vi "MultirunBuilderForNamedLocations2.vi"() -> ()   [LabVIEW 2015]
uses:
  MultirunBuilderSubVIs/RowTemplate.ctl
  Anemometry Sub Vis/Gen Trav/Spacing.ctl
  Anemometry Sub Vis/Controls/Multi_run_mode.ctl
  MultirunBuilderSubVIs/MRBRowTaskSelector.ctl
  Anemometry Sub Vis/File/Setup_Filetype.ctl
  Anemometry Sub Vis/Controls/Tunnel_Coordinates.ctl
  Anemometry Sub Vis/Globals/Meas_global.vi
  MultirunBuilderSubVIs/MRCMDFBGlobal.vi
  MultirunBuilderSubVIs/Set Speed Only.vi
  MultirunBuilderSubVIs/Wait (minutes).vi
  MultirunBuilderSubVIs/Single Measurement.vi
  MultirunBuilderSubVIs/Auto Calibrate.vi
  MultirunBuilderSubVIs/MoveTT.vi
panel:
  in  "Vert.Z-Locations 2":dbl[](array[numeric])=[12.7, 19.05, 25.4]
  in  "TaskArray":T3(array[cluster])=[{"Start X"=0.0, "Start Y"=0.0, "Start Z"=0.0, "End X"=0.0, "End Y"=0.0, "End Z"=0.0, "No. of pts."=0, "Spacing"=enum."Linear", "Filename"=path "M:/\\Projects\\8773\\Results\\Tunnel1\\AnemometerSurvey.xls", "Tunnel Speed"=7.64, "Averaging time (min)"=0.0, "Extra Commands"="", "Carrier_1 Q (l/min)"=0.0, "Carrier_2 Q (l/min)"=0.0, "Trace Gas Concentration (%)"=0.0, "Specific Arguments"="", "Comments"="Tunnel Warm Up", "Row No"=0, "Row Type Selector"=enum."Set Tunnel Speed Only", "Completion time"="", "Row Duration (mins)"=0.0, "No. of Valid pts."=0, "Meas Setup File"="Current_Setup.xls"}, {"Start X"=0.0, "Start Y"=0.0, "Start Z"=0.0, "End X"=0.0, "End Y"=0.0, "End Z"=0.0, "No. of pts."=0, "Spacing"=enum."Linear", "Filename"=path "M:/\\Projects\\8773\\Results\\Tunnel1\\AnemometerSurvey.xls", "Tunnel Speed"=0.0, "Averaging time (min)"=0.0, "Extra Commands"="", "Carrier_1 Q (l/min)"=0.0, "Carrier_2 Q (l/min)"=0.0, "Trace Gas Concentration (%)"=0.0, "Specific Arguments"="10.00", "Comments"="Tunnel Warm Up", "Row No"=0, "Row Type Selector"=enum."Wait (minutes)", "Completion time"="", "Row Duration (mins)"=0.0, "No. of Valid pts."=0, "Meas Setup File"="Current_Setup.xls"}, {"Start X"=-3390.0, "Start Y"=-113.0, "Start Z"=780.0, "End X"=-3390.0, "End Y"=-113.0, "End Z"=780.0, "No. of pts."=0, "Spacing"=enum."Linear", "Filename"=path "M:/\\Projects\\8773\\Results\\Tunnel1\\AnemometerSurvey.xls", "Tunnel Speed"=0.0, "Averaging time (min)"=1.0, "Extra Commands"="!Work in Tunnel Coordinates", "Carrier_1 Q (l/min)"=0.0, "Carrier_2 Q (l/min)"=0.0, "Trace Gas Concentration (%)"=0.0, "Specific Arguments"="", "Comments"="Zeroes", "Row No"=0, "Row Type Selector"=enum."Single Measurement", "Completion time"="", "Row Duration (mins)"=0.0, "No. of Valid pts."=0, "Meas Setup File"="Current_Setup.xls"}, {"Start X"=-3390.0, "Start Y"=-113.0, "Start Z"=780.0, "End X"=-3390.0, "End Y"=-113.0, "End Z"=780.0, "No. of pts."=0, "Spacing"=enum."Linear", "Filename"=path "M:/\\Projects\\8773\\Results\\Tunnel1\\AnemometerSurvey.xls", "Tunnel Speed"=7.64, "Averaging time (min)"=1.0, "Extra Commands"="!Work in Tunnel Coordinates", "Carrier_1 Q (l/min)"=0.0, "Carrier_2 Q (l/min)"=0.0, "Trace Gas Concentration (%)"=0.0, "Specific Arguments"="", "Comments"="CalCheck", "Row No"=0, "Row Type Selector"=enum."Single Measurement", "Completion time"="", "Row Duration (mins)"=0.0, "No. of Valid pts."=0, "Meas Setup File"="Current_Setup.xls"}, {"Start X"=0.0, "Start Y"=0.0, "Start Z"=780.0, "End X"=0.0, "End Y"=0.0, "End Z"=780.0, "No. of pts."=0, "Spacing"=enum."Linear", "Filename"=path "M:/\\Projects\\8773\\Results\\Tunnel1\\AnemometerSurvey.xls", "Tunnel Speed"=7.64, "Averaging time (min)"=1.0, "Extra Commands"="!Work in Tunnel Coordinates", "Carrier_1 Q (l/min)"=0.0, "Carrier_2 Q (l/min)"=0.0, "Trace Gas Concentration (%)"=0.0, "Specific Arguments"="", "Comments"="LocalCalCheck", "Row No"=0, "Row Type Selector"=enum."Single Measurement", "Completion time"="", "Row Duration (mins)"=0.0, "No. of Valid pts."=0, "Meas Setup File"="Current_Setup.xls"}, {"Start X"=0.0, "Start Y"=0.0, "Start Z"=0.0, "End X"=0.0, "End Y"=0.0, "End Z"=0.0, "No. of pts."=0, "Spacing"=enum."N/A", "Filename"=path "M:/\\Projects\\8773\\Results\\Tunnel1\\AnemometerSurvey.xls", "Tunnel Speed"=0.0, "Averaging time (min)"=0.0, "Extra Commands"="", "Carrier_1 Q (l/min)"=0.0, "Carrier_2 Q (l/min)"=0.0, "Trace Gas Concentration (%)"=0.0, "Specific Arguments"="MoveTT.vi;0", "Comments"="", "Row No"=0, "Row Type Selector"=enum."Run VI Named:", "Completion time"="", "Row Duration (mins)"=0.0, "No. of Valid pts."=0, "Meas Setup File"="Current_Setup.xls"}, {"Start X"=0.0, "Start Y"=0.0, "Start Z"=0.0, "End X"=0.0, "End Y"=0.0, "End Z"=0.0, "No. of pts."=0, "Spacing"=enum."Linear", "Filename"=path "M:/\\Projects\\8773\\Results\\Tunnel1\\AnemometerSurvey.xls", "Tunnel Speed"=0.0, "Averaging time (min)"=0.0, "Extra Commands"="", "Carrier_1 Q (l/min)"=0.0, "Carrier_2 Q (l/min)"=0.0, "Trace Gas Concentration (%)"=0.0, "Specific Arguments"="1440.00", "Comments"="", "Row No"=0, "Row Type Selector"=enum."Wait (minutes)", "Completion time"="", "Row Duration (mins)"=0.0, "No. of Valid pts."=0, "Meas Setup File"="Current_Setup.xls"}, {"Start X"=0.0, "Start Y"=0.0, "Start Z"=0.0, "End X"=0.0, "End Y"=0.0, "End Z"=0.0, "No. of pts."=0, "Spacing"=enum."Linear", "Filename"=path "M:/\\Projects\\8773\\Results\\Tunnel1\\AnemometerSurvey.xls", "Tunnel Speed"=0.0, "Averaging time (min)"=0.0, "Extra Commands"="-0.000", "Carrier_1 Q (l/min)"=0.0, "Carrier_2 Q (l/min)"=0.0, "Trace Gas Concentration (%)"=0.0, "Specific Arguments"="T1:Z:Corrections", "Comments"="", "Row No"=0, "Row Type Selector"=enum."Set ADAM Ch", "Completion time"="", "Row Duration (mins)"=0.0, "No. of Valid pts."=0, "Meas Setup File"="Current_Setup.xls"}, {"Start X"=-72.9, "Start Y"=-56.5, "Start Z"=12.7, "End X"=-72.9, "End Y"=-56.5, "End Z"=25.4, "No. of pts."=3, "Spacing"=enum."Specified", "Filename"=path "M:/\\Projects\\8773\\Results\\Tunnel1\\AnemometerSurvey.xls", "Tunnel Speed"=7.64, "Averaging time (min)"=1.0, "Extra Commands"="", "Carrier_1 Q (l/min)"=0.0, "Carrier_2 Q (l/min)"=0.0, "Trace Gas Concentration (%)"=0.0, "Specific Arguments"="Z= ;12.7;19.1;25.4\r", "Comments"="Anemo1", "Row No"=0, "Row Type Selector"=enum."Vertical Profile", "Completion time"="", "Row Duration (mins)"=0.0, "No. of Valid pts."=0, "Meas Setup File"="Current_Setup.xls"}, {"Start X"=0.0, "Start Y"=0.0, "Start Z"=0.0, "End X"=0.0, "End Y"=0.0, "End Z"=0.0, "No. of pts."=0, "Spacing"=enum."Linear", "Filename"=path "M:/\\Projects\\8773\\Results\\Tunnel1\\AnemometerSurvey.xls", "Tunnel Speed"=0.0, "Averaging time (min)"=0.0, "Extra Commands"="-0.000", "Carrier_1 Q (l/min)"=0.0, "Carrier_2 Q (l/min)"=0.0, "Trace Gas Concentration (%)"=0.0, "Specific Arguments"="T1:Z:Corrections", "Comments"="", "Row No"=0, "Row Type Selector"=enum."Set ADAM Ch", "Completion time"="", "Row Duration (mins)"=0.0, "No. of Valid pts."=0, "Meas Setup File"="Current_Setup.xls"}, {"Start X"=-458.4, "Start Y"=87.9, "Start Z"=25.6, "End X"=-458.4, "End Y"=87.9, "End Z"=38.3, "No. of pts."=3, "Spacing"=enum."Specified", "Filename"=path "M:/\\Projects\\8773\\Results\\Tunnel1\\AnemometerSurvey.xls", "Tunnel Speed"=7.64, "Averaging time (min)"=1.0, "Extra Commands"="", "Carrier_1 Q (l/min)"=0.0, "Carrier_2 Q (l/min)"=0.0, "Trace Gas Concentration (%)"=0.0, "Specific Arguments"="Z= ;25.6;32.0;38.3\r", "Comments"="Anemo2", "Row No"=0, "Row Type Selector"=enum."Vertical Profile", "Completion time"="", "Row Duration (mins)"=0.0, "No. of Valid pts."=0, "Meas Setup File"="Current_Setup.xls"}, {"Start X"=0.0, "Start Y"=0.0, "Start Z"=150.0, "End X"=0.0, "End Y"=0.0, "End Z"=150.0, "No. of pts."=0, "Spacing"=enum."Linear", "Filename"=path "M:/\\Projects\\8773\\Results\\Tunnel1\\AnemometerSurvey.xls", "Tunnel Speed"=0.0, "Averaging time (min)"=0.0, "Extra Commands"="!Work in Tunnel Coordinates", "Carrier_1 Q (l/min)"=0.0, "Carrier_2 Q (l/min)"=0.0, "Trace Gas Concentration (%)"=0.0, "Specific Arguments"="", "Comments"="", "Row No"=0, "Row Type Selector"=enum."Move Traverse Only", "Completion time"="", "Row Duration (mins)"=0.0, "No. of Valid pts."=0, "Meas Setup File"="Current_Setup.xls"}, {"Start X"=0.0, "Start Y"=0.0, "Start Z"=0.0, "End X"=0.0, "End Y"=0.0, "End Z"=0.0, "No. of pts."=0, "Spacing"=enum."Linear", "Filename"=path "M:/\\Projects\\8773\\Results\\Tunnel1\\AnemometerSurvey.xls", "Tunnel Speed"=0.0, "Averaging time (min)"=0.0, "Extra Commands"="", "Carrier_1 Q (l/min)"=0.0, "Carrier_2 Q (l/min)"=0.0, "Trace Gas Concentration (%)"=0.0, "Specific Arguments"="", "Comments"="Time to set ramps...", "Row No"=0, "Row Type Selector"=enum."Send Message", "Completion time"="", "Row Duration (mins)"=0.0, "No. of Valid pts."=0, "Meas Setup File"="Current_Setup.xls"}, {"Start X"=0.0, "Start Y"=0.0, "Start Z"=0.0, "End X"=0.0, "End Y"=0.0, "End Z"=0.0, "No. of pts."=0, "Spacing"=enum."Linear", "Filename"=path "", "Tunnel Speed"=0.0, "Averaging time (min)"=0.0, "Extra Commands"="", "Carrier_1 Q (l/min)"=0.0, "Carrier_2 Q (l/min)"=0.0, "Trace Gas Concentration (%)"=0.0, "Specific Arguments"="", "Comments"="", "Row No"=0, "Row Type Selector"=enum."Blank Row", "Completion time"="", "Row Duration (mins)"=0.0, "No. of Valid pts."=0, "Meas Setup File"=""}, {"Start X"=0.0, "Start Y"=0.0, "Start Z"=0.0, "End X"=0.0, "End Y"=0.0, "End Z"=0.0, "No. of pts."=0, "Spacing"=enum."N/A", "Filename"=path "M:/\\Projects\\8773\\Results\\Tunnel1\\AnemometerSurvey.xls", "Tunnel Speed"=0.0, "Averaging time (min)"=0.0, "Extra Commands"="", "Carrier_1 Q (l/min)"=0.0, "Carrier_2 Q (l/min)"=0.0, "Trace Gas Concentration (%)"=0.0, "Specific Arguments"="MoveTT.vi;20", "Comments"="", "Row No"=0, "Row Type Selector"=enum."Run VI Named:", "Completion time"="", "Row Duration (mins)"=0.0, "No. of Valid pts."=0, "Meas Setup File"="Current_Setup.xls"}, {"Start X"=0.0, "Start Y"=0.0, "Start Z"=0.0, "End X"=0.0, "End Y"=0.0, "End Z"=0.0, "No. of pts."=0, "Spacing"=enum."Linear", "Filename"=path "M:/\\Projects\\8773\\Results\\Tunnel1\\AnemometerSurvey.xls", "Tunnel Speed"=0.0, "Averaging time (min)"=0.0, "Extra Commands"="", "Carrier_1 Q (l/min)"=0.0, "Carrier_2 Q (l/min)"=0.0, "Trace Gas Concentration (%)"=0.0, "Specific Arguments"="1440.00", "Comments"="", "Row No"=0, "Row Type Selector"=enum."Wait (minutes)", "Completion time"="", "Row Duration (mins)"=0.0, "No. of Valid pts."=0, "Meas Setup File"="Current_Setup.xls"}, {"Start X"=0.0, "Start Y"=0.0, "Start Z"=0.0, "End X"=0.0, "End Y"=0.0, "End Z"=0.0, "No. of pts."=0, "Spacing"=enum."Linear", "Filename"=path "M:/\\Projects\\8773\\Results\\Tunnel1\\AnemometerSurvey.xls", "Tunnel Speed"=0.0, "Averaging time (min)"=0.0, "Extra Commands"="-0.500", "Carrier_1 Q (l/min)"=0.0, "Carrier_2 Q (l/min)"=0.0, "Trace Gas Concentration (%)"=0.0, "Specific Arguments"="T1:Z:Corrections", "Comments"="", "Row No"=0, "Row Type Selector"=enum."Set ADAM Ch", "Completion time"="", "Row Duration (mins)"=0.0, "No. of Valid pts."=0, "Meas Setup File"="Current_Setup.xls"}, {"Start X"=-72.9, "Start Y"=-56.5, "Start Z"=12.2, "End X"=-72.9, "End Y"=-56.5, "End Z"=24.9, "No. of pts."=3, "Spacing"=enum."Specified", "Filename"=path "M:/\\Projects\\8773\\Results\\Tunnel1\\AnemometerSurvey.xls", "Tunnel Speed"=7.64, "Averaging time (min)"=1.0, "Extra Commands"="", "Carrier_1 Q (l/min)"=0.0, "Carrier_2 Q (l/min)"=0.0, "Trace Gas Concentration (%)"=0.0, "Specific Arguments"="Z= ;12.2;18.6;24.9\r", "Comments"="Anemo1", "Row No"=0, "Row Type Selector"=enum."Vertical Profile", "Completion time"="", "Row Duration (mins)"=0.0, "No. of Valid pts."=0, "Meas Setup File"="Current_Setup.xls"}, {"Start X"=0.0, "Start Y"=0.0, "Start Z"=0.0, "End X"=0.0, "End Y"=0.0, "End Z"=0.0, "No. of pts."=0, "Spacing"=enum."Linear", "Filename"=path "M:/\\Projects\\8773\\Results\\Tunnel1\\AnemometerSurvey.xls", "Tunnel Speed"=0.0, "Averaging time (min)"=0.0, "Extra Commands"="-1.400", "Carrier_1 Q (l/min)"=0.0, "Carrier_2 Q (l/min)"=0.0, "Trace Gas Concentration (%)"=0.0, "Specific Arguments"="T1:Z:Corrections", "Comments"="", "Row No"=0, "Row Type Selector"=enum."Set ADAM Ch", "Completion time"="", "Row Duration (mins)"=0.0, "No. of Valid pts."=0, "Meas Setup File"="Current_Setup.xls"}, {"Start X"=-458.4, "Start Y"=87.9, "Start Z"=24.2, "End X"=-458.4, "End Y"=87.9, "End Z"=36.9, "No. of pts."=3, "Spacing"=enum."Specified", "Filename"=path "M:/\\Projects\\8773\\Results\\Tunnel1\\AnemometerSurvey.xls", "Tunnel Speed"=7.64, "Averaging time (min)"=1.0, "Extra Commands"="", "Carrier_1 Q (l/min)"=0.0, "Carrier_2 Q (l/min)"=0.0, "Trace Gas Concentration (%)"=0.0, "Specific Arguments"="Z= ;24.2;30.5;36.9\r", "Comments"="Anemo2", "Row No"=0, "Row Type Selector"=enum."Vertical Profile", "Completion time"="", "Row Duration (mins)"=0.0, "No. of Valid pts."=0, "Meas Setup File"="Current_Setup.xls"}, {"Start X"=0.0, "Start Y"=0.0, "Start Z"=150.0, "End X"=0.0, "End Y"=0.0, "End Z"=150.0, "No. of pts."=0, "Spacing"=enum."Linear", "Filename"=path "M:/\\Projects\\8773\\Results\\Tunnel1\\AnemometerSurvey.xls", "Tunnel Speed"=0.0, "Averaging time (min)"=0.0, "Extra Commands"="!Work in Tunnel Coordinates", "Carrier_1 Q (l/min)"=0.0, "Carrier_2 Q (l/min)"=0.0, "Trace Gas Concentration (%)"=0.0, "Specific Arguments"="", "Comments"="", "Row No"=0, "Row Type Selector"=enum."Move Traverse Only", "Completion time"="", "Row Duration (mins)"=0.0, "No. of Valid pts."=0, "Meas Setup File"="Current_Setup.xls"}, {"Start X"=0.0, "Start Y"=0.0, "Start Z"=0.0, "End X"=0.0, "End Y"=0.0, "End Z"=0.0, "No. of pts."=0, "Spacing"=enum."Linear", "Filename"=path "M:/\\Projects\\8773\\Results\\Tunnel1\\AnemometerSurvey.xls", "Tunnel Speed"=0.0, "Averaging time (min)"=0.0, "Extra Commands"="", "Carrier_1 Q (l/min)"=0.0, "Carrier_2 Q (l/min)"=0.0, "Trace Gas Concentration (%)"=0.0, "Specific Arguments"="", "Comments"="Time to set ramps...", "Row No"=0, "Row Type Selector"=enum."Send Message", "Completion time"="", "Row Duration (mins)"=0.0, "No. of Valid pts."=0, "Meas Setup File"="Current_Setup.xls"}, {"Start X"=0.0, "Start Y"=0.0, "Start Z"=0.0, "End X"=0.0, "End Y"=0.0, "End Z"=0.0, "No. of pts."=0, "Spacing"=enum."Linear", "Filename"=path "", "Tunnel Speed"=0.0, "Averaging time (min)"=0.0, "Extra Commands"="", "Carrier_1 Q (l/min)"=0.0, "Carrier_2 Q (l/min)"=0.0, "Trace Gas Concentration (%)"=0.0, "Specific Arguments"="", "Comments"="", "Row No"=0, "Row Type Selector"=enum."Blank Row", "Completion time"="", "Row Duration (mins)"=0.0, "No. of Valid pts."=0, "Meas Setup File"=""}, {"Start X"=0.0, "Start Y"=0.0, "Start Z"=0.0, "End X"=0.0, "End Y"=0.0, "End Z"=0.0, "No. of pts."=0, "Spacing"=enum."N/A", "Filename"=path "M:/\\Projects\\8773\\Results\\Tunnel1\\AnemometerSurvey.xls", "Tunnel Speed"=0.0, "Averaging time (min)"=0.0, "Extra Commands"="", "Carrier_1 Q (l/min)"=0.0, "Carrier_2 Q (l/min)"=0.0, "Trace Gas Concentration (%)"=0.0, "Specific Arguments"="MoveTT.vi;40", "Comments"="", "Row No"=0, "Row Type Selector"=enum."Run VI Named:", "Completion time"="", "Row Duration (mins)"=0.0, "No. of Valid pts."=0, "Meas Setup File"="Current_Setup.xls"}, {"Start X"=0.0, "Start Y"=0.0, "Start Z"=0.0, "End X"=0.0, "End Y"=0.0, "End Z"=0.0, "No. of pts."=0, "Spacing"=enum."Linear", "Filename"=path "M:/\\Projects\\8773\\Results\\Tunnel1\\AnemometerSurvey.xls", "Tunnel Speed"=0.0, "Averaging time (min)"=0.0, "Extra Commands"="", "Carrier_1 Q (l/min)"=0.0, "Carrier_2 Q (l/min)"=0.0, "Trace Gas Concentration (%)"=0.0, "Specific Arguments"="1440.00", "Comments"="", "Row No"=0, "Row Type Selector"=enum."Wait (minutes)", "Completion time"="", "Row Duration (mins)"=0.0, "No. of Valid pts."=0, "Meas Setup File"="Current_Setup.xls"}, {"Start X"=0.0, "Start Y"=0.0, "Start Z"=0.0, "End X"=0.0, "End Y"=0.0, "End Z"=0.0, "No. of pts."=0, "Spacing"=enum."Linear", "Filename"=path "M:/\\Projects\\8773\\Results\\Tunnel1\\AnemometerSurvey.xls", "Tunnel Speed"=0.0, "Averaging time (min)"=0.0, "Extra Commands"="-1.000", "Carrier_1 Q (l/min)"=0.0, "Carrier_2 Q (l/min)"=0.0, "Trace Gas Concentration (%)"=0.0, "Specific Arguments"="T1:Z:Corrections", "Comments"="", "Row No"=0, "Row Type Selector"=enum."Set ADAM Ch", "Completion time"="", "Row Duration (mins)"=0.0, "No. of Valid pts."=0, "Meas Setup File"="Current_Setup.xls"}, {"Start X"=-72.9, "Start Y"=-56.5, "Start Z"=11.7, "End X"=-72.9, "End Y"=-56.5, "End Z"=24.4, "No. of pts."=3, "Spacing"=enum."Specified", "Filename"=path "M:/\\Projects\\8773\\Results\\Tunnel1\\AnemometerSurvey.xls", "Tunnel Speed"=7.64, "Averaging time (min)"=1.0, "Extra Commands"="", "Carrier_1 Q (l/min)"=0.0, "Carrier_2 Q (l/min)"=0.0, "Trace Gas Concentration (%)"=0.0, "Specific Arguments"="Z= ;11.7;18.1;24.4\r", "Comments"="Anemo1", "Row No"=0, "Row Type Selector"=enum."Vertical Profile", "Completion time"="", "Row Duration (mins)"=0.0, "No. of Valid pts."=0, "Meas Setup File"="Current_Setup.xls"}, {"Start X"=0.0, "Start Y"=0.0, "Start Z"=0.0, "End X"=0.0, "End Y"=0.0, "End Z"=0.0, "No. of pts."=0, "Spacing"=enum."Linear", "Filename"=path "M:/\\Projects\\8773\\Results\\Tunnel1\\AnemometerSurvey.xls", "Tunnel Speed"=0.0, "Averaging time (min)"=0.0, "Extra Commands"="-3.100", "Carrier_1 Q (l/min)"=0.0, "Carrier_2 Q (l/min)"=0.0, "Trace Gas Concentration (%)"=0.0, "Specific Arguments"="T1:Z:Corrections", "Comments"="", "Row No"=0, "Row Type Selector"=enum."Set ADAM Ch", "Completion time"="", "Row Duration (mins)"=0.0, "No. of Valid pts."=0, "Meas Setup File"="Current_Setup.xls"}, {"Start X"=-458.4, "Start Y"=87.9, "Start Z"=22.5, "End X"=-458.4, "End Y"=87.9, "End Z"=35.2, "No. of pts."=3, "Spacing"=enum."Specified", "Filename"=path "M:/\\Projects\\8773\\Results\\Tunnel1\\AnemometerSurvey.xls", "Tunnel Speed"=7.64, "Averaging time (min)"=1.0, "Extra Commands"="", "Carrier_1 Q (l/min)"=0.0, "Carrier_2 Q (l/min)"=0.0, "Trace Gas Concentration (%)"=0.0, "Specific Arguments"="Z= ;22.5;28.8;35.2\r", "Comments"="Anemo2", "Row No"=0, "Row Type Selector"=enum."Vertical Profile", "Completion time"="", "Row Duration (mins)"=0.0, "No. of Valid pts."=0, "Meas Setup File"="Current_Setup.xls"}, {"Start X"=0.0, "Start Y"=0.0, "Start Z"=150.0, "End X"=0.0, "End Y"=0.0, "End Z"=150.0, "No. of pts."=0, "Spacing"=enum."Linear", "Filename"=path "M:/\\Projects\\8773\\Results\\Tunnel1\\AnemometerSurvey.xls", "Tunnel Speed"=0.0, "Averaging time (min)"=0.0, "Extra Commands"="!Work in Tunnel Coordinates", "Carrier_1 Q (l/min)"=0.0, "Carrier_2 Q (l/min)"=0.0, "Trace Gas Concentration (%)"=0.0, "Specific Arguments"="", "Comments"="", "Row No"=0, "Row Type Selector"=enum."Move Traverse Only", "Completion time"="", "Row Duration (mins)"=0.0, "No. of Valid pts."=0, "Meas Setup File"="Current_Setup.xls"}, {"Start X"=0.0, "Start Y"=0.0, "Start Z"=0.0, "End X"=0.0, "End Y"=0.0, "End Z"=0.0, "No. of pts."=0, "Spacing"=enum."Linear", "Filename"=path "M:/\\Projects\\8773\\Results\\Tunnel1\\AnemometerSurvey.xls", "Tunnel Speed"=0.0, "Averaging time (min)"=0.0, "Extra Commands"="", "Carrier_1 Q (l/min)"=0.0, "Carrier_2 Q (l/min)"=0.0, "Trace Gas Concentration (%)"=0.0, "Specific Arguments"="", "Comments"="Time to set ramps...", "Row No"=0, "Row Type Selector"=enum."Send Message", "Completion time"="", "Row Duration (mins)"=0.0, "No. of Valid pts."=0, "Meas Setup File"="Current_Setup.xls"}, {"Start X"=0.0, "Start Y"=0.0, "Start Z"=0.0, "End X"=0.0, "End Y"=0.0, "End Z"=0.0, "No. of pts."=0, "Spacing"=enum."Linear", "Filename"=path "", "Tunnel Speed"=0.0, "Averaging time (min)"=0.0, "Extra Commands"="", "Carrier_1 Q (l/min)"=0.0, "Carrier_2 Q (l/min)"=0.0, "Trace Gas Concentration (%)"=0.0, "Specific Arguments"="", "Comments"="", "Row No"=0, "Row Type Selector"=enum."Blank Row", "Completion time"="", "Row Duration (mins)"=0.0, "No. of Valid pts."=0, "Meas Setup File"=""}, {"Start X"=0.0, "Start Y"=0.0, "Start Z"=780.0, "End X"=0.0, "End Y"=0.0, "End Z"=780.0, "No. of pts."=0, "Spacing"=enum."Linear", "Filename"=path "M:/\\Projects\\8773\\Results\\Tunnel1\\AnemometerSurvey.xls", "Tunnel Speed"=7.64, "Averaging time (min)"=1.0, "Extra Commands"="!Work in Tunnel Coordinates", "Carrier_1 Q (l/min)"=0.0, "Carrier_2 Q (l/min)"=0.0, "Trace Gas Concentration (%)"=0.0, "Specific Arguments"="", "Comments"="LocalCalCheck", "Row No"=0, "Row Type Selector"=enum."Single Measurement", "Completion time"="", "Row Duration (mins)"=0.0, "No. of Valid pts."=0, "Meas Setup File"="Current_Setup.xls"}, {"Start X"=0.0, "Start Y"=0.0, "Start Z"=0.0, "End X"=0.0, "End Y"=0.0, "End Z"=0.0, "No. of pts."=0, "Spacing"=enum."N/A", "Filename"=path "M:/\\Projects\\8773\\Results\\Tunnel1\\AnemometerSurvey.xls", "Tunnel Speed"=0.0, "Averaging time (min)"=0.0, "Extra Commands"="", "Carrier_1 Q (l/min)"=0.0, "Carrier_2 Q (l/min)"=0.0, "Trace Gas Concentration (%)"=0.0, "Specific Arguments"="MoveTT.vi;60", "Comments"="", "Row No"=0, "Row Type Selector"=enum."Run VI Named:", "Completion time"="", "Row Duration (mins)"=0.0, "No. of Valid pts."=0, "Meas Setup File"="Current_Setup.xls"}, {"Start X"=0.0, "Start Y"=0.0, "Start Z"=0.0, "End X"=0.0, "End Y"=0.0, "End Z"=0.0, "No. of pts."=0, "Spacing"=enum."Linear", "Filename"=path "M:/\\Projects\\8773\\Results\\Tunnel1\\AnemometerSurvey.xls", "Tunnel Speed"=0.0, "Averaging time (min)"=0.0, "Extra Commands"="", "Carrier_1 Q (l/min)"=0.0, "Carrier_2 Q (l/min)"=0.0, "Trace Gas Concentration (%)"=0.0, "Specific Arguments"="1440.00", "Comments"="", "Row No"=0, "Row Type Selector"=enum."Wait (minutes)", "Completion time"="", "Row Duration (mins)"=0.0, "No. of Valid pts."=0, "Meas Setup File"="Current_Setup.xls"}, {"Start X"=0.0, "Start Y"=0.0, "Start Z"=0.0, "End X"=0.0, "End Y"=0.0, "End Z"=0.0, "No. of pts."=0, "Spacing"=enum."Linear", "Filename"=path "M:/\\Projects\\8773\\Results\\Tunnel1\\AnemometerSurvey.xls", "Tunnel Speed"=0.0, "Averaging time (min)"=0.0, "Extra Commands"="-0.500", "Carrier_1 Q (l/min)"=0.0, "Carrier_2 Q (l/min)"=0.0, "Trace Gas Concentration (%)"=0.0, "Specific Arguments"="T1:Z:Corrections", "Comments"="", "Row No"=0, "Row Type Selector"=enum."Set ADAM Ch", "Completion time"="", "Row Duration (mins)"=0.0, "No. of Valid pts."=0, "Meas Setup File"="Current_Setup.xls"}, {"Start X"=-72.9, "Start Y"=-56.5, "Start Z"=12.2, "End X"=-72.9, "End Y"=-56.5, "End Z"=24.9, "No. of pts."=3, "Spacing"=enum."Specified", "Filename"=path "M:/\\Projects\\8773\\Results\\Tunnel1\\AnemometerSurvey.xls", "Tunnel Speed"=7.64, "Averaging time (min)"=1.0, "Extra Commands"="", "Carrier_1 Q (l/min)"=0.0, "Carrier_2 Q (l/min)"=0.0, "Trace Gas Concentration (%)"=0.0, "Specific Arguments"="Z= ;12.2;18.6;24.9\r", "Comments"="Anemo1", "Row No"=0, "Row Type Selector"=enum."Vertical Profile", "Completion time"="", "Row Duration (mins)"=0.0, "No. of Valid pts."=0, "Meas Setup File"="Current_Setup.xls"}, {"Start X"=0.0, "Start Y"=0.0, "Start Z"=0.0, "End X"=0.0, "End Y"=0.0, "End Z"=0.0, "No. of pts."=0, "Spacing"=enum."Linear", "Filename"=path "M:/\\Projects\\8773\\Results\\Tunnel1\\AnemometerSurvey.xls", "Tunnel Speed"=0.0, "Averaging time (min)"=0.0, "Extra Commands"="-4.100", "Carrier_1 Q (l/min)"=0.0, "Carrier_2 Q (l/min)"=0.0, "Trace Gas Concentration (%)"=0.0, "Specific Arguments"="T1:Z:Corrections", "Comments"="", "Row No"=0, "Row Type Selector"=enum."Set ADAM Ch", "Completion time"="", "Row Duration (mins)"=0.0, "No. of Valid pts."=0, "Meas Setup File"="Current_Setup.xls"}, {"Start X"=-458.4, "Start Y"=87.9, "Start Z"=21.5, "End X"=-458.4, "End Y"=87.9, "End Z"=34.2, "No. of pts."=3, "Spacing"=enum."Specified", "Filename"=path "M:/\\Projects\\8773\\Results\\Tunnel1\\AnemometerSurvey.xls", "Tunnel Speed"=7.64, "Averaging time (min)"=1.0, "Extra Commands"="", "Carrier_1 Q (l/min)"=0.0, "Carrier_2 Q (l/min)"=0.0, "Trace Gas Concentration (%)"=0.0, "Specific Arguments"="Z= ;21.5;27.8;34.2\r", "Comments"="Anemo2", "Row No"=0, "Row Type Selector"=enum."Vertical Profile", "Completion time"="", "Row Duration (mins)"=0.0, "No. of Valid pts."=0, "Meas Setup File"="Current_Setup.xls"}, {"Start X"=0.0, "Start Y"=0.0, "Start Z"=150.0, "End X"=0.0, "End Y"=0.0, "End Z"=150.0, "No. of pts."=0, "Spacing"=enum."Linear", "Filename"=path "M:/\\Projects\\8773\\Results\\Tunnel1\\AnemometerSurvey.xls", "Tunnel Speed"=0.0, "Averaging time (min)"=0.0, "Extra Commands"="!Work in Tunnel Coordinates", "Carrier_1 Q (l/min)"=0.0, "Carrier_2 Q (l/min)"=0.0, "Trace Gas Concentration (%)"=0.0, "Specific Arguments"="", "Comments"="", "Row No"=0, "Row Type Selector"=enum."Move Traverse Only", "Completion time"="", "Row Duration (mins)"=0.0, "No. of Valid pts."=0, "Meas Setup File"="Current_Setup.xls"}, {"Start X"=0.0, "Start Y"=0.0, "Start Z"=0.0, "End X"=0.0, "End Y"=0.0, "End Z"=0.0, "No. of pts."=0, "Spacing"=enum."Linear", "Filename"=path "M:/\\Projects\\8773\\Results\\Tunnel1\\AnemometerSurvey.xls", "Tunnel Speed"=0.0, "Averaging time (min)"=0.0, "Extra Commands"="", "Carrier_1 Q (l/min)"=0.0, "Carrier_2 Q (l/min)"=0.0, "Trace Gas Concentration (%)"=0.0, "Specific Arguments"="", "Comments"="Time to set ramps...", "Row No"=0, "Row Type Selector"=enum."Send Message", "Completion time"="", "Row Duration (mins)"=0.0, "No. of Valid pts."=0, "Meas Setup File"="Current_Setup.xls"}, {"Start X"=0.0, "Start Y"=0.0, "Start Z"=0.0, "End X"=0.0, "End Y"=0.0, "End Z"=0.0, "No. of pts."=0, "Spacing"=enum."Linear", "Filename"=path "", "Tunnel Speed"=0.0, "Averaging time (min)"=0.0, "Extra Commands"="", "Carrier_1 Q (l/min)"=0.0, "Carrier_2 Q (l/min)"=0.0, "Trace Gas Concentration (%)"=0.0, "Specific Arguments"="", "Comments"="", "Row No"=0, "Row Type Selector"=enum."Blank Row", "Completion time"="", "Row Duration (mins)"=0.0, "No. of Valid pts."=0, "Meas Setup File"=""}, {"Start X"=0.0, "Start Y"=0.0, "Start Z"=0.0, "End X"=0.0, "End Y"=0.0, "End Z"=0.0, "No. of pts."=0, "Spacing"=enum."N/A", "Filename"=path "M:/\\Projects\\8773\\Results\\Tunnel1\\AnemometerSurvey.xls", "Tunnel Speed"=0.0, "Averaging time (min)"=0.0, "Extra Commands"="", "Carrier_1 Q (l/min)"=0.0, "Carrier_2 Q (l/min)"=0.0, "Trace Gas Concentration (%)"=0.0, "Specific Arguments"="MoveTT.vi;80", "Comments"="", "Row No"=0, "Row Type Selector"=enum."Run VI Named:", "Completion time"="", "Row Duration (mins)"=0.0, "No. of Valid pts."=0, "Meas Setup File"="Current_Setup.xls"}, {"Start X"=0.0, "Start Y"=0.0, "Start Z"=0.0, "End X"=0.0, "End Y"=0.0, "End Z"=0.0, "No. of pts."=0, "Spacing"=enum."Linear", "Filename"=path "M:/\\Projects\\8773\\Results\\Tunnel1\\AnemometerSurvey.xls", "Tunnel Speed"=0.0, "Averaging time (min)"=0.0, "Extra Commands"="", "Carrier_1 Q (l/min)"=0.0, "Carrier_2 Q (l/min)"=0.0, "Trace Gas Concentration (%)"=0.0, "Specific Arguments"="1440.00", "Comments"="", "Row No"=0, "Row Type Selector"=enum."Wait (minutes)", "Completion time"="", "Row Duration (mins)"=0.0, "No. of Valid pts."=0, "Meas Setup File"="Current_Setup.xls"}, {"Start X"=0.0, "Start Y"=0.0, "Start Z"=0.0, "End X"=0.0, "End Y"=0.0, "End Z"=0.0, "No. of pts."=0, "Spacing"=enum."Linear", "Filename"=path "M:/\\Projects\\8773\\Results\\Tunnel1\\AnemometerSurvey.xls", "Tunnel Speed"=0.0, "Averaging time (min)"=0.0, "Extra Commands"="-0.800", "Carrier_1 Q (l/min)"=0.0, "Carrier_2 Q (l/min)"=0.0, "Trace Gas Concentration (%)"=0.0, "Specific Arguments"="T1:Z:Corrections", "Comments"="", "Row No"=0, "Row Type Selector"=enum."Set ADAM Ch", "Completion time"="", "Row Duration (mins)"=0.0, "No. of Valid pts."=0, "Meas Setup File"="Current_Setup.xls"}, {"Start X"=-72.9, "Start Y"=-56.5, "Start Z"=11.9, "End X"=-72.9, "End Y"=-56.5, "End Z"=24.6, "No. of pts."=3, "Spacing"=enum."Specified", "Filename"=path "M:/\\Projects\\8773\\Results\\Tunnel1\\AnemometerSurvey.xls", "Tunnel Speed"=7.64, "Averaging time (min)"=1.0, "Extra Commands"="", "Carrier_1 Q (l/min)"=0.0, "Carrier_2 Q (l/min)"=0.0, "Trace Gas Concentration (%)"=0.0, "Specific Arguments"="Z= ;11.9;18.3;24.6\r", "Comments"="Anemo1", "Row No"=0, "Row Type Selector"=enum."Vertical Profile", "Completion time"="", "Row Duration (mins)"=0.0, "No. of Valid pts."=0, "Meas Setup File"="Current_Setup.xls"}, {"Start X"=0.0, "Start Y"=0.0, "Start Z"=0.0, "End X"=0.0, "End Y"=0.0, "End Z"=0.0, "No. of pts."=0, "Spacing"=enum."Linear", "Filename"=path "M:/\\Projects\\8773\\Results\\Tunnel1\\AnemometerSurvey.xls", "Tunnel Speed"=0.0, "Averaging time (min)"=0.0, "Extra Commands"="-4.900", "Carrier_1 Q (l/min)"=0.0, "Carrier_2 Q (l/min)"=0.0, "Trace Gas Concentration (%)"=0.0, "Specific Arguments"="T1:Z:Corrections", "Comments"="", "Row No"=0, "Row Type Selector"=enum."Set ADAM Ch", "Completion time"="", "Row Duration (mins)"=0.0, "No. of Valid pts."=0, "Meas Setup File"="Current_Setup.xls"}, {"Start X"=-458.4, "Start Y"=87.9, "Start Z"=20.7, "End X"=-458.4, "End Y"=87.9, "End Z"=33.4, "No. of pts."=3, "Spacing"=enum."Specified", "Filename"=path "M:/\\Projects\\8773\\Results\\Tunnel1\\AnemometerSurvey.xls", "Tunnel Speed"=7.64, "Averaging time (min)"=1.0, "Extra Commands"="", "Carrier_1 Q (l/min)"=0.0, "Carrier_2 Q (l/min)"=0.0, "Trace Gas Concentration (%)"=0.0, "Specific Arguments"="Z= ;20.7;27.0;33.4\r", "Comments"="Anemo2", "Row No"=0, "Row Type Selector"=enum."Vertical Profile", "Completion time"="", "Row Duration (mins)"=0.0, "No. of Valid pts."=0, "Meas Setup File"="Current_Setup.xls"}, {"Start X"=0.0, "Start Y"=0.0, "Start Z"=150.0, "End X"=0.0, "End Y"=0.0, "End Z"=150.0, "No. of pts."=0, "Spacing"=enum."Linear", "Filename"=path "M:/\\Projects\\8773\\Results\\Tunnel1\\AnemometerSurvey.xls", "Tunnel Speed"=0.0, "Averaging time (min)"=0.0, "Extra Commands"="!Work in Tunnel Coordinates", "Carrier_1 Q (l/min)"=0.0, "Carrier_2 Q (l/min)"=0.0, "Trace Gas Concentration (%)"=0.0, "Specific Arguments"="", "Comments"="", "Row No"=0, "Row Type Selector"=enum."Move Traverse Only", "Completion time"="", "Row Duration (mins)"=0.0, "No. of Valid pts."=0, "Meas Setup File"="Current_Setup.xls"}, {"Start X"=0.0, "Start Y"=0.0, "Start Z"=0.0, "End X"=0.0, "End Y"=0.0, "End Z"=0.0, "No. of pts."=0, "Spacing"=enum."Linear", "Filename"=path "M:/\\Projects\\8773\\Results\\Tunnel1\\AnemometerSurvey.xls", "Tunnel Speed"=0.0, "Averaging time (min)"=0.0, "Extra Commands"="", "Carrier_1 Q (l/min)"=0.0, "Carrier_2 Q (l/min)"=0.0, "Trace Gas Concentration (%)"=0.0, "Specific Arguments"="", "Comments"="Time to set ramps...", "Row No"=0, "Row Type Selector"=enum."Send Message", "Completion time"="", "Row Duration (mins)"=0.0, "No. of Valid pts."=0, "Meas Setup File"="Current_Setup.xls"}, {"Start X"=0.0, "Start Y"=0.0, "Start Z"=0.0, "End X"=0.0, "End Y"=0.0, "End Z"=0.0, "No. of pts."=0, "Spacing"=enum."Linear", "Filename"=path "", "Tunnel Speed"=0.0, "Averaging time (min)"=0.0, "Extra Commands"="", "Carrier_1 Q (l/min)"=0.0, "Carrier_2 Q (l/min)"=0.0, "Trace Gas Concentration (%)"=0.0, "Specific Arguments"="", "Comments"="", "Row No"=0, "Row Type Selector"=enum."Blank Row", "Completion time"="", "Row Duration (mins)"=0.0, "No. of Valid pts."=0, "Meas Setup File"=""}, {"Start X"=0.0, "Start Y"=0.0, "Start Z"=0.0, "End X"=0.0, "End Y"=0.0, "End Z"=0.0, "No. of pts."=0, "Spacing"=enum."N/A", "Filename"=path "M:/\\Projects\\8773\\Results\\Tunnel1\\AnemometerSurvey.xls", "Tunnel Speed"=0.0, "Averaging time (min)"=0.0, "Extra Commands"="", "Carrier_1 Q (l/min)"=0.0, "Carrier_2 Q (l/min)"=0.0, "Trace Gas Concentration (%)"=0.0, "Specific Arguments"="MoveTT.vi;100", "Comments"="", "Row No"=0, "Row Type Selector"=enum."Run VI Named:", "Completion time"="", "Row Duration (mins)"=0.0, "No. of Valid pts."=0, "Meas Setup File"="Current_Setup.xls"}, {"Start X"=0.0, "Start Y"=0.0, "Start Z"=0.0, "End X"=0.0, "End Y"=0.0, "End Z"=0.0, "No. of pts."=0, "Spacing"=enum."Linear", "Filename"=path "M:/\\Projects\\8773\\Results\\Tunnel1\\AnemometerSurvey.xls", "Tunnel Speed"=0.0, "Averaging time (min)"=0.0, "Extra Commands"="", "Carrier_1 Q (l/min)"=0.0, "Carrier_2 Q (l/min)"=0.0, "Trace Gas Concentration (%)"=0.0, "Specific Arguments"="1440.00", "Comments"="", "Row No"=0, "Row Type Selector"=enum."Wait (minutes)", "Completion time"="", "Row Duration (mins)"=0.0, "No. of Valid pts."=0, "Meas Setup File"="Current_Setup.xls"}, {"Start X"=0.0, "Start Y"=0.0, "Start Z"=0.0, "End X"=0.0, "End Y"=0.0, "End Z"=0.0, "No. of pts."=0, "Spacing"=enum."Linear", "Filename"=path "M:/\\Projects\\8773\\Results\\Tunnel1\\AnemometerSurvey.xls", "Tunnel Speed"=0.0, "Averaging time (min)"=0.0, "Extra Commands"="-0.900", "Carrier_1 Q (l/min)"=0.0, "Carrier_2 Q (l/min)"=0.0, "Trace Gas Concentration (%)"=0.0, "Specific Arguments"="T1:Z:Corrections", "Comments"="", "Row No"=0, "Row Type Selector"=enum."Set ADAM Ch", "Completion time"="", "Row Duration (mins)"=0.0, "No. of Valid pts."=0, "Meas Setup File"="Current_Setup.xls"}, {"Start X"=-72.9, "Start Y"=-56.5, "Start Z"=11.8, "End X"=-72.9, "End Y"=-56.5, "End Z"=24.5, "No. of pts."=3, "Spacing"=enum."Specified", "Filename"=path "M:/\\Projects\\8773\\Results\\Tunnel1\\AnemometerSurvey.xls", "Tunnel Speed"=7.64, "Averaging time (min)"=1.0, "Extra Commands"="", "Carrier_1 Q (l/min)"=0.0, "Carrier_2 Q (l/min)"=0.0, "Trace Gas Concentration (%)"=0.0, "Specific Arguments"="Z= ;11.8;18.2;24.5\r", "Comments"="Anemo1", "Row No"=0, "Row Type Selector"=enum."Vertical Profile", "Completion time"="", "Row Duration (mins)"=0.0, "No. of Valid pts."=0, "Meas Setup File"="Current_Setup.xls"}, {"Start X"=0.0, "Start Y"=0.0, "Start Z"=0.0, "End X"=0.0, "End Y"=0.0, "End Z"=0.0, "No. of pts."=0, "Spacing"=enum."Linear", "Filename"=path "M:/\\Projects\\8773\\Results\\Tunnel1\\AnemometerSurvey.xls", "Tunnel Speed"=0.0, "Averaging time (min)"=0.0, "Extra Commands"="-5.600", "Carrier_1 Q (l/min)"=0.0, "Carrier_2 Q (l/min)"=0.0, "Trace Gas Concentration (%)"=0.0, "Specific Arguments"="T1:Z:Corrections", "Comments"="", "Row No"=0, "Row Type Selector"=enum."Set ADAM Ch", "Completion time"="", "Row Duration (mins)"=0.0, "No. of Valid pts."=0, "Meas Setup File"="Current_Setup.xls"}, {"Start X"=-458.4, "Start Y"=87.9, "Start Z"=20.0, "End X"=-458.4, "End Y"=87.9, "End Z"=32.7, "No. of pts."=3, "Spacing"=enum."Specified", "Filename"=path "M:/\\Projects\\8773\\Results\\Tunnel1\\AnemometerSurvey.xls", "Tunnel Speed"=7.64, "Averaging time (min)"=1.0, "Extra Commands"="", "Carrier_1 Q (l/min)"=0.0, "Carrier_2 Q (l/min)"=0.0, "Trace Gas Concentration (%)"=0.0, "Specific Arguments"="Z= ;20.0;26.3;32.7\r", "Comments"="Anemo2", "Row No"=0, "Row Type Selector"=enum."Vertical Profile", "Completion time"="", "Row Duration (mins)"=0.0, "No. of Valid pts."=0, "Meas Setup File"="Current_Setup.xls"}, {"Start X"=0.0, "Start Y"=0.0, "Start Z"=150.0, "End X"=0.0, "End Y"=0.0, "End Z"=150.0, "No. of pts."=0, "Spacing"=enum."Linear", "Filename"=path "M:/\\Projects\\8773\\Results\\Tunnel1\\AnemometerSurvey.xls", "Tunnel Speed"=0.0, "Averaging time (min)"=0.0, "Extra Commands"="!Work in Tunnel Coordinates", "Carrier_1 Q (l/min)"=0.0, "Carrier_2 Q (l/min)"=0.0, "Trace Gas Concentration (%)"=0.0, "Specific Arguments"="", "Comments"="", "Row No"=0, "Row Type Selector"=enum."Move Traverse Only", "Completion time"="", "Row Duration (mins)"=0.0, "No. of Valid pts."=0, "Meas Setup File"="Current_Setup.xls"}, {"Start X"=0.0, "Start Y"=0.0, "Start Z"=0.0, "End X"=0.0, "End Y"=0.0, "End Z"=0.0, "No. of pts."=0, "Spacing"=enum."Linear", "Filename"=path "M:/\\Projects\\8773\\Results\\Tunnel1\\AnemometerSurvey.xls", "Tunnel Speed"=0.0, "Averaging time (min)"=0.0, "Extra Commands"="", "Carrier_1 Q (l/min)"=0.0, "Carrier_2 Q (l/min)"=0.0, "Trace Gas Concentration (%)"=0.0, "Specific Arguments"="", "Comments"="Time to set ramps...", "Row No"=0, "Row Type Selector"=enum."Send Message", "Completion time"="", "Row Duration (mins)"=0.0, "No. of Valid pts."=0, "Meas Setup File"="Current_Setup.xls"}, {"Start X"=0.0, "Start Y"=0.0, "Start Z"=0.0, "End X"=0.0, "End Y"=0.0, "End Z"=0.0, "No. of pts."=0, "Spacing"=enum."Linear", "Filename"=path "", "Tunnel Speed"=0.0, "Averaging time (min)"=0.0, "Extra Commands"="", "Carrier_1 Q (l/min)"=0.0, "Carrier_2 Q (l/min)"=0.0, "Trace Gas Concentration (%)"=0.0, "Specific Arguments"="", "Comments"="", "Row No"=0, "Row Type Selector"=enum."Blank Row", "Completion time"="", "Row Duration (mins)"=0.0, "No. of Valid pts."=0, "Meas Setup File"=""}, {"Start X"=-3390.0, "Start Y"=-113.0, "Start Z"=780.0, "End X"=-3390.0, "End Y"=-113.0, "End Z"=780.0, "No. of pts."=0, "Spacing"=enum."Linear", "Filename"=path "M:/\\Projects\\8773\\Results\\Tunnel1\\AnemometerSurvey.xls", "Tunnel Speed"=0.0, "Averaging time (min)"=1.0, "Extra Commands"="!Work in Tunnel Coordinates", "Carrier_1 Q (l/min)"=0.0, "Carrier_2 Q (l/min)"=0.0, "Trace Gas Concentration (%)"=0.0, "Specific Arguments"="", "Comments"="Zeroes", "Row No"=0, "Row Type Selector"=enum."Single Measurement", "Completion time"="", "Row Duration (mins)"=0.0, "No. of Valid pts."=0, "Meas Setup File"="Current_Setup.xls"}, {"Start X"=-3390.0, "Start Y"=-113.0, "Start Z"=780.0, "End X"=-3390.0, "End Y"=-113.0, "End Z"=780.0, "No. of pts."=0, "Spacing"=enum."Linear", "Filename"=path "M:/\\Projects\\8773\\Results\\Tunnel1\\AnemometerSurvey.xls", "Tunnel Speed"=7.64, "Averaging time (min)"=1.0, "Extra Commands"="!Work in Tunnel Coordinates", "Carrier_1 Q (l/min)"=0.0, "Carrier_2 Q (l/min)"=0.0, "Trace Gas Concentration (%)"=0.0, "Specific Arguments"="", "Comments"="CalCheck", "Row No"=0, "Row Type Selector"=enum."Single Measurement", "Completion time"="", "Row Duration (mins)"=0.0, "No. of Valid pts."=0, "Meas Setup File"="Current_Setup.xls"}, {"Start X"=0.0, "Start Y"=0.0, "Start Z"=780.0, "End X"=0.0, "End Y"=0.0, "End Z"=780.0, "No. of pts."=0, "Spacing"=enum."Linear", "Filename"=path "M:/\\Projects\\8773\\Results\\Tunnel1\\AnemometerSurvey.xls", "Tunnel Speed"=7.64, "Averaging time (min)"=1.0, "Extra Commands"="!Work in Tunnel Coordinates", "Carrier_1 Q (l/min)"=0.0, "Carrier_2 Q (l/min)"=0.0, "Trace Gas Concentration (%)"=0.0, "Specific Arguments"="", "Comments"="LocalCalCheck", "Row No"=0, "Row Type Selector"=enum."Single Measurement", "Completion time"="", "Row Duration (mins)"=0.0, "No. of Valid pts."=0, "Meas Setup File"="Current_Setup.xls"}, {"Start X"=0.0, "Start Y"=0.0, "Start Z"=0.0, "End X"=0.0, "End Y"=0.0, "End Z"=0.0, "No. of pts."=0, "Spacing"=enum."N/A", "Filename"=path "M:/\\Projects\\8773\\Results\\Tunnel1\\AnemometerSurvey.xls", "Tunnel Speed"=0.0, "Averaging time (min)"=0.0, "Extra Commands"="", "Carrier_1 Q (l/min)"=0.0, "Carrier_2 Q (l/min)"=0.0, "Trace Gas Concentration (%)"=0.0, "Specific Arguments"="MoveTT.vi;120", "Comments"="", "Row No"=0, "Row Type Selector"=enum."Run VI Named:", "Completion time"="", "Row Duration (mins)"=0.0, "No. of Valid pts."=0, "Meas Setup File"="Current_Setup.xls"}, {"Start X"=0.0, "Start Y"=0.0, "Start Z"=0.0, "End X"=0.0, "End Y"=0.0, "End Z"=0.0, "No. of pts."=0, "Spacing"=enum."Linear", "Filename"=path "M:/\\Projects\\8773\\Results\\Tunnel1\\AnemometerSurvey.xls", "Tunnel Speed"=0.0, "Averaging time (min)"=0.0, "Extra Commands"="", "Carrier_1 Q (l/min)"=0.0, "Carrier_2 Q (l/min)"=0.0, "Trace Gas Concentration (%)"=0.0, "Specific Arguments"="1440.00", "Comments"="", "Row No"=0, "Row Type Selector"=enum."Wait (minutes)", "Completion time"="", "Row Duration (mins)"=0.0, "No. of Valid pts."=0, "Meas Setup File"="Current_Setup.xls"}, {"Start X"=0.0, "Start Y"=0.0, "Start Z"=0.0, "End X"=0.0, "End Y"=0.0, "End Z"=0.0, "No. of pts."=0, "Spacing"=enum."Linear", "Filename"=path "M:/\\Projects\\8773\\Results\\Tunnel1\\AnemometerSurvey.xls", "Tunnel Speed"=0.0, "Averaging time (min)"=0.0, "Extra Commands"="-0.400", "Carrier_1 Q (l/min)"=0.0, "Carrier_2 Q (l/min)"=0.0, "Trace Gas Concentration (%)"=0.0, "Specific Arguments"="T1:Z:Corrections", "Comments"="", "Row No"=0, "Row Type Selector"=enum."Set ADAM Ch", "Completion time"="", "Row Duration (mins)"=0.0, "No. of Valid pts."=0, "Meas Setup File"="Current_Setup.xls"}, {"Start X"=-72.9, "Start Y"=-56.5, "Start Z"=12.3, "End X"=-72.9, "End Y"=-56.5, "End Z"=25.0, "No. of pts."=3, "Spacing"=enum."Specified", "Filename"=path "M:/\\Projects\\8773\\Results\\Tunnel1\\AnemometerSurvey.xls", "Tunnel Speed"=7.64, "Averaging time (min)"=1.0, "Extra Commands"="", "Carrier_1 Q (l/min)"=0.0, "Carrier_2 Q (l/min)"=0.0, "Trace Gas Concentration (%)"=0.0, "Specific Arguments"="Z= ;12.3;18.7;25.0\r", "Comments"="Anemo1", "Row No"=0, "Row Type Selector"=enum."Vertical Profile", "Completion time"="", "Row Duration (mins)"=0.0, "No. of Valid pts."=0, "Meas Setup File"="Current_Setup.xls"}, {"Start X"=0.0, "Start Y"=0.0, "Start Z"=0.0, "End X"=0.0, "End Y"=0.0, "End Z"=0.0, "No. of pts."=0, "Spacing"=enum."Linear", "Filename"=path "M:/\\Projects\\8773\\Results\\Tunnel1\\AnemometerSurvey.xls", "Tunnel Speed"=0.0, "Averaging time (min)"=0.0, "Extra Commands"="-5.500", "Carrier_1 Q (l/min)"=0.0, "Carrier_2 Q (l/min)"=0.0, "Trace Gas Concentration (%)"=0.0, "Specific Arguments"="T1:Z:Corrections", "Comments"="", "Row No"=0, "Row Type Selector"=enum."Set ADAM Ch", "Completion time"="", "Row Duration (mins)"=0.0, "No. of Valid pts."=0, "Meas Setup File"="Current_Setup.xls"}, {"Start X"=-458.4, "Start Y"=87.9, "Start Z"=20.1, "End X"=-458.4, "End Y"=87.9, "End Z"=32.8, "No. of pts."=3, "Spacing"=enum."Specified", "Filename"=path "M:/\\Projects\\8773\\Results\\Tunnel1\\AnemometerSurvey.xls", "Tunnel Speed"=7.64, "Averaging time (min)"=1.0, "Extra Commands"="", "Carrier_1 Q (l/min)"=0.0, "Carrier_2 Q (l/min)"=0.0, "Trace Gas Concentration (%)"=0.0, "Specific Arguments"="Z= ;20.1;26.5;32.8\r", "Comments"="Anemo2", "Row No"=0, "Row Type Selector"=enum."Vertical Profile", "Completion time"="", "Row Duration (mins)"=0.0, "No. of Valid pts."=0, "Meas Setup File"="Current_Setup.xls"}, {"Start X"=0.0, "Start Y"=0.0, "Start Z"=150.0, "End X"=0.0, "End Y"=0.0, "End Z"=150.0, "No. of pts."=0, "Spacing"=enum."Linear", "Filename"=path "M:/\\Projects\\8773\\Results\\Tunnel1\\AnemometerSurvey.xls", "Tunnel Speed"=0.0, "Averaging time (min)"=0.0, "Extra Commands"="!Work in Tunnel Coordinates", "Carrier_1 Q (l/min)"=0.0, "Carrier_2 Q (l/min)"=0.0, "Trace Gas Concentration (%)"=0.0, "Specific Arguments"="", "Comments"="", "Row No"=0, "Row Type Selector"=enum."Move Traverse Only", "Completion time"="", "Row Duration (mins)"=0.0, "No. of Valid pts."=0, "Meas Setup File"="Current_Setup.xls"}, {"Start X"=0.0, "Start Y"=0.0, "Start Z"=0.0, "End X"=0.0, "End Y"=0.0, "End Z"=0.0, "No. of pts."=0, "Spacing"=enum."Linear", "Filename"=path "M:/\\Projects\\8773\\Results\\Tunnel1\\AnemometerSurvey.xls", "Tunnel Speed"=0.0, "Averaging time (min)"=0.0, "Extra Commands"="", "Carrier_1 Q (l/min)"=0.0, "Carrier_2 Q (l/min)"=0.0, "Trace Gas Concentration (%)"=0.0, "Specific Arguments"="", "Comments"="Time to set ramps...", "Row No"=0, "Row Type Selector"=enum."Send Message", "Completion time"="", "Row Duration (mins)"=0.0, "No. of Valid pts."=0, "Meas Setup File"="Current_Setup.xls"}, {"Start X"=0.0, "Start Y"=0.0, "Start Z"=0.0, "End X"=0.0, "End Y"=0.0, "End Z"=0.0, "No. of pts."=0, "Spacing"=enum."Linear", "Filename"=path "", "Tunnel Speed"=0.0, "Averaging time (min)"=0.0, "Extra Commands"="", "Carrier_1 Q (l/min)"=0.0, "Carrier_2 Q (l/min)"=0.0, "Trace Gas Concentration (%)"=0.0, "Specific Arguments"="", "Comments"="", "Row No"=0, "Row Type Selector"=enum."Blank Row", "Completion time"="", "Row Duration (mins)"=0.0, "No. of Valid pts."=0, "Meas Setup File"=""}, {"Start X"=0.0, "Start Y"=0.0, "Start Z"=0.0, "End X"=0.0, "End Y"=0.0, "End Z"=0.0, "No. of pts."=0, "Spacing"=enum."N/A", "Filename"=path "M:/\\Projects\\8773\\Results\\Tunnel1\\AnemometerSurvey.xls", "Tunnel Speed"=0.0, "Averaging time (min)"=0.0, "Extra Commands"="", "Carrier_1 Q (l/min)"=0.0, "Carrier_2 Q (l/min)"=0.0, "Trace Gas Concentration (%)"=0.0, "Specific Arguments"="MoveTT.vi;140", "Comments"="", "Row No"=0, "Row Type Selector"=enum."Run VI Named:", "Completion time"="", "Row Duration (mins)"=0.0, "No. of Valid pts."=0, "Meas Setup File"="Current_Setup.xls"}, {"Start X"=0.0, "Start Y"=0.0, "Start Z"=0.0, "End X"=0.0, "End Y"=0.0, "End Z"=0.0, "No. of pts."=0, "Spacing"=enum."Linear", "Filename"=path "M:/\\Projects\\8773\\Results\\Tunnel1\\AnemometerSurvey.xls", "Tunnel Speed"=0.0, "Averaging time (min)"=0.0, "Extra Commands"="", "Carrier_1 Q (l/min)"=0.0, "Carrier_2 Q (l/min)"=0.0, "Trace Gas Concentration (%)"=0.0, "Specific Arguments"="1440.00", "Comments"="", "Row No"=0, "Row Type Selector"=enum."Wait (minutes)", "Completion time"="", "Row Duration (mins)"=0.0, "No. of Valid pts."=0, "Meas Setup File"="Current_Setup.xls"}, {"Start X"=0.0, "Start Y"=0.0, "Start Z"=0.0, "End X"=0.0, "End Y"=0.0, "End Z"=0.0, "No. of pts."=0, "Spacing"=enum."Linear", "Filename"=path "M:/\\Projects\\8773\\Results\\Tunnel1\\AnemometerSurvey.xls", "Tunnel Speed"=0.0, "Averaging time (min)"=0.0, "Extra Commands"="0.100", "Carrier_1 Q (l/min)"=0.0, "Carrier_2 Q (l/min)"=0.0, "Trace Gas Concentration (%)"=0.0, "Specific Arguments"="T1:Z:Corrections", "Comments"="", "Row No"=0, "Row Type Selector"=enum."Set ADAM Ch", "Completion time"="", "Row Duration (mins)"=0.0, "No. of Valid pts."=0, "Meas Setup File"="Current_Setup.xls"}, {"Start X"=-72.9, "Start Y"=-56.5, "Start Z"=12.8, "End X"=-72.9, "End Y"=-56.5, "End Z"=25.5, "No. of pts."=3, "Spacing"=enum."Specified", "Filename"=path "M:/\\Projects\\8773\\Results\\Tunnel1\\AnemometerSurvey.xls", "Tunnel Speed"=7.64, "Averaging time (min)"=1.0, "Extra Commands"="", "Carrier_1 Q (l/min)"=0.0, "Carrier_2 Q (l/min)"=0.0, "Trace Gas Concentration (%)"=0.0, "Specific Arguments"="Z= ;12.8;19.2;25.5\r", "Comments"="Anemo1", "Row No"=0, "Row Type Selector"=enum."Vertical Profile", "Completion time"="", "Row Duration (mins)"=0.0, "No. of Valid pts."=0, "Meas Setup File"="Current_Setup.xls"}, {"Start X"=0.0, "Start Y"=0.0, "Start Z"=0.0, "End X"=0.0, "End Y"=0.0, "End Z"=0.0, "No. of pts."=0, "Spacing"=enum."Linear", "Filename"=path "M:/\\Projects\\8773\\Results\\Tunnel1\\AnemometerSurvey.xls", "Tunnel Speed"=0.0, "Averaging time (min)"=0.0, "Extra Commands"="-5.100", "Carrier_1 Q (l/min)"=0.0, "Carrier_2 Q (l/min)"=0.0, "Trace Gas Concentration (%)"=0.0, "Specific Arguments"="T1:Z:Corrections", "Comments"="", "Row No"=0, "Row Type Selector"=enum."Set ADAM Ch", "Completion time"="", "Row Duration (mins)"=0.0, "No. of Valid pts."=0, "Meas Setup File"="Current_Setup.xls"}, {"Start X"=-458.4, "Start Y"=87.9, "Start Z"=20.5, "End X"=-458.4, "End Y"=87.9, "End Z"=33.2, "No. of pts."=3, "Spacing"=enum."Specified", "Filename"=path "M:/\\Projects\\8773\\Results\\Tunnel1\\AnemometerSurvey.xls", "Tunnel Speed"=7.64, "Averaging time (min)"=1.0, "Extra Commands"="", "Carrier_1 Q (l/min)"=0.0, "Carrier_2 Q (l/min)"=0.0, "Trace Gas Concentration (%)"=0.0, "Specific Arguments"="Z= ;20.5;26.8;33.2\r", "Comments"="Anemo2", "Row No"=0, "Row Type Selector"=enum."Vertical Profile", "Completion time"="", "Row Duration (mins)"=0.0, "No. of Valid pts."=0, "Meas Setup File"="Current_Setup.xls"}, {"Start X"=0.0, "Start Y"=0.0, "Start Z"=150.0, "End X"=0.0, "End Y"=0.0, "End Z"=150.0, "No. of pts."=0, "Spacing"=enum."Linear", "Filename"=path "M:/\\Projects\\8773\\Results\\Tunnel1\\AnemometerSurvey.xls", "Tunnel Speed"=0.0, "Averaging time (min)"=0.0, "Extra Commands"="!Work in Tunnel Coordinates", "Carrier_1 Q (l/min)"=0.0, "Carrier_2 Q (l/min)"=0.0, "Trace Gas Concentration (%)"=0.0, "Specific Arguments"="", "Comments"="", "Row No"=0, "Row Type Selector"=enum."Move Traverse Only", "Completion time"="", "Row Duration (mins)"=0.0, "No. of Valid pts."=0, "Meas Setup File"="Current_Setup.xls"}, {"Start X"=0.0, "Start Y"=0.0, "Start Z"=0.0, "End X"=0.0, "End Y"=0.0, "End Z"=0.0, "No. of pts."=0, "Spacing"=enum."Linear", "Filename"=path "M:/\\Projects\\8773\\Results\\Tunnel1\\AnemometerSurvey.xls", "Tunnel Speed"=0.0, "Averaging time (min)"=0.0, "Extra Commands"="", "Carrier_1 Q (l/min)"=0.0, "Carrier_2 Q (l/min)"=0.0, "Trace Gas Concentration (%)"=0.0, "Specific Arguments"="", "Comments"="Time to set ramps...", "Row No"=0, "Row Type Selector"=enum."Send Message", "Completion time"="", "Row Duration (mins)"=0.0, "No. of Valid pts."=0, "Meas Setup File"="Current_Setup.xls"}, {"Start X"=0.0, "Start Y"=0.0, "Start Z"=0.0, "End X"=0.0, "End Y"=0.0, "End Z"=0.0, "No. of pts."=0, "Spacing"=enum."Linear", "Filename"=path "", "Tunnel Speed"=0.0, "Averaging time (min)"=0.0, "Extra Commands"="", "Carrier_1 Q (l/min)"=0.0, "Carrier_2 Q (l/min)"=0.0, "Trace Gas Concentration (%)"=0.0, "Specific Arguments"="", "Comments"="", "Row No"=0, "Row Type Selector"=enum."Blank Row", "Completion time"="", "Row Duration (mins)"=0.0, "No. of Valid pts."=0, "Meas Setup File"=""}, {"Start X"=0.0, "Start Y"=0.0, "Start Z"=0.0, "End X"=0.0, "End Y"=0.0, "End Z"=0.0, "No. of pts."=0, "Spacing"=enum."N/A", "Filename"=path "M:/\\Projects\\8773\\Results\\Tunnel1\\AnemometerSurvey.xls", "Tunnel Speed"=0.0, "Averaging time (min)"=0.0, "Extra Commands"="", "Carrier_1 Q (l/min)"=0.0, "Carrier_2 Q (l/min)"=0.0, "Trace Gas Concentration (%)"=0.0, "Specific Arguments"="MoveTT.vi;160", "Comments"="", "Row No"=0, "Row Type Selector"=enum."Run VI Named:", "Completion time"="", "Row Duration (mins)"=0.0, "No. of Valid pts."=0, "Meas Setup File"="Current_Setup.xls"}, {"Start X"=0.0, "Start Y"=0.0, "Start Z"=0.0, "End X"=0.0, "End Y"=0.0, "End Z"=0.0, "No. of pts."=0, "Spacing"=enum."Linear", "Filename"=path "M:/\\Projects\\8773\\Results\\Tunnel1\\AnemometerSurvey.xls", "Tunnel Speed"=0.0, "Averaging time (min)"=0.0, "Extra Commands"="", "Carrier_1 Q (l/min)"=0.0, "Carrier_2 Q (l/min)"=0.0, "Trace Gas Concentration (%)"=0.0, "Specific Arguments"="1440.00", "Comments"="", "Row No"=0, "Row Type Selector"=enum."Wait (minutes)", "Completion time"="", "Row Duration (mins)"=0.0, "No. of Valid pts."=0, "Meas Setup File"="Current_Setup.xls"}, {"Start X"=0.0, "Start Y"=0.0, "Start Z"=0.0, "End X"=0.0, "End Y"=0.0, "End Z"=0.0, "No. of pts."=0, "Spacing"=enum."Linear", "Filename"=path "M:/\\Projects\\8773\\Results\\Tunnel1\\AnemometerSurvey.xls", "Tunnel Speed"=0.0, "Averaging time (min)"=0.0, "Extra Commands"="0.100", "Carrier_1 Q (l/min)"=0.0, "Carrier_2 Q (l/min)"=0.0, "Trace Gas Concentration (%)"=0.0, "Specific Arguments"="T1:Z:Corrections", "Comments"="", "Row No"=0, "Row Type Selector"=enum."Set ADAM Ch", "Completion time"="", "Row Duration (mins)"=0.0, "No. of Valid pts."=0, "Meas Setup File"="Current_Setup.xls"}, {"Start X"=-72.9, "Start Y"=-56.5, "Start Z"=12.8, "End X"=-72.9, "End Y"=-56.5, "End Z"=25.5, "No. of pts."=3, "Spacing"=enum."Specified", "Filename"=path "M:/\\Projects\\8773\\Results\\Tunnel1\\AnemometerSurvey.xls", "Tunnel Speed"=7.64, "Averaging time (min)"=1.0, "Extra Commands"="", "Carrier_1 Q (l/min)"=0.0, "Carrier_2 Q (l/min)"=0.0, "Trace Gas Concentration (%)"=0.0, "Specific Arguments"="Z= ;12.8;19.2;25.5\r", "Comments"="Anemo1", "Row No"=0, "Row Type Selector"=enum."Vertical Profile", "Completion time"="", "Row Duration (mins)"=0.0, "No. of Valid pts."=0, "Meas Setup File"="Current_Setup.xls"}, {"Start X"=0.0, "Start Y"=0.0, "Start Z"=0.0, "End X"=0.0, "End Y"=0.0, "End Z"=0.0, "No. of pts."=0, "Spacing"=enum."Linear", "Filename"=path "M:/\\Projects\\8773\\Results\\Tunnel1\\AnemometerSurvey.xls", "Tunnel Speed"=0.0, "Averaging time (min)"=0.0, "Extra Commands"="-4.700", "Carrier_1 Q (l/min)"=0.0, "Carrier_2 Q (l/min)"=0.0, "Trace Gas Concentration (%)"=0.0, "Specific Arguments"="T1:Z:Corrections", "Comments"="", "Row No"=0, "Row Type Selector"=enum."Set ADAM Ch", "Completion time"="", "Row Duration (mins)"=0.0, "No. of Valid pts."=0, "Meas Setup File"="Current_Setup.xls"}, {"Start X"=-458.4, "Start Y"=87.9, "Start Z"=20.9, "End X"=-458.4, "End Y"=87.9, "End Z"=33.6, "No. of pts."=3, "Spacing"=enum."Specified", "Filename"=path "M:/\\Projects\\8773\\Results\\Tunnel1\\AnemometerSurvey.xls", "Tunnel Speed"=7.64, "Averaging time (min)"=1.0, "Extra Commands"="", "Carrier_1 Q (l/min)"=0.0, "Carrier_2 Q (l/min)"=0.0, "Trace Gas Concentration (%)"=0.0, "Specific Arguments"="Z= ;20.9;27.2;33.6\r", "Comments"="Anemo2", "Row No"=0, "Row Type Selector"=enum."Vertical Profile", "Completion time"="", "Row Duration (mins)"=0.0, "No. of Valid pts."=0, "Meas Setup File"="Current_Setup.xls"}, {"Start X"=0.0, "Start Y"=0.0, "Start Z"=150.0, "End X"=0.0, "End Y"=0.0, "End Z"=150.0, "No. of pts."=0, "Spacing"=enum."Linear", "Filename"=path "M:/\\Projects\\8773\\Results\\Tunnel1\\AnemometerSurvey.xls", "Tunnel Speed"=0.0, "Averaging time (min)"=0.0, "Extra Commands"="!Work in Tunnel Coordinates", "Carrier_1 Q (l/min)"=0.0, "Carrier_2 Q (l/min)"=0.0, "Trace Gas Concentration (%)"=0.0, "Specific Arguments"="", "Comments"="", "Row No"=0, "Row Type Selector"=enum."Move Traverse Only", "Completion time"="", "Row Duration (mins)"=0.0, "No. of Valid pts."=0, "Meas Setup File"="Current_Setup.xls"}, {"Start X"=0.0, "Start Y"=0.0, "Start Z"=0.0, "End X"=0.0, "End Y"=0.0, "End Z"=0.0, "No. of pts."=0, "Spacing"=enum."Linear", "Filename"=path "M:/\\Projects\\8773\\Results\\Tunnel1\\AnemometerSurvey.xls", "Tunnel Speed"=0.0, "Averaging time (min)"=0.0, "Extra Commands"="", "Carrier_1 Q (l/min)"=0.0, "Carrier_2 Q (l/min)"=0.0, "Trace Gas Concentration (%)"=0.0, "Specific Arguments"="", "Comments"="Time to set ramps...", "Row No"=0, "Row Type Selector"=enum."Send Message", "Completion time"="", "Row Duration (mins)"=0.0, "No. of Valid pts."=0, "Meas Setup File"="Current_Setup.xls"}, {"Start X"=0.0, "Start Y"=0.0, "Start Z"=0.0, "End X"=0.0, "End Y"=0.0, "End Z"=0.0, "No. of pts."=0, "Spacing"=enum."Linear", "Filename"=path "", "Tunnel Speed"=0.0, "Averaging time (min)"=0.0, "Extra Commands"="", "Carrier_1 Q (l/min)"=0.0, "Carrier_2 Q (l/min)"=0.0, "Trace Gas Concentration (%)"=0.0, "Specific Arguments"="", "Comments"="", "Row No"=0, "Row Type Selector"=enum."Blank Row", "Completion time"="", "Row Duration (mins)"=0.0, "No. of Valid pts."=0, "Meas Setup File"=""}, {"Start X"=0.0, "Start Y"=0.0, "Start Z"=780.0, "End X"=0.0, "End Y"=0.0, "End Z"=780.0, "No. of pts."=0, "Spacing"=enum."Linear", "Filename"=path "M:/\\Projects\\8773\\Results\\Tunnel1\\AnemometerSurvey.xls", "Tunnel Speed"=7.64, "Averaging time (min)"=1.0, "Extra Commands"="!Work in Tunnel Coordinates", "Carrier_1 Q (l/min)"=0.0, "Carrier_2 Q (l/min)"=0.0, "Trace Gas Concentration (%)"=0.0, "Specific Arguments"="", "Comments"="LocalCalCheck", "Row No"=0, "Row Type Selector"=enum."Single Measurement", "Completion time"="", "Row Duration (mins)"=0.0, "No. of Valid pts."=0, "Meas Setup File"="Current_Setup.xls"}, {"Start X"=0.0, "Start Y"=0.0, "Start Z"=0.0, "End X"=0.0, "End Y"=0.0, "End Z"=0.0, "No. of pts."=0, "Spacing"=enum."N/A", "Filename"=path "M:/\\Projects\\8773\\Results\\Tunnel1\\AnemometerSurvey.xls", "Tunnel Speed"=0.0, "Averaging time (min)"=0.0, "Extra Commands"="", "Carrier_1 Q (l/min)"=0.0, "Carrier_2 Q (l/min)"=0.0, "Trace Gas Concentration (%)"=0.0, "Specific Arguments"="MoveTT.vi;180", "Comments"="", "Row No"=0, "Row Type Selector"=enum."Run VI Named:", "Completion time"="", "Row Duration (mins)"=0.0, "No. of Valid pts."=0, "Meas Setup File"="Current_Setup.xls"}, {"Start X"=0.0, "Start Y"=0.0, "Start Z"=0.0, "End X"=0.0, "End Y"=0.0, "End Z"=0.0, "No. of pts."=0, "Spacing"=enum."Linear", "Filename"=path "M:/\\Projects\\8773\\Results\\Tunnel1\\AnemometerSurvey.xls", "Tunnel Speed"=0.0, "Averaging time (min)"=0.0, "Extra Commands"="", "Carrier_1 Q (l/min)"=0.0, "Carrier_2 Q (l/min)"=0.0, "Trace Gas Concentration (%)"=0.0, "Specific Arguments"="1440.00", "Comments"="", "Row No"=0, "Row Type Selector"=enum."Wait (minutes)", "Completion time"="", "Row Duration (mins)"=0.0, "No. of Valid pts."=0, "Meas Setup File"="Current_Setup.xls"}, {"Start X"=0.0, "Start Y"=0.0, "Start Z"=0.0, "End X"=0.0, "End Y"=0.0, "End Z"=0.0, "No. of pts."=0, "Spacing"=enum."Linear", "Filename"=path "M:/\\Projects\\8773\\Results\\Tunnel1\\AnemometerSurvey.xls", "Tunnel Speed"=0.0, "Averaging time (min)"=0.0, "Extra Commands"="0.500", "Carrier_1 Q (l/min)"=0.0, "Carrier_2 Q (l/min)"=0.0, "Trace Gas Concentration (%)"=0.0, "Specific Arguments"="T1:Z:Corrections", "Comments"="", "Row No"=0, "Row Type Selector"=enum."Set ADAM Ch", "Completion time"="", "Row Duration (mins)"=0.0, "No. of Valid pts."=0, "Meas Setup File"="Current_Setup.xls"}, {"Start X"=-72.9, "Start Y"=-56.5, "Start Z"=13.2, "End X"=-72.9, "End Y"=-56.5, "End Z"=25.9, "No. of pts."=3, "Spacing"=enum."Specified", "Filename"=path "M:/\\Projects\\8773\\Results\\Tunnel1\\AnemometerSurvey.xls", "Tunnel Speed"=7.64, "Averaging time (min)"=1.0, "Extra Commands"="", "Carrier_1 Q (l/min)"=0.0, "Carrier_2 Q (l/min)"=0.0, "Trace Gas Concentration (%)"=0.0, "Specific Arguments"="Z= ;13.2;19.6;25.9\r", "Comments"="Anemo1", "Row No"=0, "Row Type Selector"=enum."Vertical Profile", "Completion time"="", "Row Duration (mins)"=0.0, "No. of Valid pts."=0, "Meas Setup File"="Current_Setup.xls"}, {"Start X"=0.0, "Start Y"=0.0, "Start Z"=0.0, "End X"=0.0, "End Y"=0.0, "End Z"=0.0, "No. of pts."=0, "Spacing"=enum."Linear", "Filename"=path "M:/\\Projects\\8773\\Results\\Tunnel1\\AnemometerSurvey.xls", "Tunnel Speed"=0.0, "Averaging time (min)"=0.0, "Extra Commands"="-3.900", "Carrier_1 Q (l/min)"=0.0, "Carrier_2 Q (l/min)"=0.0, "Trace Gas Concentration (%)"=0.0, "Specific Arguments"="T1:Z:Corrections", "Comments"="", "Row No"=0, "Row Type Selector"=enum."Set ADAM Ch", "Completion time"="", "Row Duration (mins)"=0.0, "No. of Valid pts."=0, "Meas Setup File"="Current_Setup.xls"}, {"Start X"=-458.4, "Start Y"=87.9, "Start Z"=21.7, "End X"=-458.4, "End Y"=87.9, "End Z"=34.4, "No. of pts."=3, "Spacing"=enum."Specified", "Filename"=path "M:/\\Projects\\8773\\Results\\Tunnel1\\AnemometerSurvey.xls", "Tunnel Speed"=7.64, "Averaging time (min)"=1.0, "Extra Commands"="", "Carrier_1 Q (l/min)"=0.0, "Carrier_2 Q (l/min)"=0.0, "Trace Gas Concentration (%)"=0.0, "Specific Arguments"="Z= ;21.7;28.0;34.4\r", "Comments"="Anemo2", "Row No"=0, "Row Type Selector"=enum."Vertical Profile", "Completion time"="", "Row Duration (mins)"=0.0, "No. of Valid pts."=0, "Meas Setup File"="Current_Setup.xls"}, {"Start X"=0.0, "Start Y"=0.0, "Start Z"=150.0, "End X"=0.0, "End Y"=0.0, "End Z"=150.0, "No. of pts."=0, "Spacing"=enum."Linear", "Filename"=path "M:/\\Projects\\8773\\Results\\Tunnel1\\AnemometerSurvey.xls", "Tunnel Speed"=0.0, "Averaging time (min)"=0.0, "Extra Commands"="!Work in Tunnel Coordinates", "Carrier_1 Q (l/min)"=0.0, "Carrier_2 Q (l/min)"=0.0, "Trace Gas Concentration (%)"=0.0, "Specific Arguments"="", "Comments"="", "Row No"=0, "Row Type Selector"=enum."Move Traverse Only", "Completion time"="", "Row Duration (mins)"=0.0, "No. of Valid pts."=0, "Meas Setup File"="Current_Setup.xls"}, {"Start X"=0.0, "Start Y"=0.0, "Start Z"=0.0, "End X"=0.0, "End Y"=0.0, "End Z"=0.0, "No. of pts."=0, "Spacing"=enum."Linear", "Filename"=path "M:/\\Projects\\8773\\Results\\Tunnel1\\AnemometerSurvey.xls", "Tunnel Speed"=0.0, "Averaging time (min)"=0.0, "Extra Commands"="", "Carrier_1 Q (l/min)"=0.0, "Carrier_2 Q (l/min)"=0.0, "Trace Gas Concentration (%)"=0.0, "Specific Arguments"="", "Comments"="Time to set ramps...", "Row No"=0, "Row Type Selector"=enum."Send Message", "Completion time"="", "Row Duration (mins)"=0.0, "No. of Valid pts."=0, "Meas Setup File"="Current_Setup.xls"}, {"Start X"=0.0, "Start Y"=0.0, "Start Z"=0.0, "End X"=0.0, "End Y"=0.0, "End Z"=0.0, "No. of pts."=0, "Spacing"=enum."Linear", "Filename"=path "", "Tunnel Speed"=0.0, "Averaging time (min)"=0.0, "Extra Commands"="", "Carrier_1 Q (l/min)"=0.0, "Carrier_2 Q (l/min)"=0.0, "Trace Gas Concentration (%)"=0.0, "Specific Arguments"="", "Comments"="", "Row No"=0, "Row Type Selector"=enum."Blank Row", "Completion time"="", "Row Duration (mins)"=0.0, "No. of Valid pts."=0, "Meas Setup File"=""}, {"Start X"=0.0, "Start Y"=0.0, "Start Z"=0.0, "End X"=0.0, "End Y"=0.0, "End Z"=0.0, "No. of pts."=0, "Spacing"=enum."N/A", "Filename"=path "M:/\\Projects\\8773\\Results\\Tunnel1\\AnemometerSurvey.xls", "Tunnel Speed"=0.0, "Averaging time (min)"=0.0, "Extra Commands"="", "Carrier_1 Q (l/min)"=0.0, "Carrier_2 Q (l/min)"=0.0, "Trace Gas Concentration (%)"=0.0, "Specific Arguments"="MoveTT.vi;200", "Comments"="", "Row No"=0, "Row Type Selector"=enum."Run VI Named:", "Completion time"="", "Row Duration (mins)"=0.0, "No. of Valid pts."=0, "Meas Setup File"="Current_Setup.xls"}, {"Start X"=0.0, "Start Y"=0.0, "Start Z"=0.0, "End X"=0.0, "End Y"=0.0, "End Z"=0.0, "No. of pts."=0, "Spacing"=enum."Linear", "Filename"=path "M:/\\Projects\\8773\\Results\\Tunnel1\\AnemometerSurvey.xls", "Tunnel Speed"=0.0, "Averaging time (min)"=0.0, "Extra Commands"="", "Carrier_1 Q (l/min)"=0.0, "Carrier_2 Q (l/min)"=0.0, "Trace Gas Concentration (%)"=0.0, "Specific Arguments"="1440.00", "Comments"="", "Row No"=0, "Row Type Selector"=enum."Wait (minutes)", "Completion time"="", "Row Duration (mins)"=0.0, "No. of Valid pts."=0, "Meas Setup File"="Current_Setup.xls"}, {"Start X"=0.0, "Start Y"=0.0, "Start Z"=0.0, "End X"=0.0, "End Y"=0.0, "End Z"=0.0, "No. of pts."=0, "Spacing"=enum."Linear", "Filename"=path "M:/\\Projects\\8773\\Results\\Tunnel1\\AnemometerSurvey.xls", "Tunnel Speed"=0.0, "Averaging time (min)"=0.0, "Extra Commands"="0.600", "Carrier_1 Q (l/min)"=0.0, "Carrier_2 Q (l/min)"=0.0, "Trace Gas Concentration (%)"=0.0, "Specific Arguments"="T1:Z:Corrections", "Comments"="", "Row No"=0, "Row Type Selector"=enum."Set ADAM Ch", "Completion time"="", "Row Duration (mins)"=0.0, "No. of Valid pts."=0, "Meas Setup File"="Current_Setup.xls"}, {"Start X"=-72.9, "Start Y"=-56.5, "Start Z"=13.3, "End X"=-72.9, "End Y"=-56.5, "End Z"=26.0, "No. of pts."=3, "Spacing"=enum."Specified", "Filename"=path "M:/\\Projects\\8773\\Results\\Tunnel1\\AnemometerSurvey.xls", "Tunnel Speed"=7.64, "Averaging time (min)"=1.0, "Extra Commands"="", "Carrier_1 Q (l/min)"=0.0, "Carrier_2 Q (l/min)"=0.0, "Trace Gas Concentration (%)"=0.0, "Specific Arguments"="Z= ;13.3;19.7;26.0\r", "Comments"="Anemo1", "Row No"=0, "Row Type Selector"=enum."Vertical Profile", "Completion time"="", "Row Duration (mins)"=0.0, "No. of Valid pts."=0, "Meas Setup File"="Current_Setup.xls"}, {"Start X"=0.0, "Start Y"=0.0, "Start Z"=0.0, "End X"=0.0, "End Y"=0.0, "End Z"=0.0, "No. of pts."=0, "Spacing"=enum."Linear", "Filename"=path "M:/\\Projects\\8773\\Results\\Tunnel1\\AnemometerSurvey.xls", "Tunnel Speed"=0.0, "Averaging time (min)"=0.0, "Extra Commands"="-2.700", "Carrier_1 Q (l/min)"=0.0, "Carrier_2 Q (l/min)"=0.0, "Trace Gas Concentration (%)"=0.0, "Specific Arguments"="T1:Z:Corrections", "Comments"="", "Row No"=0, "Row Type Selector"=enum."Set ADAM Ch", "Completion time"="", "Row Duration (mins)"=0.0, "No. of Valid pts."=0, "Meas Setup File"="Current_Setup.xls"}, {"Start X"=-458.4, "Start Y"=87.9, "Start Z"=22.9, "End X"=-458.4, "End Y"=87.9, "End Z"=35.6, "No. of pts."=3, "Spacing"=enum."Specified", "Filename"=path "M:/\\Projects\\8773\\Results\\Tunnel1\\AnemometerSurvey.xls", "Tunnel Speed"=7.64, "Averaging time (min)"=1.0, "Extra Commands"="", "Carrier_1 Q (l/min)"=0.0, "Carrier_2 Q (l/min)"=0.0, "Trace Gas Concentration (%)"=0.0, "Specific Arguments"="Z= ;22.9;29.2;35.6\r", "Comments"="Anemo2", "Row No"=0, "Row Type Selector"=enum."Vertical Profile", "Completion time"="", "Row Duration (mins)"=0.0, "No. of Valid pts."=0, "Meas Setup File"="Current_Setup.xls"}, {"Start X"=0.0, "Start Y"=0.0, "Start Z"=150.0, "End X"=0.0, "End Y"=0.0, "End Z"=150.0, "No. of pts."=0, "Spacing"=enum."Linear", "Filename"=path "M:/\\Projects\\8773\\Results\\Tunnel1\\AnemometerSurvey.xls", "Tunnel Speed"=0.0, "Averaging time (min)"=0.0, "Extra Commands"="!Work in Tunnel Coordinates", "Carrier_1 Q (l/min)"=0.0, "Carrier_2 Q (l/min)"=0.0, "Trace Gas Concentration (%)"=0.0, "Specific Arguments"="", "Comments"="", "Row No"=0, "Row Type Selector"=enum."Move Traverse Only", "Completion time"="", "Row Duration (mins)"=0.0, "No. of Valid pts."=0, "Meas Setup File"="Current_Setup.xls"}, {"Start X"=0.0, "Start Y"=0.0, "Start Z"=0.0, "End X"=0.0, "End Y"=0.0, "End Z"=0.0, "No. of pts."=0, "Spacing"=enum."Linear", "Filename"=path "M:/\\Projects\\8773\\Results\\Tunnel1\\AnemometerSurvey.xls", "Tunnel Speed"=0.0, "Averaging time (min)"=0.0, "Extra Commands"="", "Carrier_1 Q (l/min)"=0.0, "Carrier_2 Q (l/min)"=0.0, "Trace Gas Concentration (%)"=0.0, "Specific Arguments"="", "Comments"="Time to set ramps...", "Row No"=0, "Row Type Selector"=enum."Send Message", "Completion time"="", "Row Duration (mins)"=0.0, "No. of Valid pts."=0, "Meas Setup File"="Current_Setup.xls"}, {"Start X"=0.0, "Start Y"=0.0, "Start Z"=0.0, "End X"=0.0, "End Y"=0.0, "End Z"=0.0, "No. of pts."=0, "Spacing"=enum."Linear", "Filename"=path "", "Tunnel Speed"=0.0, "Averaging time (min)"=0.0, "Extra Commands"="", "Carrier_1 Q (l/min)"=0.0, "Carrier_2 Q (l/min)"=0.0, "Trace Gas Concentration (%)"=0.0, "Specific Arguments"="", "Comments"="", "Row No"=0, "Row Type Selector"=enum."Blank Row", "Completion time"="", "Row Duration (mins)"=0.0, "No. of Valid pts."=0, "Meas Setup File"=""}, {"Start X"=0.0, "Start Y"=0.0, "Start Z"=0.0, "End X"=0.0, "End Y"=0.0, "End Z"=0.0, "No. of pts."=0, "Spacing"=enum."N/A", "Filename"=path "M:/\\Projects\\8773\\Results\\Tunnel1\\AnemometerSurvey.xls", "Tunnel Speed"=0.0, "Averaging time (min)"=0.0, "Extra Commands"="", "Carrier_1 Q (l/min)"=0.0, "Carrier_2 Q (l/min)"=0.0, "Trace Gas Concentration (%)"=0.0, "Specific Arguments"="MoveTT.vi;220", "Comments"="", "Row No"=0, "Row Type Selector"=enum."Run VI Named:", "Completion time"="", "Row Duration (mins)"=0.0, "No. of Valid pts."=0, "Meas Setup File"="Current_Setup.xls"}, {"Start X"=0.0, "Start Y"=0.0, "Start Z"=0.0, "End X"=0.0, "End Y"=0.0, "End Z"=0.0, "No. of pts."=0, "Spacing"=enum."Linear", "Filename"=path "M:/\\Projects\\8773\\Results\\Tunnel1\\AnemometerSurvey.xls", "Tunnel Speed"=0.0, "Averaging time (min)"=0.0, "Extra Commands"="", "Carrier_1 Q (l/min)"=0.0, "Carrier_2 Q (l/min)"=0.0, "Trace Gas Concentration (%)"=0.0, "Specific Arguments"="1440.00", "Comments"="", "Row No"=0, "Row Type Selector"=enum."Wait (minutes)", "Completion time"="", "Row Duration (mins)"=0.0, "No. of Valid pts."=0, "Meas Setup File"="Current_Setup.xls"}, {"Start X"=0.0, "Start Y"=0.0, "Start Z"=0.0, "End X"=0.0, "End Y"=0.0, "End Z"=0.0, "No. of pts."=0, "Spacing"=enum."Linear", "Filename"=path "M:/\\Projects\\8773\\Results\\Tunnel1\\AnemometerSurvey.xls", "Tunnel Speed"=0.0, "Averaging time (min)"=0.0, "Extra Commands"="0.100", "Carrier_1 Q (l/min)"=0.0, "Carrier_2 Q (l/min)"=0.0, "Trace Gas Concentration (%)"=0.0, "Specific Arguments"="T1:Z:Corrections", "Comments"="", "Row No"=0, "Row Type Selector"=enum."Set ADAM Ch", "Completion time"="", "Row Duration (mins)"=0.0, "No. of Valid pts."=0, "Meas Setup File"="Current_Setup.xls"}, {"Start X"=-72.9, "Start Y"=-56.5, "Start Z"=12.8, "End X"=-72.9, "End Y"=-56.5, "End Z"=25.5, "No. of pts."=3, "Spacing"=enum."Specified", "Filename"=path "M:/\\Projects\\8773\\Results\\Tunnel1\\AnemometerSurvey.xls", "Tunnel Speed"=7.64, "Averaging time (min)"=1.0, "Extra Commands"="", "Carrier_1 Q (l/min)"=0.0, "Carrier_2 Q (l/min)"=0.0, "Trace Gas Concentration (%)"=0.0, "Specific Arguments"="Z= ;12.8;19.2;25.5\r", "Comments"="Anemo1", "Row No"=0, "Row Type Selector"=enum."Vertical Profile", "Completion time"="", "Row Duration (mins)"=0.0, "No. of Valid pts."=0, "Meas Setup File"="Current_Setup.xls"}, {"Start X"=0.0, "Start Y"=0.0, "Start Z"=0.0, "End X"=0.0, "End Y"=0.0, "End Z"=0.0, "No. of pts."=0, "Spacing"=enum."Linear", "Filename"=path "M:/\\Projects\\8773\\Results\\Tunnel1\\AnemometerSurvey.xls", "Tunnel Speed"=0.0, "Averaging time (min)"=0.0, "Extra Commands"="-2.100", "Carrier_1 Q (l/min)"=0.0, "Carrier_2 Q (l/min)"=0.0, "Trace Gas Concentration (%)"=0.0, "Specific Arguments"="T1:Z:Corrections", "Comments"="", "Row No"=0, "Row Type Selector"=enum."Set ADAM Ch", "Completion time"="", "Row Duration (mins)"=0.0, "No. of Valid pts."=0, "Meas Setup File"="Current_Setup.xls"}, {"Start X"=-458.4, "Start Y"=87.9, "Start Z"=23.5, "End X"=-458.4, "End Y"=87.9, "End Z"=36.2, "No. of pts."=3, "Spacing"=enum."Specified", "Filename"=path "M:/\\Projects\\8773\\Results\\Tunnel1\\AnemometerSurvey.xls", "Tunnel Speed"=7.64, "Averaging time (min)"=1.0, "Extra Commands"="", "Carrier_1 Q (l/min)"=0.0, "Carrier_2 Q (l/min)"=0.0, "Trace Gas Concentration (%)"=0.0, "Specific Arguments"="Z= ;23.5;29.8;36.2\r", "Comments"="Anemo2", "Row No"=0, "Row Type Selector"=enum."Vertical Profile", "Completion time"="", "Row Duration (mins)"=0.0, "No. of Valid pts."=0, "Meas Setup File"="Current_Setup.xls"}, {"Start X"=0.0, "Start Y"=0.0, "Start Z"=150.0, "End X"=0.0, "End Y"=0.0, "End Z"=150.0, "No. of pts."=0, "Spacing"=enum."Linear", "Filename"=path "M:/\\Projects\\8773\\Results\\Tunnel1\\AnemometerSurvey.xls", "Tunnel Speed"=0.0, "Averaging time (min)"=0.0, "Extra Commands"="!Work in Tunnel Coordinates", "Carrier_1 Q (l/min)"=0.0, "Carrier_2 Q (l/min)"=0.0, "Trace Gas Concentration (%)"=0.0, "Specific Arguments"="", "Comments"="", "Row No"=0, "Row Type Selector"=enum."Move Traverse Only", "Completion time"="", "Row Duration (mins)"=0.0, "No. of Valid pts."=0, "Meas Setup File"="Current_Setup.xls"}, {"Start X"=0.0, "Start Y"=0.0, "Start Z"=0.0, "End X"=0.0, "End Y"=0.0, "End Z"=0.0, "No. of pts."=0, "Spacing"=enum."Linear", "Filename"=path "M:/\\Projects\\8773\\Results\\Tunnel1\\AnemometerSurvey.xls", "Tunnel Speed"=0.0, "Averaging time (min)"=0.0, "Extra Commands"="", "Carrier_1 Q (l/min)"=0.0, "Carrier_2 Q (l/min)"=0.0, "Trace Gas Concentration (%)"=0.0, "Specific Arguments"="", "Comments"="Time to set ramps...", "Row No"=0, "Row Type Selector"=enum."Send Message", "Completion time"="", "Row Duration (mins)"=0.0, "No. of Valid pts."=0, "Meas Setup File"="Current_Setup.xls"}, {"Start X"=0.0, "Start Y"=0.0, "Start Z"=0.0, "End X"=0.0, "End Y"=0.0, "End Z"=0.0, "No. of pts."=0, "Spacing"=enum."Linear", "Filename"=path "", "Tunnel Speed"=0.0, "Averaging time (min)"=0.0, "Extra Commands"="", "Carrier_1 Q (l/min)"=0.0, "Carrier_2 Q (l/min)"=0.0, "Trace Gas Concentration (%)"=0.0, "Specific Arguments"="", "Comments"="", "Row No"=0, "Row Type Selector"=enum."Blank Row", "Completion time"="", "Row Duration (mins)"=0.0, "No. of Valid pts."=0, "Meas Setup File"=""}, {"Start X"=-3390.0, "Start Y"=-113.0, "Start Z"=780.0, "End X"=-3390.0, "End Y"=-113.0, "End Z"=780.0, "No. of pts."=0, "Spacing"=enum."Linear", "Filename"=path "M:/\\Projects\\8773\\Results\\Tunnel1\\AnemometerSurvey.xls", "Tunnel Speed"=0.0, "Averaging time (min)"=1.0, "Extra Commands"="!Work in Tunnel Coordinates", "Carrier_1 Q (l/min)"=0.0, "Carrier_2 Q (l/min)"=0.0, "Trace Gas Concentration (%)"=0.0, "Specific Arguments"="", "Comments"="Zeroes", "Row No"=0, "Row Type Selector"=enum."Single Measurement", "Completion time"="", "Row Duration (mins)"=0.0, "No. of Valid pts."=0, "Meas Setup File"="Current_Setup.xls"}, {"Start X"=-3390.0, "Start Y"=-113.0, "Start Z"=780.0, "End X"=-3390.0, "End Y"=-113.0, "End Z"=780.0, "No. of pts."=0, "Spacing"=enum."Linear", "Filename"=path "M:/\\Projects\\8773\\Results\\Tunnel1\\AnemometerSurvey.xls", "Tunnel Speed"=7.64, "Averaging time (min)"=1.0, "Extra Commands"="!Work in Tunnel Coordinates", "Carrier_1 Q (l/min)"=0.0, "Carrier_2 Q (l/min)"=0.0, "Trace Gas Concentration (%)"=0.0, "Specific Arguments"="", "Comments"="CalCheck", "Row No"=0, "Row Type Selector"=enum."Single Measurement", "Completion time"="", "Row Duration (mins)"=0.0, "No. of Valid pts."=0, "Meas Setup File"="Current_Setup.xls"}, {"Start X"=0.0, "Start Y"=0.0, "Start Z"=780.0, "End X"=0.0, "End Y"=0.0, "End Z"=780.0, "No. of pts."=0, "Spacing"=enum."Linear", "Filename"=path "M:/\\Projects\\8773\\Results\\Tunnel1\\AnemometerSurvey.xls", "Tunnel Speed"=7.64, "Averaging time (min)"=1.0, "Extra Commands"="!Work in Tunnel Coordinates", "Carrier_1 Q (l/min)"=0.0, "Carrier_2 Q (l/min)"=0.0, "Trace Gas Concentration (%)"=0.0, "Specific Arguments"="", "Comments"="LocalCalCheck", "Row No"=0, "Row Type Selector"=enum."Single Measurement", "Completion time"="", "Row Duration (mins)"=0.0, "No. of Valid pts."=0, "Meas Setup File"="Current_Setup.xls"}, {"Start X"=0.0, "Start Y"=0.0, "Start Z"=0.0, "End X"=0.0, "End Y"=0.0, "End Z"=0.0, "No. of pts."=0, "Spacing"=enum."N/A", "Filename"=path "M:/\\Projects\\8773\\Results\\Tunnel1\\AnemometerSurvey.xls", "Tunnel Speed"=0.0, "Averaging time (min)"=0.0, "Extra Commands"="", "Carrier_1 Q (l/min)"=0.0, "Carrier_2 Q (l/min)"=0.0, "Trace Gas Concentration (%)"=0.0, "Specific Arguments"="MoveTT.vi;240", "Comments"="", "Row No"=0, "Row Type Selector"=enum."Run VI Named:", "Completion time"="", "Row Duration (mins)"=0.0, "No. of Valid pts."=0, "Meas Setup File"="Current_Setup.xls"}, {"Start X"=0.0, "Start Y"=0.0, "Start Z"=0.0, "End X"=0.0, "End Y"=0.0, "End Z"=0.0, "No. of pts."=0, "Spacing"=enum."Linear", "Filename"=path "M:/\\Projects\\8773\\Results\\Tunnel1\\AnemometerSurvey.xls", "Tunnel Speed"=0.0, "Averaging time (min)"=0.0, "Extra Commands"="", "Carrier_1 Q (l/min)"=0.0, "Carrier_2 Q (l/min)"=0.0, "Trace Gas Concentration (%)"=0.0, "Specific Arguments"="1440.00", "Comments"="", "Row No"=0, "Row Type Selector"=enum."Wait (minutes)", "Completion time"="", "Row Duration (mins)"=0.0, "No. of Valid pts."=0, "Meas Setup File"="Current_Setup.xls"}, {"Start X"=0.0, "Start Y"=0.0, "Start Z"=0.0, "End X"=0.0, "End Y"=0.0, "End Z"=0.0, "No. of pts."=0, "Spacing"=enum."Linear", "Filename"=path "M:/\\Projects\\8773\\Results\\Tunnel1\\AnemometerSurvey.xls", "Tunnel Speed"=0.0, "Averaging time (min)"=0.0, "Extra Commands"="0.600", "Carrier_1 Q (l/min)"=0.0, "Carrier_2 Q (l/min)"=0.0, "Trace Gas Concentration (%)"=0.0, "Specific Arguments"="T1:Z:Corrections", "Comments"="", "Row No"=0, "Row Type Selector"=enum."Set ADAM Ch", "Completion time"="", "Row Duration (mins)"=0.0, "No. of Valid pts."=0, "Meas Setup File"="Current_Setup.xls"}, {"Start X"=-72.9, "Start Y"=-56.5, "Start Z"=13.3, "End X"=-72.9, "End Y"=-56.5, "End Z"=26.0, "No. of pts."=3, "Spacing"=enum."Specified", "Filename"=path "M:/\\Projects\\8773\\Results\\Tunnel1\\AnemometerSurvey.xls", "Tunnel Speed"=7.64, "Averaging time (min)"=1.0, "Extra Commands"="", "Carrier_1 Q (l/min)"=0.0, "Carrier_2 Q (l/min)"=0.0, "Trace Gas Concentration (%)"=0.0, "Specific Arguments"="Z= ;13.3;19.7;26.0\r", "Comments"="Anemo1", "Row No"=0, "Row Type Selector"=enum."Vertical Profile", "Completion time"="", "Row Duration (mins)"=0.0, "No. of Valid pts."=0, "Meas Setup File"="Current_Setup.xls"}, {"Start X"=0.0, "Start Y"=0.0, "Start Z"=0.0, "End X"=0.0, "End Y"=0.0, "End Z"=0.0, "No. of pts."=0, "Spacing"=enum."Linear", "Filename"=path "M:/\\Projects\\8773\\Results\\Tunnel1\\AnemometerSurvey.xls", "Tunnel Speed"=0.0, "Averaging time (min)"=0.0, "Extra Commands"="-0.900", "Carrier_1 Q (l/min)"=0.0, "Carrier_2 Q (l/min)"=0.0, "Trace Gas Concentration (%)"=0.0, "Specific Arguments"="T1:Z:Corrections", "Comments"="", "Row No"=0, "Row Type Selector"=enum."Set ADAM Ch", "Completion time"="", "Row Duration (mins)"=0.0, "No. of Valid pts."=0, "Meas Setup File"="Current_Setup.xls"}, {"Start X"=-458.4, "Start Y"=87.9, "Start Z"=24.7, "End X"=-458.4, "End Y"=87.9, "End Z"=37.4, "No. of pts."=3, "Spacing"=enum."Specified", "Filename"=path "M:/\\Projects\\8773\\Results\\Tunnel1\\AnemometerSurvey.xls", "Tunnel Speed"=7.64, "Averaging time (min)"=1.0, "Extra Commands"="", "Carrier_1 Q (l/min)"=0.0, "Carrier_2 Q (l/min)"=0.0, "Trace Gas Concentration (%)"=0.0, "Specific Arguments"="Z= ;24.7;31.0;37.4\r", "Comments"="Anemo2", "Row No"=0, "Row Type Selector"=enum."Vertical Profile", "Completion time"="", "Row Duration (mins)"=0.0, "No. of Valid pts."=0, "Meas Setup File"="Current_Setup.xls"}, {"Start X"=0.0, "Start Y"=0.0, "Start Z"=150.0, "End X"=0.0, "End Y"=0.0, "End Z"=150.0, "No. of pts."=0, "Spacing"=enum."Linear", "Filename"=path "M:/\\Projects\\8773\\Results\\Tunnel1\\AnemometerSurvey.xls", "Tunnel Speed"=0.0, "Averaging time (min)"=0.0, "Extra Commands"="!Work in Tunnel Coordinates", "Carrier_1 Q (l/min)"=0.0, "Carrier_2 Q (l/min)"=0.0, "Trace Gas Concentration (%)"=0.0, "Specific Arguments"="", "Comments"="", "Row No"=0, "Row Type Selector"=enum."Move Traverse Only", "Completion time"="", "Row Duration (mins)"=0.0, "No. of Valid pts."=0, "Meas Setup File"="Current_Setup.xls"}, {"Start X"=0.0, "Start Y"=0.0, "Start Z"=0.0, "End X"=0.0, "End Y"=0.0, "End Z"=0.0, "No. of pts."=0, "Spacing"=enum."Linear", "Filename"=path "M:/\\Projects\\8773\\Results\\Tunnel1\\AnemometerSurvey.xls", "Tunnel Speed"=0.0, "Averaging time (min)"=0.0, "Extra Commands"="", "Carrier_1 Q (l/min)"=0.0, "Carrier_2 Q (l/min)"=0.0, "Trace Gas Concentration (%)"=0.0, "Specific Arguments"="", "Comments"="Time to set ramps...", "Row No"=0, "Row Type Selector"=enum."Send Message", "Completion time"="", "Row Duration (mins)"=0.0, "No. of Valid pts."=0, "Meas Setup File"="Current_Setup.xls"}, {"Start X"=0.0, "Start Y"=0.0, "Start Z"=0.0, "End X"=0.0, "End Y"=0.0, "End Z"=0.0, "No. of pts."=0, "Spacing"=enum."Linear", "Filename"=path "", "Tunnel Speed"=0.0, "Averaging time (min)"=0.0, "Extra Commands"="", "Carrier_1 Q (l/min)"=0.0, "Carrier_2 Q (l/min)"=0.0, "Trace Gas Concentration (%)"=0.0, "Specific Arguments"="", "Comments"="", "Row No"=0, "Row Type Selector"=enum."Blank Row", "Completion time"="", "Row Duration (mins)"=0.0, "No. of Valid pts."=0, "Meas Setup File"=""}, {"Start X"=0.0, "Start Y"=0.0, "Start Z"=0.0, "End X"=0.0, "End Y"=0.0, "End Z"=0.0, "No. of pts."=0, "Spacing"=enum."N/A", "Filename"=path "M:/\\Projects\\8773\\Results\\Tunnel1\\AnemometerSurvey.xls", "Tunnel Speed"=0.0, "Averaging time (min)"=0.0, "Extra Commands"="", "Carrier_1 Q (l/min)"=0.0, "Carrier_2 Q (l/min)"=0.0, "Trace Gas Concentration (%)"=0.0, "Specific Arguments"="MoveTT.vi;260", "Comments"="", "Row No"=0, "Row Type Selector"=enum."Run VI Named:", "Completion time"="", "Row Duration (mins)"=0.0, "No. of Valid pts."=0, "Meas Setup File"="Current_Setup.xls"}, {"Start X"=0.0, "Start Y"=0.0, "Start Z"=0.0, "End X"=0.0, "End Y"=0.0, "End Z"=0.0, "No. of pts."=0, "Spacing"=enum."Linear", "Filename"=path "M:/\\Projects\\8773\\Results\\Tunnel1\\AnemometerSurvey.xls", "Tunnel Speed"=0.0, "Averaging time (min)"=0.0, "Extra Commands"="", "Carrier_1 Q (l/min)"=0.0, "Carrier_2 Q (l/min)"=0.0, "Trace Gas Concentration (%)"=0.0, "Specific Arguments"="1440.00", "Comments"="", "Row No"=0, "Row Type Selector"=enum."Wait (minutes)", "Completion time"="", "Row Duration (mins)"=0.0, "No. of Valid pts."=0, "Meas Setup File"="Current_Setup.xls"}, {"Start X"=0.0, "Start Y"=0.0, "Start Z"=0.0, "End X"=0.0, "End Y"=0.0, "End Z"=0.0, "No. of pts."=0, "Spacing"=enum."Linear", "Filename"=path "M:/\\Projects\\8773\\Results\\Tunnel1\\AnemometerSurvey.xls", "Tunnel Speed"=0.0, "Averaging time (min)"=0.0, "Extra Commands"="0.600", "Carrier_1 Q (l/min)"=0.0, "Carrier_2 Q (l/min)"=0.0, "Trace Gas Concentration (%)"=0.0, "Specific Arguments"="T1:Z:Corrections", "Comments"="", "Row No"=0, "Row Type Selector"=enum."Set ADAM Ch", "Completion time"="", "Row Duration (mins)"=0.0, "No. of Valid pts."=0, "Meas Setup File"="Current_Setup.xls"}, {"Start X"=-72.9, "Start Y"=-56.5, "Start Z"=13.3, "End X"=-72.9, "End Y"=-56.5, "End Z"=26.0, "No. of pts."=3, "Spacing"=enum."Specified", "Filename"=path "M:/\\Projects\\8773\\Results\\Tunnel1\\AnemometerSurvey.xls", "Tunnel Speed"=7.64, "Averaging time (min)"=1.0, "Extra Commands"="", "Carrier_1 Q (l/min)"=0.0, "Carrier_2 Q (l/min)"=0.0, "Trace Gas Concentration (%)"=0.0, "Specific Arguments"="Z= ;13.3;19.7;26.0\r", "Comments"="Anemo1", "Row No"=0, "Row Type Selector"=enum."Vertical Profile", "Completion time"="", "Row Duration (mins)"=0.0, "No. of Valid pts."=0, "Meas Setup File"="Current_Setup.xls"}, {"Start X"=0.0, "Start Y"=0.0, "Start Z"=0.0, "End X"=0.0, "End Y"=0.0, "End Z"=0.0, "No. of pts."=0, "Spacing"=enum."Linear", "Filename"=path "M:/\\Projects\\8773\\Results\\Tunnel1\\AnemometerSurvey.xls", "Tunnel Speed"=0.0, "Averaging time (min)"=0.0, "Extra Commands"="0.300", "Carrier_1 Q (l/min)"=0.0, "Carrier_2 Q (l/min)"=0.0, "Trace Gas Concentration (%)"=0.0, "Specific Arguments"="T1:Z:Corrections", "Comments"="", "Row No"=0, "Row Type Selector"=enum."Set ADAM Ch", "Completion time"="", "Row Duration (mins)"=0.0, "No. of Valid pts."=0, "Meas Setup File"="Current_Setup.xls"}, {"Start X"=-458.4, "Start Y"=87.9, "Start Z"=25.9, "End X"=-458.4, "End Y"=87.9, "End Z"=38.6, "No. of pts."=3, "Spacing"=enum."Specified", "Filename"=path "M:/\\Projects\\8773\\Results\\Tunnel1\\AnemometerSurvey.xls", "Tunnel Speed"=7.64, "Averaging time (min)"=1.0, "Extra Commands"="", "Carrier_1 Q (l/min)"=0.0, "Carrier_2 Q (l/min)"=0.0, "Trace Gas Concentration (%)"=0.0, "Specific Arguments"="Z= ;25.9;32.2;38.6\r", "Comments"="Anemo2", "Row No"=0, "Row Type Selector"=enum."Vertical Profile", "Completion time"="", "Row Duration (mins)"=0.0, "No. of Valid pts."=0, "Meas Setup File"="Current_Setup.xls"}, {"Start X"=0.0, "Start Y"=0.0, "Start Z"=150.0, "End X"=0.0, "End Y"=0.0, "End Z"=150.0, "No. of pts."=0, "Spacing"=enum."Linear", "Filename"=path "M:/\\Projects\\8773\\Results\\Tunnel1\\AnemometerSurvey.xls", "Tunnel Speed"=0.0, "Averaging time (min)"=0.0, "Extra Commands"="!Work in Tunnel Coordinates", "Carrier_1 Q (l/min)"=0.0, "Carrier_2 Q (l/min)"=0.0, "Trace Gas Concentration (%)"=0.0, "Specific Arguments"="", "Comments"="", "Row No"=0, "Row Type Selector"=enum."Move Traverse Only", "Completion time"="", "Row Duration (mins)"=0.0, "No. of Valid pts."=0, "Meas Setup File"="Current_Setup.xls"}, {"Start X"=0.0, "Start Y"=0.0, "Start Z"=0.0, "End X"=0.0, "End Y"=0.0, "End Z"=0.0, "No. of pts."=0, "Spacing"=enum."Linear", "Filename"=path "M:/\\Projects\\8773\\Results\\Tunnel1\\AnemometerSurvey.xls", "Tunnel Speed"=0.0, "Averaging time (min)"=0.0, "Extra Commands"="", "Carrier_1 Q (l/min)"=0.0, "Carrier_2 Q (l/min)"=0.0, "Trace Gas Concentration (%)"=0.0, "Specific Arguments"="", "Comments"="Time to set ramps...", "Row No"=0, "Row Type Selector"=enum."Send Message", "Completion time"="", "Row Duration (mins)"=0.0, "No. of Valid pts."=0, "Meas Setup File"="Current_Setup.xls"}, {"Start X"=0.0, "Start Y"=0.0, "Start Z"=0.0, "End X"=0.0, "End Y"=0.0, "End Z"=0.0, "No. of pts."=0, "Spacing"=enum."Linear", "Filename"=path "", "Tunnel Speed"=0.0, "Averaging time (min)"=0.0, "Extra Commands"="", "Carrier_1 Q (l/min)"=0.0, "Carrier_2 Q (l/min)"=0.0, "Trace Gas Concentration (%)"=0.0, "Specific Arguments"="", "Comments"="", "Row No"=0, "Row Type Selector"=enum."Blank Row", "Completion time"="", "Row Duration (mins)"=0.0, "No. of Valid pts."=0, "Meas Setup File"=""}, {"Start X"=0.0, "Start Y"=0.0, "Start Z"=0.0, "End X"=0.0, "End Y"=0.0, "End Z"=0.0, "No. of pts."=0, "Spacing"=enum."N/A", "Filename"=path "M:/\\Projects\\8773\\Results\\Tunnel1\\AnemometerSurvey.xls", "Tunnel Speed"=0.0, "Averaging time (min)"=0.0, "Extra Commands"="", "Carrier_1 Q (l/min)"=0.0, "Carrier_2 Q (l/min)"=0.0, "Trace Gas Concentration (%)"=0.0, "Specific Arguments"="MoveTT.vi;280", "Comments"="", "Row No"=0, "Row Type Selector"=enum."Run VI Named:", "Completion time"="", "Row Duration (mins)"=0.0, "No. of Valid pts."=0, "Meas Setup File"="Current_Setup.xls"}, {"Start X"=0.0, "Start Y"=0.0, "Start Z"=0.0, "End X"=0.0, "End Y"=0.0, "End Z"=0.0, "No. of pts."=0, "Spacing"=enum."Linear", "Filename"=path "M:/\\Projects\\8773\\Results\\Tunnel1\\AnemometerSurvey.xls", "Tunnel Speed"=0.0, "Averaging time (min)"=0.0, "Extra Commands"="", "Carrier_1 Q (l/min)"=0.0, "Carrier_2 Q (l/min)"=0.0, "Trace Gas Concentration (%)"=0.0, "Specific Arguments"="1440.00", "Comments"="", "Row No"=0, "Row Type Selector"=enum."Wait (minutes)", "Completion time"="", "Row Duration (mins)"=0.0, "No. of Valid pts."=0, "Meas Setup File"="Current_Setup.xls"}, {"Start X"=0.0, "Start Y"=0.0, "Start Z"=0.0, "End X"=0.0, "End Y"=0.0, "End Z"=0.0, "No. of pts."=0, "Spacing"=enum."Linear", "Filename"=path "M:/\\Projects\\8773\\Results\\Tunnel1\\AnemometerSurvey.xls", "Tunnel Speed"=0.0, "Averaging time (min)"=0.0, "Extra Commands"="0.300", "Carrier_1 Q (l/min)"=0.0, "Carrier_2 Q (l/min)"=0.0, "Trace Gas Concentration (%)"=0.0, "Specific Arguments"="T1:Z:Corrections", "Comments"="", "Row No"=0, "Row Type Selector"=enum."Set ADAM Ch", "Completion time"="", "Row Duration (mins)"=0.0, "No. of Valid pts."=0, "Meas Setup File"="Current_Setup.xls"}, {"Start X"=-72.9, "Start Y"=-56.5, "Start Z"=13.0, "End X"=-72.9, "End Y"=-56.5, "End Z"=25.7, "No. of pts."=3, "Spacing"=enum."Specified", "Filename"=path "M:/\\Projects\\8773\\Results\\Tunnel1\\AnemometerSurvey.xls", "Tunnel Speed"=7.64, "Averaging time (min)"=1.0, "Extra Commands"="", "Carrier_1 Q (l/min)"=0.0, "Carrier_2 Q (l/min)"=0.0, "Trace Gas Concentration (%)"=0.0, "Specific Arguments"="Z= ;13.0;19.3;25.7\r", "Comments"="Anemo1", "Row No"=0, "Row Type Selector"=enum."Vertical Profile", "Completion time"="", "Row Duration (mins)"=0.0, "No. of Valid pts."=0, "Meas Setup File"="Current_Setup.xls"}, {"Start X"=0.0, "Start Y"=0.0, "Start Z"=0.0, "End X"=0.0, "End Y"=0.0, "End Z"=0.0, "No. of pts."=0, "Spacing"=enum."Linear", "Filename"=path "M:/\\Projects\\8773\\Results\\Tunnel1\\AnemometerSurvey.xls", "Tunnel Speed"=0.0, "Averaging time (min)"=0.0, "Extra Commands"="0.900", "Carrier_1 Q (l/min)"=0.0, "Carrier_2 Q (l/min)"=0.0, "Trace Gas Concentration (%)"=0.0, "Specific Arguments"="T1:Z:Corrections", "Comments"="", "Row No"=0, "Row Type Selector"=enum."Set ADAM Ch", "Completion time"="", "Row Duration (mins)"=0.0, "No. of Valid pts."=0, "Meas Setup File"="Current_Setup.xls"}, {"Start X"=-458.4, "Start Y"=87.9, "Start Z"=26.5, "End X"=-458.4, "End Y"=87.9, "End Z"=39.2, "No. of pts."=3, "Spacing"=enum."Specified", "Filename"=path "M:/\\Projects\\8773\\Results\\Tunnel1\\AnemometerSurvey.xls", "Tunnel Speed"=7.64, "Averaging time (min)"=1.0, "Extra Commands"="", "Carrier_1 Q (l/min)"=0.0, "Carrier_2 Q (l/min)"=0.0, "Trace Gas Concentration (%)"=0.0, "Specific Arguments"="Z= ;26.5;32.8;39.2\r", "Comments"="Anemo2", "Row No"=0, "Row Type Selector"=enum."Vertical Profile", "Completion time"="", "Row Duration (mins)"=0.0, "No. of Valid pts."=0, "Meas Setup File"="Current_Setup.xls"}, {"Start X"=0.0, "Start Y"=0.0, "Start Z"=150.0, "End X"=0.0, "End Y"=0.0, "End Z"=150.0, "No. of pts."=0, "Spacing"=enum."Linear", "Filename"=path "M:/\\Projects\\8773\\Results\\Tunnel1\\AnemometerSurvey.xls", "Tunnel Speed"=0.0, "Averaging time (min)"=0.0, "Extra Commands"="!Work in Tunnel Coordinates", "Carrier_1 Q (l/min)"=0.0, "Carrier_2 Q (l/min)"=0.0, "Trace Gas Concentration (%)"=0.0, "Specific Arguments"="", "Comments"="", "Row No"=0, "Row Type Selector"=enum."Move Traverse Only", "Completion time"="", "Row Duration (mins)"=0.0, "No. of Valid pts."=0, "Meas Setup File"="Current_Setup.xls"}, {"Start X"=0.0, "Start Y"=0.0, "Start Z"=0.0, "End X"=0.0, "End Y"=0.0, "End Z"=0.0, "No. of pts."=0, "Spacing"=enum."Linear", "Filename"=path "M:/\\Projects\\8773\\Results\\Tunnel1\\AnemometerSurvey.xls", "Tunnel Speed"=0.0, "Averaging time (min)"=0.0, "Extra Commands"="", "Carrier_1 Q (l/min)"=0.0, "Carrier_2 Q (l/min)"=0.0, "Trace Gas Concentration (%)"=0.0, "Specific Arguments"="", "Comments"="Time to set ramps...", "Row No"=0, "Row Type Selector"=enum."Send Message", "Completion time"="", "Row Duration (mins)"=0.0, "No. of Valid pts."=0, "Meas Setup File"="Current_Setup.xls"}, {"Start X"=0.0, "Start Y"=0.0, "Start Z"=0.0, "End X"=0.0, "End Y"=0.0, "End Z"=0.0, "No. of pts."=0, "Spacing"=enum."Linear", "Filename"=path "", "Tunnel Speed"=0.0, "Averaging time (min)"=0.0, "Extra Commands"="", "Carrier_1 Q (l/min)"=0.0, "Carrier_2 Q (l/min)"=0.0, "Trace Gas Concentration (%)"=0.0, "Specific Arguments"="", "Comments"="", "Row No"=0, "Row Type Selector"=enum."Blank Row", "Completion time"="", "Row Duration (mins)"=0.0, "No. of Valid pts."=0, "Meas Setup File"=""}, {"Start X"=0.0, "Start Y"=0.0, "Start Z"=780.0, "End X"=0.0, "End Y"=0.0, "End Z"=780.0, "No. of pts."=0, "Spacing"=enum."Linear", "Filename"=path "M:/\\Projects\\8773\\Results\\Tunnel1\\AnemometerSurvey.xls", "Tunnel Speed"=7.64, "Averaging time (min)"=1.0, "Extra Commands"="!Work in Tunnel Coordinates", "Carrier_1 Q (l/min)"=0.0, "Carrier_2 Q (l/min)"=0.0, "Trace Gas Concentration (%)"=0.0, "Specific Arguments"="", "Comments"="LocalCalCheck", "Row No"=0, "Row Type Selector"=enum."Single Measurement", "Completion time"="", "Row Duration (mins)"=0.0, "No. of Valid pts."=0, "Meas Setup File"="Current_Setup.xls"}, {"Start X"=0.0, "Start Y"=0.0, "Start Z"=0.0, "End X"=0.0, "End Y"=0.0, "End Z"=0.0, "No. of pts."=0, "Spacing"=enum."N/A", "Filename"=path "M:/\\Projects\\8773\\Results\\Tunnel1\\AnemometerSurvey.xls", "Tunnel Speed"=0.0, "Averaging time (min)"=0.0, "Extra Commands"="", "Carrier_1 Q (l/min)"=0.0, "Carrier_2 Q (l/min)"=0.0, "Trace Gas Concentration (%)"=0.0, "Specific Arguments"="MoveTT.vi;300", "Comments"="", "Row No"=0, "Row Type Selector"=enum."Run VI Named:", "Completion time"="", "Row Duration (mins)"=0.0, "No. of Valid pts."=0, "Meas Setup File"="Current_Setup.xls"}, {"Start X"=0.0, "Start Y"=0.0, "Start Z"=0.0, "End X"=0.0, "End Y"=0.0, "End Z"=0.0, "No. of pts."=0, "Spacing"=enum."Linear", "Filename"=path "M:/\\Projects\\8773\\Results\\Tunnel1\\AnemometerSurvey.xls", "Tunnel Speed"=0.0, "Averaging time (min)"=0.0, "Extra Commands"="", "Carrier_1 Q (l/min)"=0.0, "Carrier_2 Q (l/min)"=0.0, "Trace Gas Concentration (%)"=0.0, "Specific Arguments"="1440.00", "Comments"="", "Row No"=0, "Row Type Selector"=enum."Wait (minutes)", "Completion time"="", "Row Duration (mins)"=0.0, "No. of Valid pts."=0, "Meas Setup File"="Current_Setup.xls"}, {"Start X"=0.0, "Start Y"=0.0, "Start Z"=0.0, "End X"=0.0, "End Y"=0.0, "End Z"=0.0, "No. of pts."=0, "Spacing"=enum."Linear", "Filename"=path "M:/\\Projects\\8773\\Results\\Tunnel1\\AnemometerSurvey.xls", "Tunnel Speed"=0.0, "Averaging time (min)"=0.0, "Extra Commands"="0.800", "Carrier_1 Q (l/min)"=0.0, "Carrier_2 Q (l/min)"=0.0, "Trace Gas Concentration (%)"=0.0, "Specific Arguments"="T1:Z:Corrections", "Comments"="", "Row No"=0, "Row Type Selector"=enum."Set ADAM Ch", "Completion time"="", "Row Duration (mins)"=0.0, "No. of Valid pts."=0, "Meas Setup File"="Current_Setup.xls"}, {"Start X"=-72.9, "Start Y"=-56.5, "Start Z"=13.5, "End X"=-72.9, "End Y"=-56.5, "End Z"=26.2, "No. of pts."=3, "Spacing"=enum."Specified", "Filename"=path "M:/\\Projects\\8773\\Results\\Tunnel1\\AnemometerSurvey.xls", "Tunnel Speed"=7.64, "Averaging time (min)"=1.0, "Extra Commands"="", "Carrier_1 Q (l/min)"=0.0, "Carrier_2 Q (l/min)"=0.0, "Trace Gas Concentration (%)"=0.0, "Specific Arguments"="Z= ;13.5;19.8;26.2\r", "Comments"="Anemo1", "Row No"=0, "Row Type Selector"=enum."Vertical Profile", "Completion time"="", "Row Duration (mins)"=0.0, "No. of Valid pts."=0, "Meas Setup File"="Current_Setup.xls"}, {"Start X"=0.0, "Start Y"=0.0, "Start Z"=0.0, "End X"=0.0, "End Y"=0.0, "End Z"=0.0, "No. of pts."=0, "Spacing"=enum."Linear", "Filename"=path "M:/\\Projects\\8773\\Results\\Tunnel1\\AnemometerSurvey.xls", "Tunnel Speed"=0.0, "Averaging time (min)"=0.0, "Extra Commands"="1.800", "Carrier_1 Q (l/min)"=0.0, "Carrier_2 Q (l/min)"=0.0, "Trace Gas Concentration (%)"=0.0, "Specific Arguments"="T1:Z:Corrections", "Comments"="", "Row No"=0, "Row Type Selector"=enum."Set ADAM Ch", "Completion time"="", "Row Duration (mins)"=0.0, "No. of Valid pts."=0, "Meas Setup File"="Current_Setup.xls"}, {"Start X"=-458.4, "Start Y"=87.9, "Start Z"=27.4, "End X"=-458.4, "End Y"=87.9, "End Z"=40.1, "No. of pts."=3, "Spacing"=enum."Specified", "Filename"=path "M:/\\Projects\\8773\\Results\\Tunnel1\\AnemometerSurvey.xls", "Tunnel Speed"=7.64, "Averaging time (min)"=1.0, "Extra Commands"="", "Carrier_1 Q (l/min)"=0.0, "Carrier_2 Q (l/min)"=0.0, "Trace Gas Concentration (%)"=0.0, "Specific Arguments"="Z= ;27.4;33.8;40.1\r", "Comments"="Anemo2", "Row No"=0, "Row Type Selector"=enum."Vertical Profile", "Completion time"="", "Row Duration (mins)"=0.0, "No. of Valid pts."=0, "Meas Setup File"="Current_Setup.xls"}, {"Start X"=0.0, "Start Y"=0.0, "Start Z"=150.0, "End X"=0.0, "End Y"=0.0, "End Z"=150.0, "No. of pts."=0, "Spacing"=enum."Linear", "Filename"=path "M:/\\Projects\\8773\\Results\\Tunnel1\\AnemometerSurvey.xls", "Tunnel Speed"=0.0, "Averaging time (min)"=0.0, "Extra Commands"="!Work in Tunnel Coordinates", "Carrier_1 Q (l/min)"=0.0, "Carrier_2 Q (l/min)"=0.0, "Trace Gas Concentration (%)"=0.0, "Specific Arguments"="", "Comments"="", "Row No"=0, "Row Type Selector"=enum."Move Traverse Only", "Completion time"="", "Row Duration (mins)"=0.0, "No. of Valid pts."=0, "Meas Setup File"="Current_Setup.xls"}, {"Start X"=0.0, "Start Y"=0.0, "Start Z"=0.0, "End X"=0.0, "End Y"=0.0, "End Z"=0.0, "No. of pts."=0, "Spacing"=enum."Linear", "Filename"=path "M:/\\Projects\\8773\\Results\\Tunnel1\\AnemometerSurvey.xls", "Tunnel Speed"=0.0, "Averaging time (min)"=0.0, "Extra Commands"="", "Carrier_1 Q (l/min)"=0.0, "Carrier_2 Q (l/min)"=0.0, "Trace Gas Concentration (%)"=0.0, "Specific Arguments"="", "Comments"="Time to set ramps...", "Row No"=0, "Row Type Selector"=enum."Send Message", "Completion time"="", "Row Duration (mins)"=0.0, "No. of Valid pts."=0, "Meas Setup File"="Current_Setup.xls"}, {"Start X"=0.0, "Start Y"=0.0, "Start Z"=0.0, "End X"=0.0, "End Y"=0.0, "End Z"=0.0, "No. of pts."=0, "Spacing"=enum."Linear", "Filename"=path "", "Tunnel Speed"=0.0, "Averaging time (min)"=0.0, "Extra Commands"="", "Carrier_1 Q (l/min)"=0.0, "Carrier_2 Q (l/min)"=0.0, "Trace Gas Concentration (%)"=0.0, "Specific Arguments"="", "Comments"="", "Row No"=0, "Row Type Selector"=enum."Blank Row", "Completion time"="", "Row Duration (mins)"=0.0, "No. of Valid pts."=0, "Meas Setup File"=""}, {"Start X"=0.0, "Start Y"=0.0, "Start Z"=0.0, "End X"=0.0, "End Y"=0.0, "End Z"=0.0, "No. of pts."=0, "Spacing"=enum."N/A", "Filename"=path "M:/\\Projects\\8773\\Results\\Tunnel1\\AnemometerSurvey.xls", "Tunnel Speed"=0.0, "Averaging time (min)"=0.0, "Extra Commands"="", "Carrier_1 Q (l/min)"=0.0, "Carrier_2 Q (l/min)"=0.0, "Trace Gas Concentration (%)"=0.0, "Specific Arguments"="MoveTT.vi;320", "Comments"="", "Row No"=0, "Row Type Selector"=enum."Run VI Named:", "Completion time"="", "Row Duration (mins)"=0.0, "No. of Valid pts."=0, "Meas Setup File"="Current_Setup.xls"}, {"Start X"=0.0, "Start Y"=0.0, "Start Z"=0.0, "End X"=0.0, "End Y"=0.0, "End Z"=0.0, "No. of pts."=0, "Spacing"=enum."Linear", "Filename"=path "M:/\\Projects\\8773\\Results\\Tunnel1\\AnemometerSurvey.xls", "Tunnel Speed"=0.0, "Averaging time (min)"=0.0, "Extra Commands"="", "Carrier_1 Q (l/min)"=0.0, "Carrier_2 Q (l/min)"=0.0, "Trace Gas Concentration (%)"=0.0, "Specific Arguments"="1440.00", "Comments"="", "Row No"=0, "Row Type Selector"=enum."Wait (minutes)", "Completion time"="", "Row Duration (mins)"=0.0, "No. of Valid pts."=0, "Meas Setup File"="Current_Setup.xls"}, {"Start X"=0.0, "Start Y"=0.0, "Start Z"=0.0, "End X"=0.0, "End Y"=0.0, "End Z"=0.0, "No. of pts."=0, "Spacing"=enum."Linear", "Filename"=path "M:/\\Projects\\8773\\Results\\Tunnel1\\AnemometerSurvey.xls", "Tunnel Speed"=0.0, "Averaging time (min)"=0.0, "Extra Commands"="0.700", "Carrier_1 Q (l/min)"=0.0, "Carrier_2 Q (l/min)"=0.0, "Trace Gas Concentration (%)"=0.0, "Specific Arguments"="T1:Z:Corrections", "Comments"="", "Row No"=0, "Row Type Selector"=enum."Set ADAM Ch", "Completion time"="", "Row Duration (mins)"=0.0, "No. of Valid pts."=0, "Meas Setup File"="Current_Setup.xls"}, {"Start X"=-72.9, "Start Y"=-56.5, "Start Z"=13.4, "End X"=-72.9, "End Y"=-56.5, "End Z"=26.1, "No. of pts."=3, "Spacing"=enum."Specified", "Filename"=path "M:/\\Projects\\8773\\Results\\Tunnel1\\AnemometerSurvey.xls", "Tunnel Speed"=7.64, "Averaging time (min)"=1.0, "Extra Commands"="", "Carrier_1 Q (l/min)"=0.0, "Carrier_2 Q (l/min)"=0.0, "Trace Gas Concentration (%)"=0.0, "Specific Arguments"="Z= ;13.4;19.8;26.1\r", "Comments"="Anemo1", "Row No"=0, "Row Type Selector"=enum."Vertical Profile", "Completion time"="", "Row Duration (mins)"=0.0, "No. of Valid pts."=0, "Meas Setup File"="Current_Setup.xls"}, {"Start X"=0.0, "Start Y"=0.0, "Start Z"=0.0, "End X"=0.0, "End Y"=0.0, "End Z"=0.0, "No. of pts."=0, "Spacing"=enum."Linear", "Filename"=path "M:/\\Projects\\8773\\Results\\Tunnel1\\AnemometerSurvey.xls", "Tunnel Speed"=0.0, "Averaging time (min)"=0.0, "Extra Commands"="2.200", "Carrier_1 Q (l/min)"=0.0, "Carrier_2 Q (l/min)"=0.0, "Trace Gas Concentration (%)"=0.0, "Specific Arguments"="T1:Z:Corrections", "Comments"="", "Row No"=0, "Row Type Selector"=enum."Set ADAM Ch", "Completion time"="", "Row Duration (mins)"=0.0, "No. of Valid pts."=0, "Meas Setup File"="Current_Setup.xls"}, {"Start X"=-458.4, "Start Y"=87.9, "Start Z"=27.8, "End X"=-458.4, "End Y"=87.9, "End Z"=40.5, "No. of pts."=3, "Spacing"=enum."Specified", "Filename"=path "M:/\\Projects\\8773\\Results\\Tunnel1\\AnemometerSurvey.xls", "Tunnel Speed"=7.64, "Averaging time (min)"=1.0, "Extra Commands"="", "Carrier_1 Q (l/min)"=0.0, "Carrier_2 Q (l/min)"=0.0, "Trace Gas Concentration (%)"=0.0, "Specific Arguments"="Z= ;27.8;34.2;40.5\r", "Comments"="Anemo2", "Row No"=0, "Row Type Selector"=enum."Vertical Profile", "Completion time"="", "Row Duration (mins)"=0.0, "No. of Valid pts."=0, "Meas Setup File"="Current_Setup.xls"}, {"Start X"=0.0, "Start Y"=0.0, "Start Z"=150.0, "End X"=0.0, "End Y"=0.0, "End Z"=150.0, "No. of pts."=0, "Spacing"=enum."Linear", "Filename"=path "M:/\\Projects\\8773\\Results\\Tunnel1\\AnemometerSurvey.xls", "Tunnel Speed"=0.0, "Averaging time (min)"=0.0, "Extra Commands"="!Work in Tunnel Coordinates", "Carrier_1 Q (l/min)"=0.0, "Carrier_2 Q (l/min)"=0.0, "Trace Gas Concentration (%)"=0.0, "Specific Arguments"="", "Comments"="", "Row No"=0, "Row Type Selector"=enum."Move Traverse Only", "Completion time"="", "Row Duration (mins)"=0.0, "No. of Valid pts."=0, "Meas Setup File"="Current_Setup.xls"}, {"Start X"=0.0, "Start Y"=0.0, "Start Z"=0.0, "End X"=0.0, "End Y"=0.0, "End Z"=0.0, "No. of pts."=0, "Spacing"=enum."Linear", "Filename"=path "M:/\\Projects\\8773\\Results\\Tunnel1\\AnemometerSurvey.xls", "Tunnel Speed"=0.0, "Averaging time (min)"=0.0, "Extra Commands"="", "Carrier_1 Q (l/min)"=0.0, "Carrier_2 Q (l/min)"=0.0, "Trace Gas Concentration (%)"=0.0, "Specific Arguments"="", "Comments"="Time to set ramps...", "Row No"=0, "Row Type Selector"=enum."Send Message", "Completion time"="", "Row Duration (mins)"=0.0, "No. of Valid pts."=0, "Meas Setup File"="Current_Setup.xls"}, {"Start X"=0.0, "Start Y"=0.0, "Start Z"=0.0, "End X"=0.0, "End Y"=0.0, "End Z"=0.0, "No. of pts."=0, "Spacing"=enum."Linear", "Filename"=path "", "Tunnel Speed"=0.0, "Averaging time (min)"=0.0, "Extra Commands"="", "Carrier_1 Q (l/min)"=0.0, "Carrier_2 Q (l/min)"=0.0, "Trace Gas Concentration (%)"=0.0, "Specific Arguments"="", "Comments"="", "Row No"=0, "Row Type Selector"=enum."Blank Row", "Completion time"="", "Row Duration (mins)"=0.0, "No. of Valid pts."=0, "Meas Setup File"=""}, {"Start X"=0.0, "Start Y"=0.0, "Start Z"=0.0, "End X"=0.0, "End Y"=0.0, "End Z"=0.0, "No. of pts."=0, "Spacing"=enum."N/A", "Filename"=path "M:/\\Projects\\8773\\Results\\Tunnel1\\AnemometerSurvey.xls", "Tunnel Speed"=0.0, "Averaging time (min)"=0.0, "Extra Commands"="", "Carrier_1 Q (l/min)"=0.0, "Carrier_2 Q (l/min)"=0.0, "Trace Gas Concentration (%)"=0.0, "Specific Arguments"="MoveTT.vi;340", "Comments"="", "Row No"=0, "Row Type Selector"=enum."Run VI Named:", "Completion time"="", "Row Duration (mins)"=0.0, "No. of Valid pts."=0, "Meas Setup File"="Current_Setup.xls"}, {"Start X"=0.0, "Start Y"=0.0, "Start Z"=0.0, "End X"=0.0, "End Y"=0.0, "End Z"=0.0, "No. of pts."=0, "Spacing"=enum."Linear", "Filename"=path "M:/\\Projects\\8773\\Results\\Tunnel1\\AnemometerSurvey.xls", "Tunnel Speed"=0.0, "Averaging time (min)"=0.0, "Extra Commands"="", "Carrier_1 Q (l/min)"=0.0, "Carrier_2 Q (l/min)"=0.0, "Trace Gas Concentration (%)"=0.0, "Specific Arguments"="1440.00", "Comments"="", "Row No"=0, "Row Type Selector"=enum."Wait (minutes)", "Completion time"="", "Row Duration (mins)"=0.0, "No. of Valid pts."=0, "Meas Setup File"="Current_Setup.xls"}, {"Start X"=0.0, "Start Y"=0.0, "Start Z"=0.0, "End X"=0.0, "End Y"=0.0, "End Z"=0.0, "No. of pts."=0, "Spacing"=enum."Linear", "Filename"=path "M:/\\Projects\\8773\\Results\\Tunnel1\\AnemometerSurvey.xls", "Tunnel Speed"=0.0, "Averaging time (min)"=0.0, "Extra Commands"="-0.000", "Carrier_1 Q (l/min)"=0.0, "Carrier_2 Q (l/min)"=0.0, "Trace Gas Concentration (%)"=0.0, "Specific Arguments"="T1:Z:Corrections", "Comments"="", "Row No"=0, "Row Type Selector"=enum."Set ADAM Ch", "Completion time"="", "Row Duration (mins)"=0.0, "No. of Valid pts."=0, "Meas Setup File"="Current_Setup.xls"}, {"Start X"=-72.9, "Start Y"=-56.5, "Start Z"=12.7, "End X"=-72.9, "End Y"=-56.5, "End Z"=25.4, "No. of pts."=3, "Spacing"=enum."Specified", "Filename"=path "M:/\\Projects\\8773\\Results\\Tunnel1\\AnemometerSurvey.xls", "Tunnel Speed"=7.64, "Averaging time (min)"=1.0, "Extra Commands"="", "Carrier_1 Q (l/min)"=0.0, "Carrier_2 Q (l/min)"=0.0, "Trace Gas Concentration (%)"=0.0, "Specific Arguments"="Z= ;12.7;19.1;25.4\r", "Comments"="Anemo1", "Row No"=0, "Row Type Selector"=enum."Vertical Profile", "Completion time"="", "Row Duration (mins)"=0.0, "No. of Valid pts."=0, "Meas Setup File"="Current_Setup.xls"}, {"Start X"=0.0, "Start Y"=0.0, "Start Z"=0.0, "End X"=0.0, "End Y"=0.0, "End Z"=0.0, "No. of pts."=0, "Spacing"=enum."Linear", "Filename"=path "M:/\\Projects\\8773\\Results\\Tunnel1\\AnemometerSurvey.xls", "Tunnel Speed"=0.0, "Averaging time (min)"=0.0, "Extra Commands"="1.200", "Carrier_1 Q (l/min)"=0.0, "Carrier_2 Q (l/min)"=0.0, "Trace Gas Concentration (%)"=0.0, "Specific Arguments"="T1:Z:Corrections", "Comments"="", "Row No"=0, "Row Type Selector"=enum."Set ADAM Ch", "Completion time"="", "Row Duration (mins)"=0.0, "No. of Valid pts."=0, "Meas Setup File"="Current_Setup.xls"}, {"Start X"=-458.4, "Start Y"=87.9, "Start Z"=26.8, "End X"=-458.4, "End Y"=87.9, "End Z"=39.5, "No. of pts."=3, "Spacing"=enum."Specified", "Filename"=path "M:/\\Projects\\8773\\Results\\Tunnel1\\AnemometerSurvey.xls", "Tunnel Speed"=7.64, "Averaging time (min)"=1.0, "Extra Commands"="", "Carrier_1 Q (l/min)"=0.0, "Carrier_2 Q (l/min)"=0.0, "Trace Gas Concentration (%)"=0.0, "Specific Arguments"="Z= ;26.8;33.2;39.5\r", "Comments"="Anemo2", "Row No"=0, "Row Type Selector"=enum."Vertical Profile", "Completion time"="", "Row Duration (mins)"=0.0, "No. of Valid pts."=0, "Meas Setup File"="Current_Setup.xls"}, {"Start X"=0.0, "Start Y"=0.0, "Start Z"=150.0, "End X"=0.0, "End Y"=0.0, "End Z"=150.0, "No. of pts."=0, "Spacing"=enum."Linear", "Filename"=path "M:/\\Projects\\8773\\Results\\Tunnel1\\AnemometerSurvey.xls", "Tunnel Speed"=0.0, "Averaging time (min)"=0.0, "Extra Commands"="!Work in Tunnel Coordinates", "Carrier_1 Q (l/min)"=0.0, "Carrier_2 Q (l/min)"=0.0, "Trace Gas Concentration (%)"=0.0, "Specific Arguments"="", "Comments"="", "Row No"=0, "Row Type Selector"=enum."Move Traverse Only", "Completion time"="", "Row Duration (mins)"=0.0, "No. of Valid pts."=0, "Meas Setup File"="Current_Setup.xls"}, {"Start X"=0.0, "Start Y"=0.0, "Start Z"=0.0, "End X"=0.0, "End Y"=0.0, "End Z"=0.0, "No. of pts."=0, "Spacing"=enum."Linear", "Filename"=path "M:/\\Projects\\8773\\Results\\Tunnel1\\AnemometerSurvey.xls", "Tunnel Speed"=0.0, "Averaging time (min)"=0.0, "Extra Commands"="", "Carrier_1 Q (l/min)"=0.0, "Carrier_2 Q (l/min)"=0.0, "Trace Gas Concentration (%)"=0.0, "Specific Arguments"="", "Comments"="Time to set ramps...", "Row No"=0, "Row Type Selector"=enum."Send Message", "Completion time"="", "Row Duration (mins)"=0.0, "No. of Valid pts."=0, "Meas Setup File"="Current_Setup.xls"}, {"Start X"=0.0, "Start Y"=0.0, "Start Z"=0.0, "End X"=0.0, "End Y"=0.0, "End Z"=0.0, "No. of pts."=0, "Spacing"=enum."Linear", "Filename"=path "", "Tunnel Speed"=0.0, "Averaging time (min)"=0.0, "Extra Commands"="", "Carrier_1 Q (l/min)"=0.0, "Carrier_2 Q (l/min)"=0.0, "Trace Gas Concentration (%)"=0.0, "Specific Arguments"="", "Comments"="", "Row No"=0, "Row Type Selector"=enum."Blank Row", "Completion time"="", "Row Duration (mins)"=0.0, "No. of Valid pts."=0, "Meas Setup File"=""}, {"Start X"=0.0, "Start Y"=0.0, "Start Z"=0.0, "End X"=0.0, "End Y"=0.0, "End Z"=0.0, "No. of pts."=0, "Spacing"=enum."N/A", "Filename"=path "M:/\\Projects\\8773\\Results\\Tunnel1\\AnemometerSurvey.xls", "Tunnel Speed"=0.0, "Averaging time (min)"=0.0, "Extra Commands"="", "Carrier_1 Q (l/min)"=0.0, "Carrier_2 Q (l/min)"=0.0, "Trace Gas Concentration (%)"=0.0, "Specific Arguments"="MoveTT.vi;0", "Comments"="", "Row No"=0, "Row Type Selector"=enum."Run VI Named:", "Completion time"="", "Row Duration (mins)"=0.0, "No. of Valid pts."=0, "Meas Setup File"="Current_Setup.xls"}, {"Start X"=-3390.0, "Start Y"=-113.0, "Start Z"=780.0, "End X"=-3390.0, "End Y"=-113.0, "End Z"=780.0, "No. of pts."=0, "Spacing"=enum."Linear", "Filename"=path "M:/\\Projects\\8773\\Results\\Tunnel1\\AnemometerSurvey.xls", "Tunnel Speed"=0.0, "Averaging time (min)"=1.0, "Extra Commands"="!Work in Tunnel Coordinates", "Carrier_1 Q (l/min)"=0.0, "Carrier_2 Q (l/min)"=0.0, "Trace Gas Concentration (%)"=0.0, "Specific Arguments"="", "Comments"="Zeroes", "Row No"=0, "Row Type Selector"=enum."Single Measurement", "Completion time"="", "Row Duration (mins)"=0.0, "No. of Valid pts."=0, "Meas Setup File"="Current_Setup.xls"}, {"Start X"=-3390.0, "Start Y"=-113.0, "Start Z"=780.0, "End X"=-3390.0, "End Y"=-113.0, "End Z"=780.0, "No. of pts."=0, "Spacing"=enum."Linear", "Filename"=path "M:/\\Projects\\8773\\Results\\Tunnel1\\AnemometerSurvey.xls", "Tunnel Speed"=7.64, "Averaging time (min)"=1.0, "Extra Commands"="!Work in Tunnel Coordinates", "Carrier_1 Q (l/min)"=0.0, "Carrier_2 Q (l/min)"=0.0, "Trace Gas Concentration (%)"=0.0, "Specific Arguments"="", "Comments"="CalCheck", "Row No"=0, "Row Type Selector"=enum."Single Measurement", "Completion time"="", "Row Duration (mins)"=0.0, "No. of Valid pts."=0, "Meas Setup File"="Current_Setup.xls"}, {"Start X"=0.0, "Start Y"=0.0, "Start Z"=780.0, "End X"=0.0, "End Y"=0.0, "End Z"=780.0, "No. of pts."=0, "Spacing"=enum."Linear", "Filename"=path "M:/\\Projects\\8773\\Results\\Tunnel1\\AnemometerSurvey.xls", "Tunnel Speed"=7.64, "Averaging time (min)"=1.0, "Extra Commands"="!Work in Tunnel Coordinates", "Carrier_1 Q (l/min)"=0.0, "Carrier_2 Q (l/min)"=0.0, "Trace Gas Concentration (%)"=0.0, "Specific Arguments"="", "Comments"="LocalCalCheck", "Row No"=0, "Row Type Selector"=enum."Single Measurement", "Completion time"="", "Row Duration (mins)"=0.0, "No. of Valid pts."=0, "Meas Setup File"="Current_Setup.xls"}, {"Start X"=0.0, "Start Y"=0.0, "Start Z"=0.0, "End X"=0.0, "End Y"=0.0, "End Z"=0.0, "No. of pts."=0, "Spacing"=enum."Linear", "Filename"=path "M:/\\Projects\\8773\\Results\\Tunnel1\\AnemometerSurvey.xls", "Tunnel Speed"=0.0, "Averaging time (min)"=0.0, "Extra Commands"="", "Carrier_1 Q (l/min)"=0.0, "Carrier_2 Q (l/min)"=0.0, "Trace Gas Concentration (%)"=0.0, "Specific Arguments"="", "Comments"="Tunnel Off", "Row No"=0, "Row Type Selector"=enum."Set Tunnel Speed Only", "Completion time"="", "Row Duration (mins)"=0.0, "No. of Valid pts."=0, "Meas Setup File"="Current_Setup.xls"}] {"Carrier_2 Q (l/min)" format="%#.2f"; "Row Duration (mins)" format="%#.1f"; "Row No" min=0; "Trace Gas Concentration (%)" min=0.0 format="%#_4f"; "Carrier_1 Q (l/min)" format="%#.2f"; "Tunnel Speed" format="%#.2f"; "Start X" format="%#.2f"; "Start Y" format="%#.2f"; "Start Z" format="%#.2f"; "End X" format="%#.2f"; "End Y" format="%#.2f"; "End Z" format="%#.2f"; "Averaging time (min)" min=0.0 format="%#.2f"}
  in  "Tab Control":T4(tab)=enum."Single Measurements"
  in  "Jump Bad Positions":bool
  in  "Work in TUNNEL Coordinates":bool
  in  "Command File Path / Name":path=path "/CentralDataCache/Projects/9999/Commands/Post_Processing_Machine/AnemometerSurveyTEST.xls"
  in  "Results File Path / Name":path=path "M:/\\Projects\\8773\\Results\\Tunnel1\\AnemometerSurvey.xls"
  in  "Setup:":string(combo)="Current_Setup.xls"
  in  "Tunnel Warmup (min)":dbl=10.0
  in  "Velocity (m/s)":dbl=7.64
  in  "Measure (seconds)":dbl=60.0
  out "Measure (mins)":dbl=1.0
  in  "Multirun Closure Tasks":T5={"Turn Table --> Zero"=TRUE, "AutoCal"=FALSE, "Zeroes"=TRUE, "Global Cal Checks"=TRUE, "Local Cal Checks"=TRUE, "Tunnel Off"=TRUE}
  in  "Task Selection":T6={"Tunnel Warm Up"=TRUE, "AutoCal"=FALSE, "Zeroes"=TRUE, "Turn Table Schedule"=TRUE, "Global Cal Checks"=TRUE, "Local Cal Checks"=TRUE, "Vertical Profile"=TRUE, "Lateral Profile"=FALSE, "Reinitialize Task Array"=TRUE, "Save Command File"=TRUE, "Longitudinal Profile"=FALSE}
  in  "Autocal.TunnelSpeeds":dbl[](array[numeric])=[2.18, 3.06, 4.37, 5.68, 7.86, 10.26, 13.1]
  in  "SpeedSettings":dbl[](array[numeric])
  in  "SingleMeasurement.Coords":T7(array[cluster])
  in  "Zeroes":T8={"X"=-3390.0, "Y"=-113.0, "Z"=780.0, "Use Tunnel Coords?"=TRUE, "RepeatEveryXDeg"=120.0}
  in  "Local Calcheck":T9={"X"=0.0, "Y"=0.0, "Z"=780.0, "Use Tunnel Coords? Coords"=TRUE, "RepeatEveryXDeg"=60.0}
  in  "Global Calcheck":T8={"X"=-3390.0, "Y"=-113.0, "Z"=780.0, "Use Tunnel Coords?"=TRUE, "RepeatEveryXDeg"=120.0}
  in  "Calculate TT Array":bool=TRUE
  in  "Angle Increment":dbl=20.0
  in  "Ending Angle":dbl=340.0
  in  "Starting Angle":dbl
  in  "Azimuth Values":dbl[](array[numeric])=[0.0, 20.0, 40.0, 60.0, 80.0, 100.0, 120.0, 140.0, 160.0, 180.0, 200.0, 220.0, 240.0, 260.0, 280.0, 300.0, 320.0, 340.0]
  in  "Build-A-Block":T11(array[cluster])=[{"Row Type Selector"=enum."Longitudinal Profile", "Index"=0.0, "Direction"=enum."Forward"}, {"Row Type Selector"=enum."Longitudinal Profile", "Index"=1.0, "Direction"=enum."Reverse"}]
  in  "VertProf.Coords":T12(array[cluster])=[{"X"=-72.9, "Y"=-56.5, "Z0"=0.0, "Name"="Anemo1", "Spacing"=enum."Specified", "Z.start"=45.0, "Z.end"=45.0, "NumPts"=0.0}, {"X"=-458.4, "Y"=87.9, "Z0"=12.9, "Name"="Anemo2", "Spacing"=enum."Specified", "Z.start"=45.0, "Z.end"=45.0, "NumPts"=0.0}]
  in  "Vert.Z-Locations":dbl[](array[numeric])=[12.7, 19.05, 25.4]
  in  "VP.TTHeightCorrs":T13={"TT.Azimuths"=[0.0, 20.0, 40.0, 60.0, 80.0, 100.0, 120.0, 140.0, 160.0, 180.0, 200.0, 220.0, 240.0, 260.0, 280.0, 300.0, 320.0, 340.0], "Z.HeightCorrs"=[[-0.0, -0.0], [-0.5, -1.4000000000000057], [-1.0, -3.1000000000000085], [-0.5, -4.1000000000000085], [-0.7999999999999972, -4.900000000000006], [-0.8999999999999915, -5.6000000000000085], [-0.3999999999999915, -5.5], [0.10000000000000853, -5.1000000000000085], [0.10000000000000853, -4.700000000000003], [0.5, -3.9000000000000057], [0.6000000000000085, -2.700000000000003], [0.10000000000000853, -2.1000000000000085], [0.6000000000000085, -0.9000000000000057], [0.6000000000000085, 0.29999999999999716], [0.29999999999999716, 0.8999999999999915], [0.7999999999999972, 1.7999999999999972], [0.7000000000000028, 2.200000000000003], [-0.0, 1.2000000000000028]], "Use Height Corrections"=TRUE, "Height Survey Filepaths"=[path "/CentralDataCache/Projects/8773/Results/Tunnel1/Height Survey & Corrections/Zsurvey-Anemo1.xls", path "/CentralDataCache/Projects/8773/Results/Tunnel1/Height Survey & Corrections/Zsurvey-Anemo2.xls"], "Corrections from File"=TRUE}
  in  "Correction Channel Name":string="T1:Z:Corrections"
  in  "LatProf.Coords":T14(array[cluster])=[{"X"=-1900.0, "Y0"=-500.0, "Z"=229.0, "Name"="TTLE", "Spacing"=enum."Linear", "Y.start"=-500.0, "Y.end"=500.0, "NumPts"=11.0}, {"X"=0.0, "Y0"=-500.0, "Z"=229.0, "Name"="TTC", "Spacing"=enum."Specified", "Y.start"=-500.0, "Y.end"=500.0, "NumPts"=12.0}, {"X"=1475.0, "Y0"=-500.0, "Z"=229.0, "Name"="TTTE", "Spacing"=enum."Specified", "Y.start"=-500.0, "Y.end"=500.0, "NumPts"=13.0}]
  in  "Lat.Y-Locations":dbl[](array[numeric])=[-500.0, -400.0, -300.0, -200.0, -100.0, 0.0, 100.0, 200.0, 300.0, 400.0, 500.0]
  in  "Lat.HeightCorrs":T15={"Yvalues"=[0.0, 10.0, 20.0, 30.0, 40.0, 50.0, 60.0, 70.0, 80.0, 90.0, 100.0, 110.0, 120.0, 130.0, 140.0, 150.0, 160.0, 170.0, 180.0, 190.0, 200.0, 210.0, 220.0, 230.0, 240.0, 250.0, 260.0, 270.0, 280.0, 290.0, 300.0, 310.0, 320.0, 330.0, 340.0, 350.0], "X.HeightCorrs"=[[0.0], [-0.4], [-0.4], [-0.1], [0.6], [1.1], [1.5], [1.6], [1.5], [1.1], [0.3], [0.0], [-0.3], [-0.3], [-0.4], [0.7], [0.9], [1.8], [2.4], [2.5], [2.5], [2.2], [1.3], [0.7], [0.4], [0.0], [0.0], [0.8], [1.1], [1.7], [2.4], [2.4], [2.3], [2.3], [1.2], [0.4]], "Use Height Corrections"=FALSE}
  in  "LongProf.Coords":T16(array[cluster])=[{"X0"=-3340.0, "Y"=-500.0, "Z"=229.0, "Name"="Window", "Spacing"=enum."Specified", "X.start"=-3340.0, "X.end"=1475.0, "NumPts"=11.0}, {"X0"=-3340.0, "Y"=0.0, "Z"=229.0, "Name"="MidSpan", "Spacing"=enum."Specified", "X.start"=-3341.0, "X.end"=1476.0, "NumPts"=12.0}, {"X0"=-3340.0, "Y"=500.0, "Z"=229.0, "Name"="Wall", "Spacing"=enum."Specified", "X.start"=-3342.0, "X.end"=1477.0, "NumPts"=13.0}]
  in  "Long.X-Locations":dbl[](array[numeric])=[-500.0, -250.0, 0.0, 250.0, 500.0]
  in  "Long.HeightCorrs":T17={"XValues"=[0.0, 10.0, 20.0, 30.0, 40.0, 50.0, 60.0, 70.0, 80.0, 90.0, 100.0, 110.0, 120.0, 130.0, 140.0, 150.0, 160.0, 170.0, 180.0, 190.0, 200.0, 210.0, 220.0, 230.0, 240.0, 250.0, 260.0, 270.0, 280.0, 290.0, 300.0, 310.0, 320.0, 330.0, 340.0, 350.0], "Y.HeightCorrs"=[[0.0], [-0.4], [-0.4], [-0.1], [0.6], [1.1], [1.5], [1.6], [1.5], [1.1], [0.3], [0.0], [-0.3], [-0.3], [-0.4], [0.7], [0.9], [1.8], [2.4], [2.5], [2.5], [2.2], [1.3], [0.7], [0.4], [0.0], [0.0], [0.8], [1.1], [1.7], [2.4], [2.4], [2.3], [2.3], [1.2], [0.4]], "Use Height Corrections"=FALSE}
  in  "MoveTrav.Coords":T18(array[cluster])=[{"X"=0.0, "Y"=0.0, "Z"=150.0, "Use Tunnel Coords?"=TRUE}]
  in  "MessagesArray":string[](array[string])=["Time to set ramps..."]
  in  "Wait Time (min)":dbl[](array[numeric])=[1440.0]
  out "Audit Array":string[](array[string])=["Initialize", "Initialize Remaining Globals", "Build TT Array", "Warm Up", "Zeroes", "AutoCal", "GlobalCalCheck", "LocalCalCheck", "Turn Table Schedule", "Build-A-Block", "Repeat?", "Zeroes", "AutoCal", "GlobalCalCheck", "LocalCalCheck", "Turn Table Schedule", "Build-A-Block", "Repeat?", "Zeroes", "AutoCal", "GlobalCalCheck", "LocalCalCheck", "Turn Table Schedule", "Build-A-Block", "Repeat?", "Zeroes", "AutoCal", "GlobalCalCheck", "LocalCalCheck", "Turn Table Schedule", "Build-A-Block", "Repeat?", "Zeroes", "AutoCal", "GlobalCalCheck", "LocalCalCheck", "Turn Table Schedule", "Build-A-Block", "Repeat?", "Zeroes", "AutoCal", "GlobalCalCheck", "LocalCalCheck", "Turn Table Schedule", "Build-A-Block", "Repeat?", "Zeroes", "AutoCal", "GlobalCalCheck", "LocalCalCheck", "Turn Table Schedule", "Build-A-Block", "Repeat?", "Zeroes", "AutoCal", "GlobalCalCheck", "LocalCalCheck", "Turn Table Schedule", "Build-A-Block", "Repeat?", "Zeroes", "AutoCal", "GlobalCalCheck", "LocalCalCheck", "Turn Table Schedule", "Build-A-Block", "Repeat?", "Zeroes", "AutoCal", "GlobalCalCheck", "LocalCalCheck", "Turn Table Schedule", "Build-A-Block", "Repeat?", "Zeroes", "AutoCal", "GlobalCalCheck", "LocalCalCheck", "Turn Table Schedule", "Build-A-Block", "Repeat?", "Zeroes", "AutoCal", "GlobalCalCheck", "LocalCalCheck", "Turn Table Schedule", "Build-A-Block", "Repeat?", "Zeroes", "AutoCal", "GlobalCalCheck", "LocalCalCheck", "Turn Table Schedule", "Build-A-Block", "Repeat?", "Zeroes", "AutoCal", "GlobalCalCheck", "LocalCalCheck", "Turn Table Schedule", "Build-A-Block", "Repeat?", "Zeroes", "AutoCal", "GlobalCalCheck", "LocalCalCheck", "Turn Table Schedule", "Build-A-Block", "Repeat?", "Zeroes", "AutoCal", "GlobalCalCheck", "LocalCalCheck", "Turn Table Schedule", "Build-A-Block", "Repeat?", "Zeroes", "AutoCal", "GlobalCalCheck", "LocalCalCheck", "Turn Table Schedule", "Build-A-Block", "Repeat?", "Zeroes", "AutoCal", "GlobalCalCheck", "LocalCalCheck", "Turn Table Schedule", "Build-A-Block", "Repeat?", "End", "Save Multirun?"]
  in  "Index Tracking":T19
  in  "Stop Button":bool
  in  "RowTemplate":T20 {"Carrier_2 Q (l/min)" format="%#.2f"; "Row Duration (mins)" format="%#.1f"; "Row No" min=0; "Trace Gas Concentration (%)" min=0.0 format="%#_4f"; "Carrier_1 Q (l/min)" format="%#.2f"; "Tunnel Speed" format="%#.2f"; "Start X" format="%#.2f"; "Start Y" format="%#.2f"; "Start Z" format="%#.2f"; "End X" format="%#.2f"; "End Y" format="%#.2f"; "End Z" format="%#.2f"; "Averaging time (min)" min=0.0 format="%#.2f"}
  # "X           Y            Z"
  # "Start"
  # "End"
  # "The Build-A-Block feature can be used with or without the TT:Schedule Task Enabled. Use the Row Type Selector in the 1st column to specify the order of tasks in the block. The 2nd column is an index value -- each type of task has a tab control to itself in this interface. In the relevant tab control, you can set up an array of tasks. For instance, you can setup an array of vertical profile tasks, each having different details. Use the index control here to specify which Vertical Profile task [from the array] you would like to call. The 3rd column only applies to profile tasks, and it controls whether a profile is surveyed in the direction given by its setup or in the reverse direction. This can be used to serpentine profiles for efficiency."
  # "X           Y            Z"
  # "Start"
  # "End"
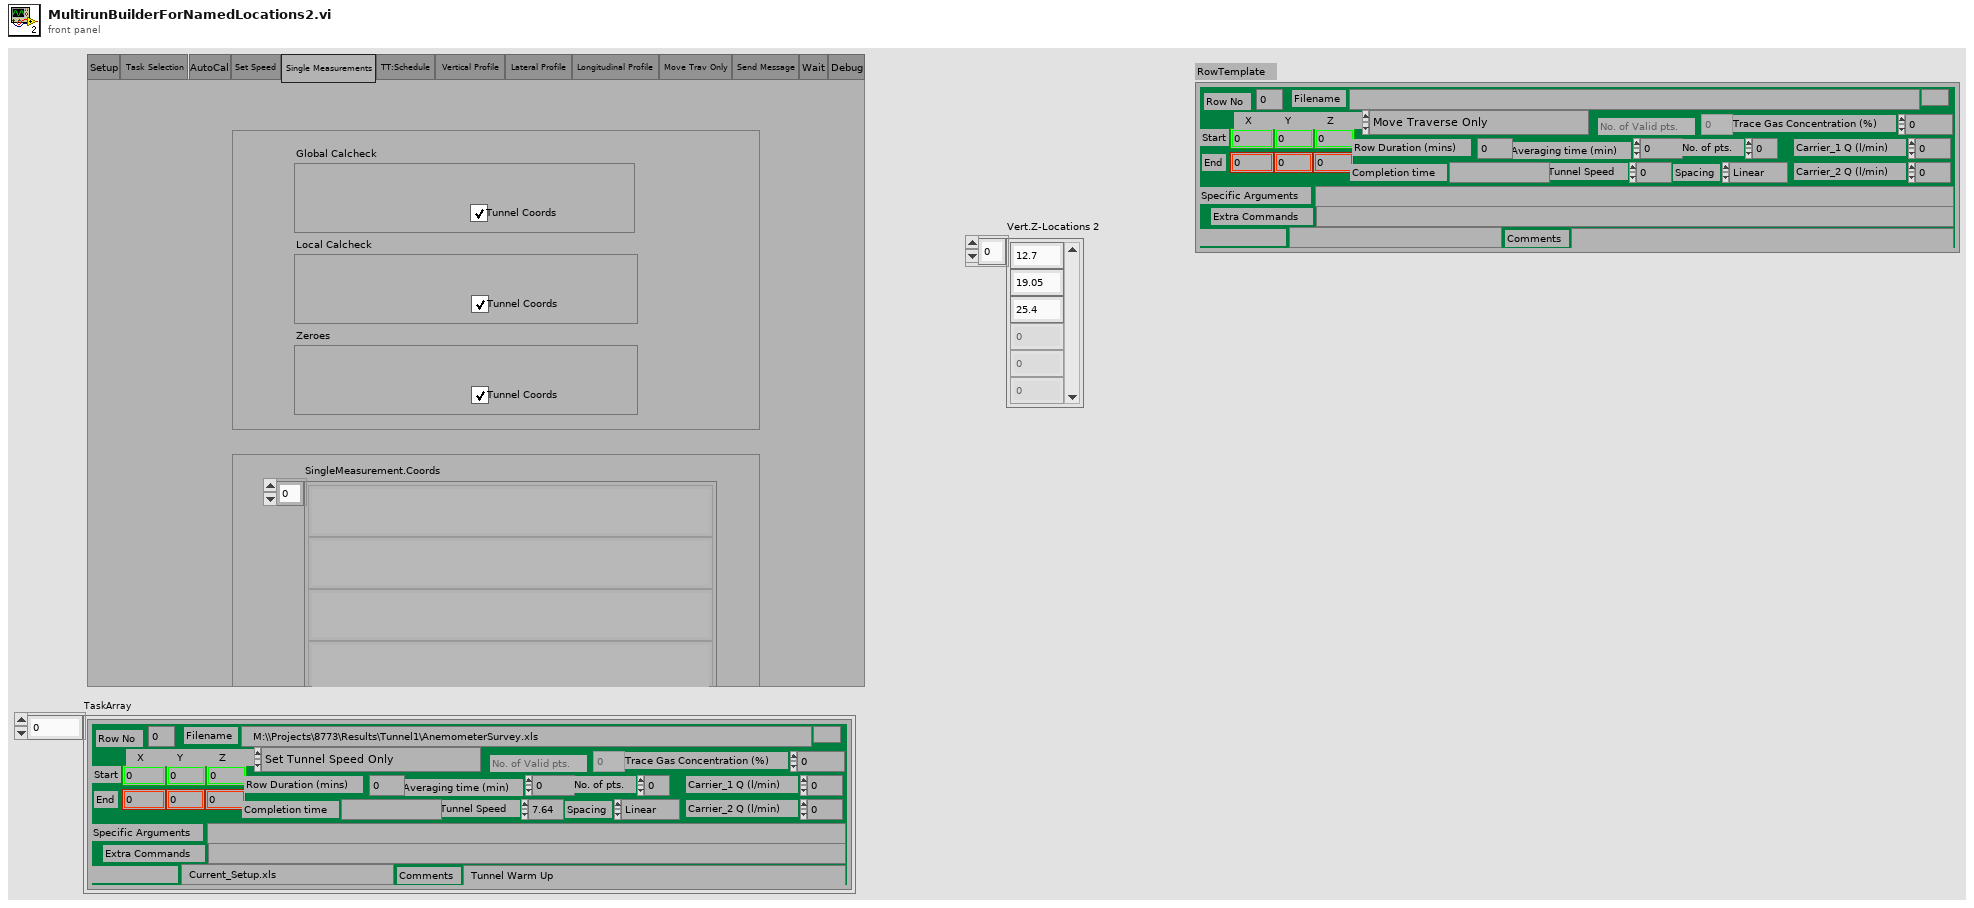
[diagram p1: front panel]
types:
  T1 = typedef "Spacing.ctl" = enum16{"Linear", "Log", "Gauss", "Specified", "N/A"}
  T2 = typedef "Multi_run_mode.ctl" = enum16{"Move Traverse Only", "Set Tunnel Speed Only", "Set Source Only", "Set Measurement Conditions", "Single Measurement", "Vertical Profile", "Lateral Profile", "Longitudinal Profile", "Explore Volume", "Multi-Axis Profile", "Auto Calibrate", "Meas Fast FID Bkgnd", "Check Beam Power", "Scanning Valve Measurement", "Run VI Named:", "Set ADAM Ch", "Wait (minutes)", "Send Message", "Synchronize With:", "Fall Back to this Row", "Turn Off Row Repeating", "Blank Row", "Traverse 3D Volume"}
  T3 = cluster{"Start X":sgl, "Start Y":sgl, "Start Z":sgl, "End X":sgl, "End Y":sgl, "End Z":sgl, "No. of pts.":i32, "Spacing":T1, "Filename":path, "Tunnel Speed":dbl, "Averaging time (min)":dbl, "Extra Commands":string, "Carrier_1 Q (l/min)":dbl, "Carrier_2 Q (l/min)":dbl, "Trace Gas Concentration (%)":dbl, "Specific Arguments":string, "Comments":string, "Row No":i32, "Row Type Selector":T2, "Completion time":string, "Row Duration (mins)":dbl, "No. of Valid pts.":i32, "Meas Setup File":string}[]
  T4 = enum32{"Setup", "Task Selection", "AutoCal", "Set Speed", "Single Measurements", "TT:Schedule", "Vertical Profile", "Lateral Profile", "Longitudinal Profile", "Move Trav Only", "Send Message", "Wait", "Debug"}
  T5 = cluster{"Turn Table --> Zero":bool, "AutoCal":bool, "Zeroes":bool, "Global Cal Checks":bool, "Local Cal Checks":bool, "Tunnel Off":bool}
  T6 = cluster{"Tunnel Warm Up":bool, "AutoCal":bool, "Zeroes":bool, "Turn Table Schedule":bool, "Global Cal Checks":bool, "Local Cal Checks":bool, "Vertical Profile":bool, "Lateral Profile":bool, "Reinitialize Task Array":bool, "Save Command File":bool, "Longitudinal Profile":bool}
  T7 = cluster{"X":dbl, "Y":dbl, "Z":dbl, "Name":string, "Use Tunnel Coords?":bool}[]
  T8 = cluster{"X":dbl, "Y":dbl, "Z":dbl, "Use Tunnel Coords?":bool, "RepeatEveryXDeg":dbl}
  T9 = cluster{"X":dbl, "Y":dbl, "Z":dbl, "Use Tunnel Coords? Coords":bool, "RepeatEveryXDeg":dbl}
  T10 = typedef "MRBRowTaskSelector.ctl" = enum16{"Move Traverse Only", "Set Tunnel Speed Only", "Set Source Only", "Set Measurement Conditions", "Single Measurement", "Vertical Profile", "Lateral Profile", "Longitudinal Profile", "Explore Volume", "Multi-Axis Profile", "Auto Calibrate", "Meas Fast FID Bkgnd", "Check Beam Power", "Scanning Valve Measurement", "Run VI Named:", "MoveTT", "TravZSurvey", "Set ADAM Ch", "Wait (minutes)", "Send Message", "Synchronize With:", "Fall Back to this Row", "Turn Off Row Repeating", "Blank Row", "Traverse 3D Volume"}
  T11 = cluster{"Row Type Selector":T10, "Index":dbl, "Direction":enum16{"Forward", "Reverse"}}[]
  T12 = cluster{"X":dbl, "Y":dbl, "Z0":dbl, "Name":string, "Spacing":enum16{"Linear", "Log", "Gauss", "Specified", "N/A"}, "Z.start":dbl, "Z.end":dbl, "NumPts":dbl}[]
  T13 = cluster{"TT.Azimuths":dbl[], "Z.HeightCorrs":dbl[][], "Use Height Corrections":bool, "Height Survey Filepaths":path[], "Corrections from File":bool}
  T14 = cluster{"X":dbl, "Y0":dbl, "Z":dbl, "Name":string, "Spacing":enum16{"Linear", "Log", "Gauss", "Specified", "N/A"}, "Y.start":dbl, "Y.end":dbl, "NumPts":dbl}[]
  T15 = cluster{"Yvalues":dbl[], "X.HeightCorrs":dbl[][], "Use Height Corrections":bool}
  T16 = cluster{"X0":dbl, "Y":dbl, "Z":dbl, "Name":string, "Spacing":enum16{"Linear", "Log", "Gauss", "Specified", "N/A"}, "X.start":dbl, "X.end":dbl, "NumPts":dbl}[]
  T17 = cluster{"XValues":dbl[], "Y.HeightCorrs":dbl[][], "Use Height Corrections":bool}
  T18 = cluster{"X":dbl, "Y":dbl, "Z":dbl, "Use Tunnel Coords?":bool}[]
  T19 = cluster{"Azimuth Array Index":u32, "Vert Prof Array Index":u32, "Lat Prof Array Index":u32, "Long Prof Array Index":u32}
  T20 = typedef "RowTemplate.ctl" = cluster{"Start X":sgl, "Start Y":sgl, "Start Z":sgl, "End X":sgl, "End Y":sgl, "End Z":sgl, "No. of pts.":i32, "Spacing":T1, "Filename":path, "Tunnel Speed":dbl, "Averaging time (min)":dbl, "Extra Commands":string, "Carrier_1 Q (l/min)":dbl, "Carrier_2 Q (l/min)":dbl, "Trace Gas Concentration (%)":dbl, "Specific Arguments":string, "Comments":string, "Row No":i32, "Row Type Selector":T2, "Completion time":string, "Row Duration (mins)":dbl, "No. of Valid pts.":i32, "Meas Setup File":string}
  T21 = cluster{"Azimuth Array Index":u32, "Vert Prof Array Index":u32, "Lat Prof Array Index":u32, "Azimuth Array Index 2":u32}
  T22 = cluster{"X":dbl, "Y":dbl, "Z":dbl, string, "Use Tunnel Coords?":bool}
  T23 = enum16{"Load Command File", "Save Command File", "Check Multi Run Prog", "Check Multi Run Prog With Live Moves", "Run Multi Run Prog"}
  T24 = typedef "Tunnel_Coordinates.ctl" = enum16{"Work in Tunnel Coordinates", "Work in Model Coordinates"}
  T25 = typedef "Setup_Filetype.ctl" = enum16{"Measurement Setups", "Calibration Setups", "General", "Results File Plotter Setups", "Speed Calib Tweaks"}
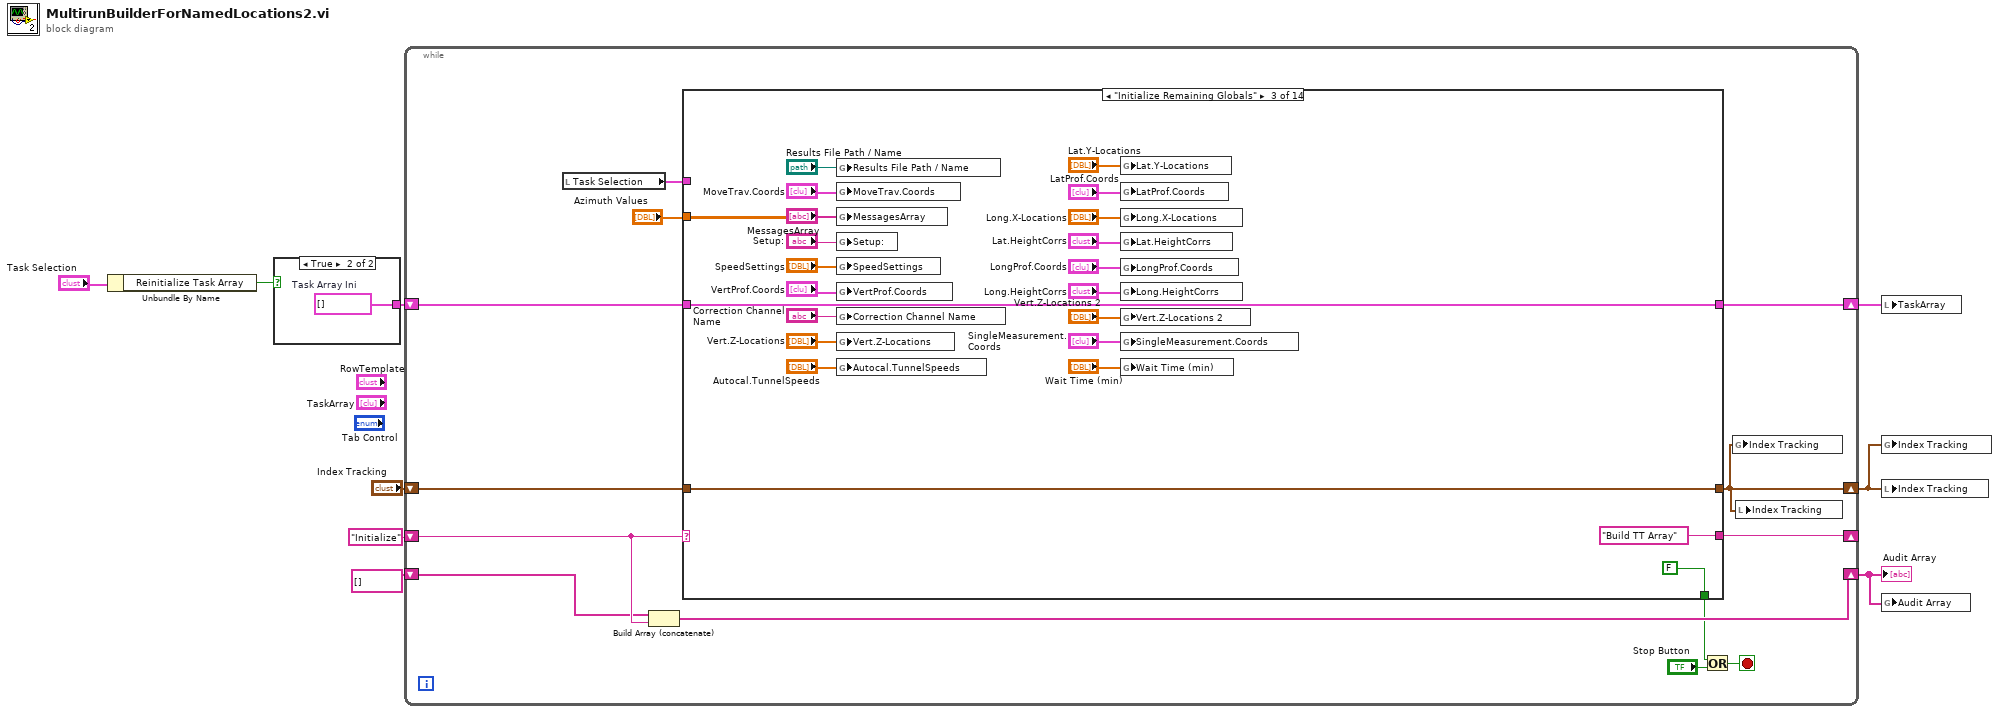
[diagram p0: block diagram]
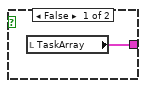
[diagram p2: hidden frame]
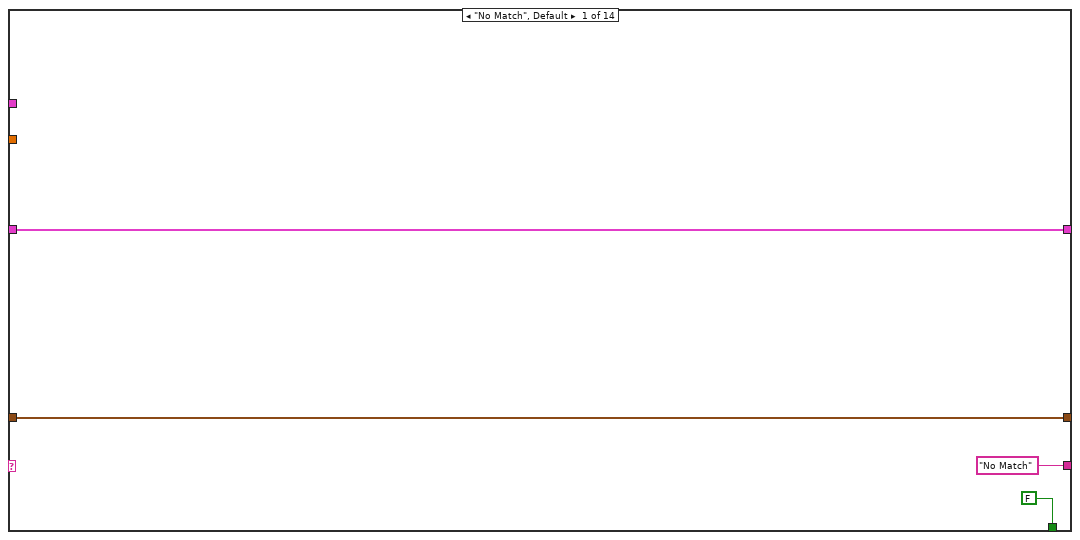
[diagram p3: hidden frame]
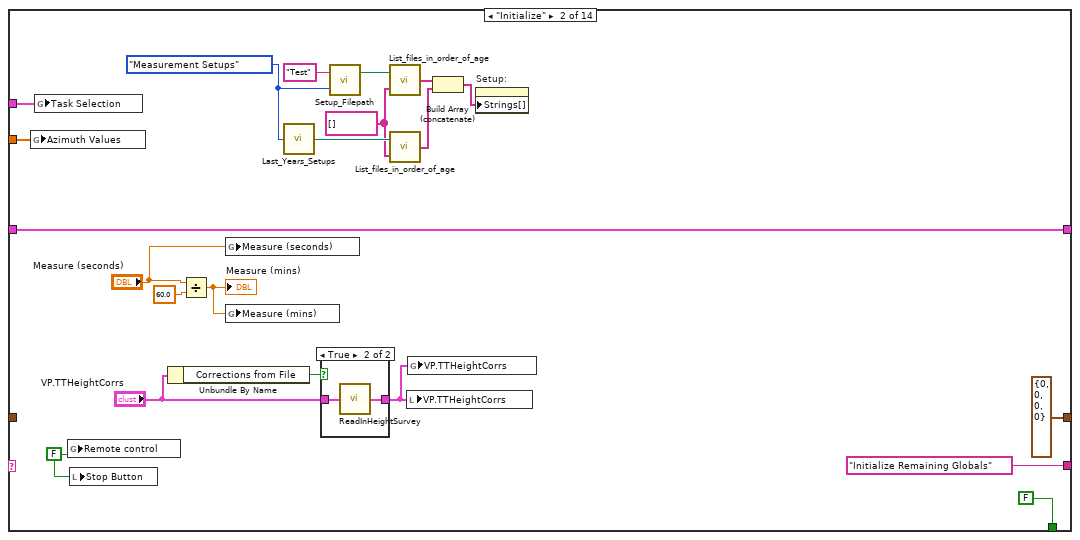
[diagram p4: hidden frame]
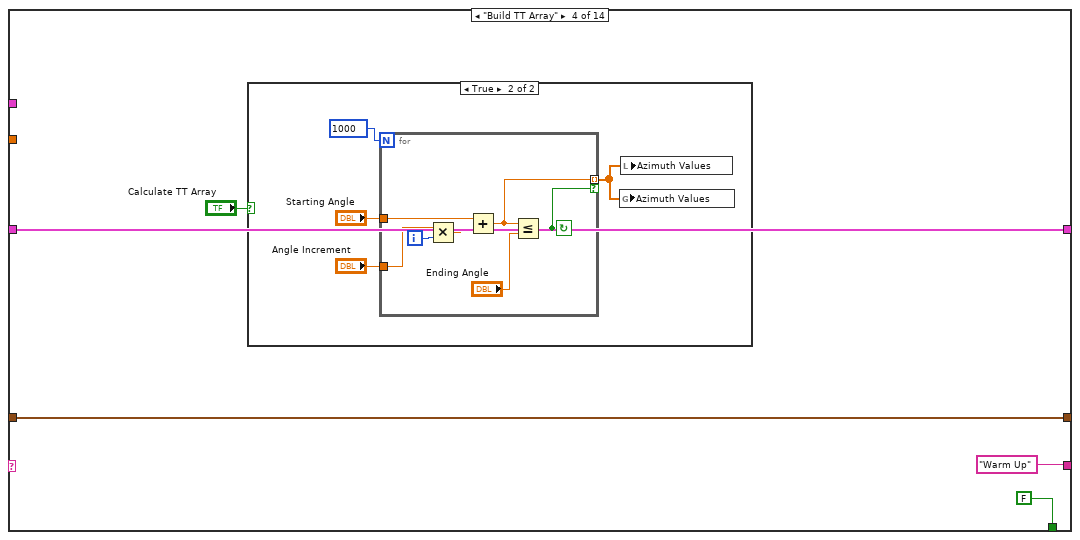
[diagram p6: hidden frame]
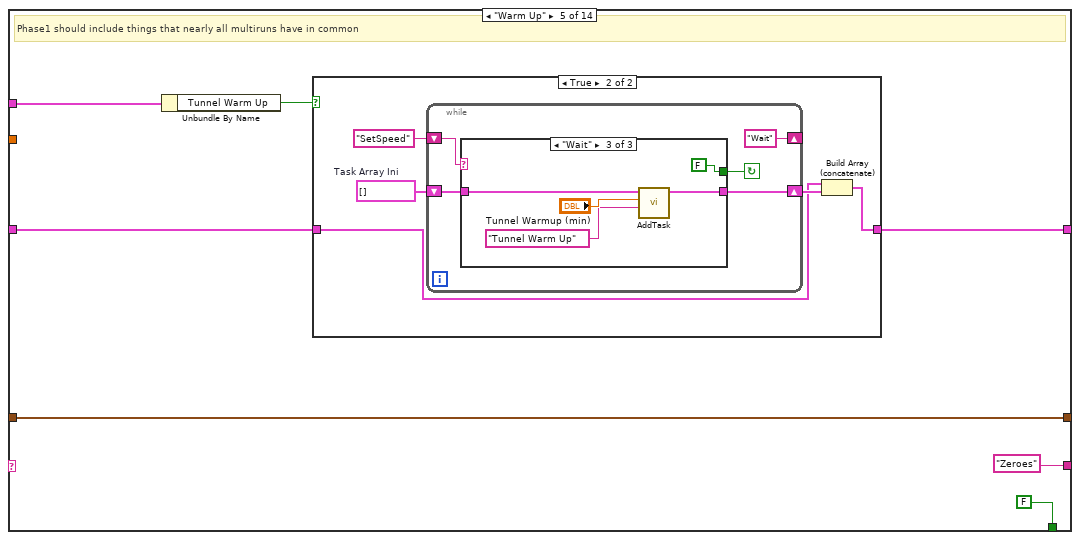
[diagram p8: hidden frame]
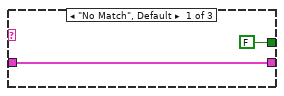
[diagram p10: hidden frame]
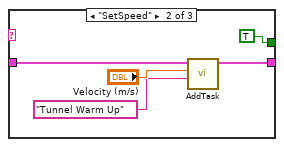
[diagram p11: hidden frame]
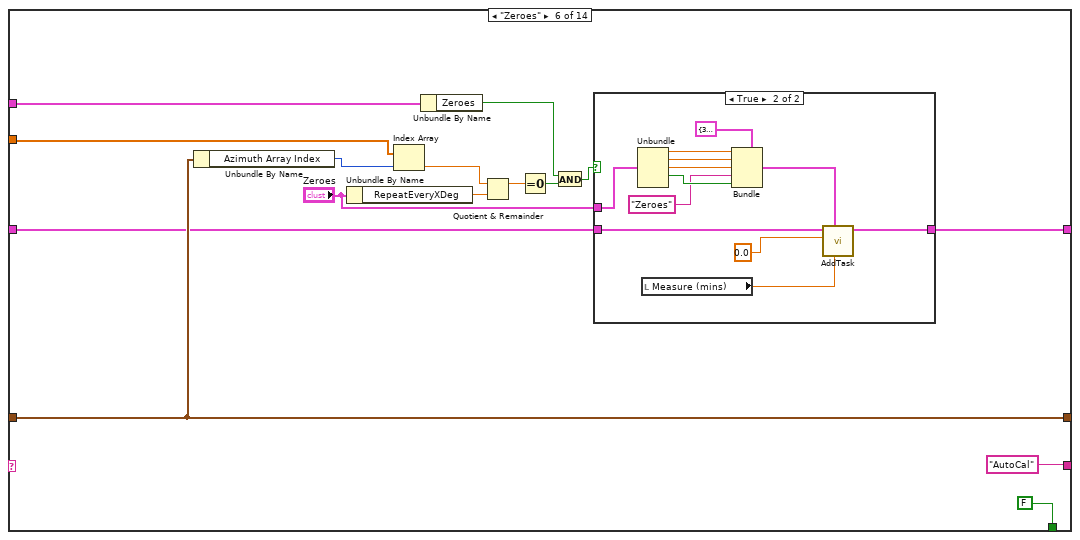
[diagram p12: hidden frame]
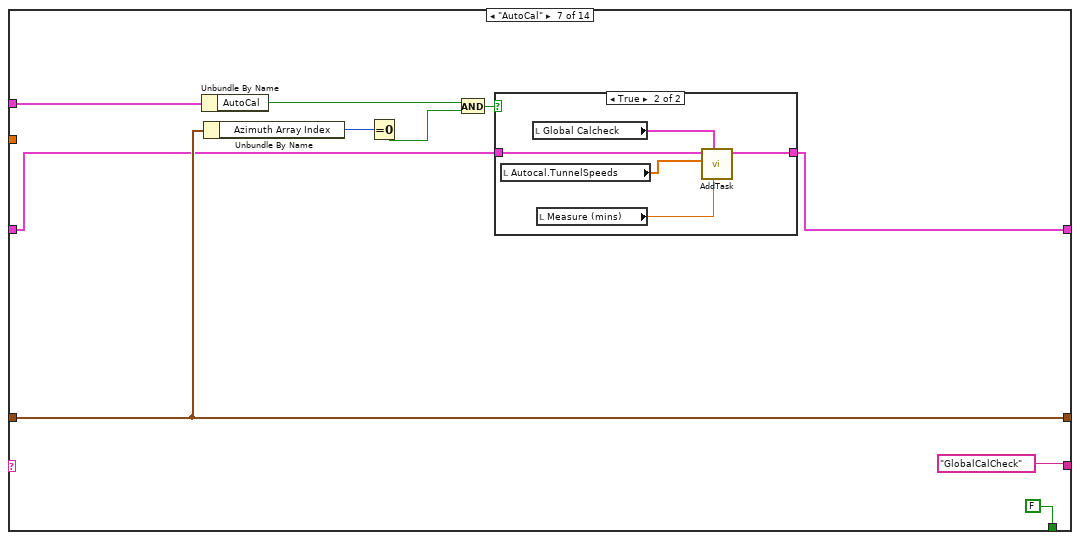
[diagram p14: hidden frame]
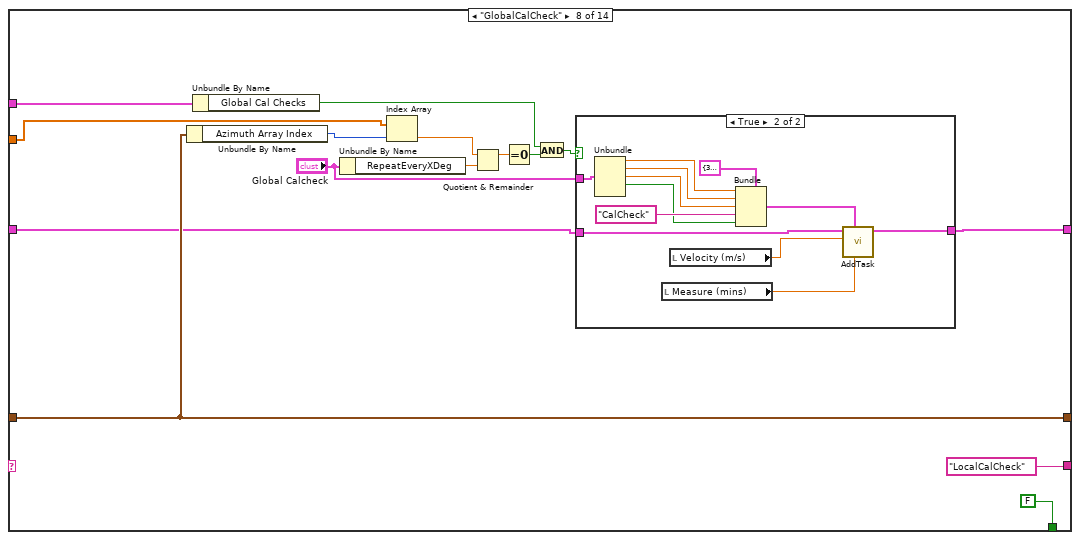
[diagram p16: hidden frame]
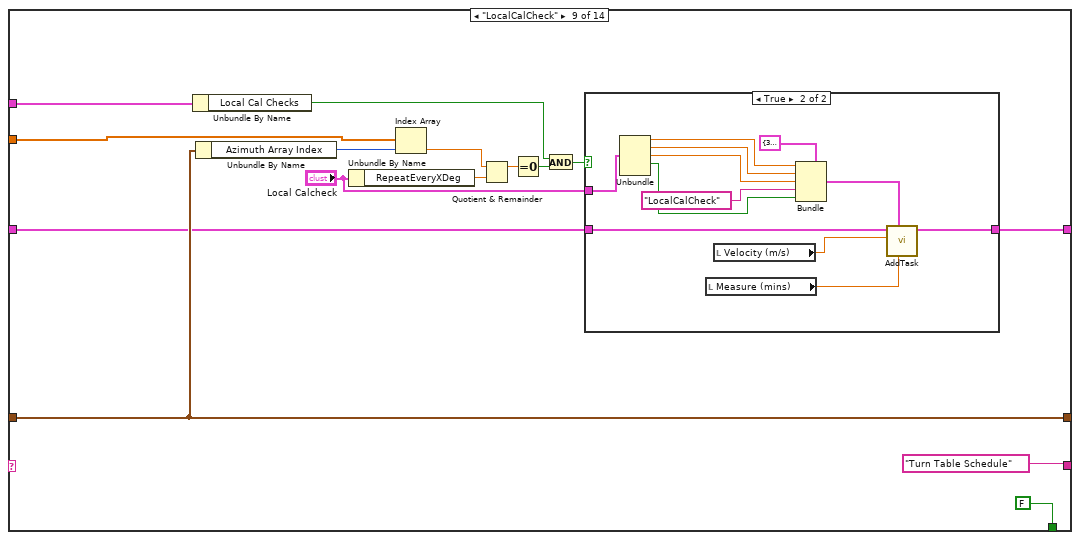
[diagram p18: hidden frame]
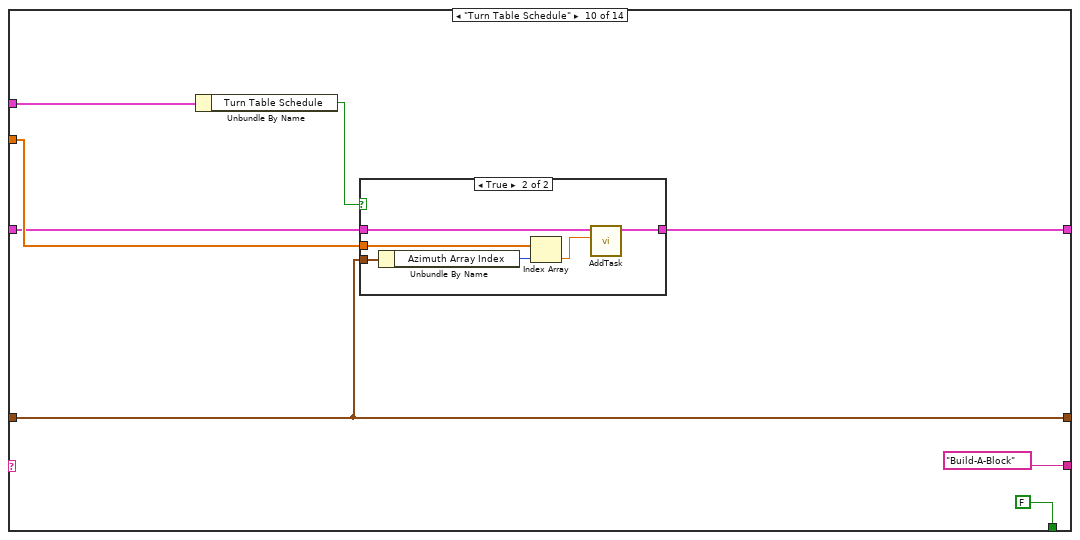
[diagram p20: hidden frame]
diagram:
  n1 = Unbundle By Name("Task Selection") -> ("Reinitialize Task Array"=w6:bool)
  n2 = case shown="True" w6 {
    tunnel: [w10 w11] -> w8
    frame False {
      n3 = local read "TaskArray"() -> (w10:T3)
    }
    frame True {
      w11 = T3 []  # Task Array Ini
    }
  }
  n4 = while {
    shift-right: [w24] -> _
    shift-left: "Initialize" -> [w22]
    shift-right: [w13] -> w1
    shift-left: w8 -> [w14]
    shift-right: [w21] -> w2
    shift-left: string[] [] -> [w20]
    shift-right: [w12] -> w3
    shift-left: "Index Tracking" -> [w23]
    stop <- w17 stop-if-true
    n5 = local read "Task Selection"() -> (w16:T6)
    n6 = Build Array (concatenate)(w20, w22) -> (w21:string[])
    n7 = case shown="\"Initialize Remaining Globals\"" w22 {
      tunnel: ["No Match" "Initialize Remaining Globals" "Build TT Array" "Warm Up" "Zeroes" "AutoCal" "GlobalCalCheck" "LocalCalCheck" "Turn Table Schedule" "Build-A-Block" "Repeat?" w247 "Save Multirun?" ("t") _] -> w24
      tunnel: [FALSE ("Stop Button") FALSE ("Stop Button") FALSE FALSE ("Stop Button") FALSE ("Stop Button") FALSE ("Stop Button") FALSE ("Stop Button") FALSE ("Stop Button") FALSE ("Stop Button") FALSE ("Stop Button") FALSE ("Stop Button") FALSE ("Stop Button") FALSE TRUE] -> w18
      tunnel: "Azimuth Values" -> [_ w35 _ _ _ w133 _ w168 w195 w227 _ w246 _ _]
      tunnel: w23 -> [w26 _ w60 w78 w95 w131 w155 w172 w201 w223 w237 w252 w280 w378]
      tunnel: [w26 T21 {"Azimuth Array Index"=0, "Vert Prof Array Index"=0, "Lat Prof Array Index"=0, "Azimuth Array Index 2"=0} ("Index Tracking") w60 w78 w95 w131 w155 w172 w201 w223 w237 w250 w280 w378] -> w12
      tunnel: w16 -> [_ w34 _ _ w94 w127 w151 w171 w200 w224 _ w243 _ w384]
      tunnel: w14 -> [w25 w36 w59 w75 w92 w121 w149 w165 w194 w222 w239 w244 w270 w381]
      tunnel: [w25 w36 w59 w75 w91 w122 w150 w166 w193 w221 w238 w244 w271 w380] -> w13
      frame "No Match", Default {
      }
      frame "Initialize" {
        w38 = FALSE ("Remote control")
        w48 = Setup_Filetype."Measurement Setups" ("Setup File Type")
        w43 = string[] [] ("file names")
        n8 = global write "MRCMDFBGlobal.vi" "Azimuth Values"(w35) -> ()
        n9 = global write "MRCMDFBGlobal.vi" "Task Selection"(w34) -> ()
        n10 = global write "Meas_global.vi" "Remote control"(w38) -> ()
        n11 = local write "Stop Button"(w38) -> ()
        n12 = Unbundle By Name("VP.TTHeightCorrs") -> ("Corrections from File"=w37:bool)
        n13 = Divide(x="Measure (seconds)", y=60.0 ("x")) -> (x/y=w33:dbl)
        "Measure (mins)" <- w33
        n14 = global write "MRCMDFBGlobal.vi" "Measure (seconds)"("Measure (seconds)") -> ()
        n15 = global write "MRCMDFBGlobal.vi" "Measure (mins)"(w33) -> ()
        n16 = call "Last_Years_Setups.vi"("Setup File Type"=w48) -> ("Directory"=w49:path)
        n17 = case shown="True" w37 {
          tunnel: "VP.TTHeightCorrs" -> [w50 w52]
          tunnel: [w50 w51] -> w30
          frame False {
          }
          frame True {
            n18 = call "ReadInHeightSurvey.vi"("VP.TTHeightCorrs In"=w52) -> ("VP.TTHeightCorrs Out"=w51:T13)
          }
        }
        n19 = call "Setup_Filepath.vi"("Setup File Type"=w48, "Filename in"="Test") -> ("Directory"=w47:path)  [unwired: 1 out]
        n20 = call "List_files_in_order_of_age.vi"("Files to Hide"=w43, "Folder"=w47) -> ("file names"=w46:string[])
        n21 = call "List_files_in_order_of_age.vi"("Files to Hide"=w43, "Folder"=w49) -> ("file names"=w45:string[])
        n22 = local write "VP.TTHeightCorrs"(w30) -> ()
        n23 = global write "MRCMDFBGlobal.vi" "VP.TTHeightCorrs"(w30) -> ()
        n24 = Build Array (concatenate)(w46, w45) -> (w42:string[])
        n25 = property on="Setup:" class="CmbBox"("Strings[]"=w42) -> ()  [unwired: 2 in, 2 out]
      }
      frame "Initialize Remaining Globals" {
        n26 = global write "MRCMDFBGlobal.vi" "Results File Path / Name"("Results File Path / Name") -> ()
        n27 = global write "MRCMDFBGlobal.vi" "MoveTrav.Coords"("MoveTrav.Coords") -> ()
        n28 = global write "MRCMDFBGlobal.vi" "MessagesArray"("MessagesArray") -> ()
        n29 = global write "MRCMDFBGlobal.vi" "Setup:"("Setup:") -> ()
        n30 = global write "MRCMDFBGlobal.vi" "SpeedSettings"("SpeedSettings") -> ()
        n31 = global write "MRCMDFBGlobal.vi" "VertProf.Coords"("VertProf.Coords") -> ()
        n32 = global write "MRCMDFBGlobal.vi" "Correction Channel Name"("Correction Channel Name") -> ()
        n33 = global write "MRCMDFBGlobal.vi" "Vert.Z-Locations"("Vert.Z-Locations") -> ()
        n34 = global write "MRCMDFBGlobal.vi" "Autocal.TunnelSpeeds"("Autocal.TunnelSpeeds") -> ()
        n35 = global write "MRCMDFBGlobal.vi" "Lat.Y-Locations"("Lat.Y-Locations") -> ()
        n36 = global write "MRCMDFBGlobal.vi" "LatProf.Coords"("LatProf.Coords") -> ()
        n37 = global write "MRCMDFBGlobal.vi" "Long.X-Locations"("Long.X-Locations") -> ()
        n38 = global write "MRCMDFBGlobal.vi" "Lat.HeightCorrs"("Lat.HeightCorrs") -> ()
        n39 = global write "MRCMDFBGlobal.vi" "LongProf.Coords"("LongProf.Coords") -> ()
        n40 = global write "MRCMDFBGlobal.vi" "Long.HeightCorrs"("Long.HeightCorrs") -> ()
        n41 = global write "MRCMDFBGlobal.vi" "Vert.Z-Locations 2"("Vert.Z-Locations 2") -> ()
        n42 = global write "MRCMDFBGlobal.vi" "SingleMeasurement.Coords"("SingleMeasurement.Coords") -> ()
        n43 = global write "MRCMDFBGlobal.vi" "Wait Time (min)"("Wait Time (min)") -> ()
      }
      frame "Build TT Array" {
        n44 = case shown="True" "Calculate TT Array" {
          frame False {
          }
          frame True {
            n45 = for {
              N: 1000 -> [_]
              tunnel: "Starting Angle" -> [w88]
              tunnel: "Angle Increment" -> [w89]
              tunnel: [w85] -> w80 mode=indexing if=w84
              i -> [w90]
              stop <- w84 continue-if-true
              n46 = Multiply(x=w89, y=w90) -> (x*y=w87:dbl)
              n47 = Add(x=w88, y=w87) -> (x+y=w85:dbl)
              n48 = Less Or Equal?(x=w85, y="Ending Angle") -> (x <= y?=w84:bool)
            }
            n49 = global write "MRCMDFBGlobal.vi" "Azimuth Values"(w80) -> ()
            n50 = local write "Azimuth Values"(w80) -> ()
          }
        }
      }
      frame "Warm Up" {
        # "Phase1 should include things that nearly all multiruns have in common"
        n51 = Unbundle By Name(w94) -> ("Tunnel Warm Up"=w93:bool)
        n52 = case shown="True" w93 {
          tunnel: w92 -> [w98 w100]
          tunnel: [w98 w99] -> w91
          frame False {
          }
          frame True {
            w102 = T3 []  # Task Array Ini
            n53 = while {
              shift-right: ["Wait"] -> _
              shift-left: "SetSpeed" -> [w108]
              shift-right: [w104] -> w101
              shift-left: w102 -> [w105]
              stop <- w106 continue-if-true
              n54 = case shown="\"Wait\"" w108 {
                tunnel: [FALSE TRUE FALSE] -> w106
                tunnel: w105 -> [w109 w112 w117]
                tunnel: [w109 w111 w116] -> w104
                frame "No Match", Default {
                }
                frame "SetSpeed" {
                  n55 = call-poly "AddTask.vi"("Comments"="Tunnel Warm Up", "Tunnel Speed"="Velocity (m/s)", "Input Task Array"=w112) -> ("Output Task Array"=w111:T20[])  [unwired: 8 in]
                }
                frame "Wait" {
                  n56 = call-poly "AddTask.vi"("Comments"="Tunnel Warm Up", "Wait Time (min)"="Tunnel Warmup (min)", "Input Task Array"=w117) -> ("Output Task Array"=w116:T20[])  [unwired: 8 in]
                }
              }
            }
            n57 = Build Array (concatenate)(w100, w101) -> (w99:T20[])
          }
        }
      }
      frame "Zeroes" {
        n58 = Unbundle By Name(w131) -> ("Azimuth Array Index"=w132:u32)
        n59 = Unbundle By Name("Zeroes") -> ("RepeatEveryXDeg"=w129:dbl)
        n60 = Index Array(array=w133, index=w132) -> (element=w130:dbl)
        n61 = Unbundle By Name(w127) -> ("Zeroes"=w126:bool)
        n62 = Quotient & Remainder(x=w130, y=w129) -> (x-y*floor(x/y)=w128:dbl)  [unwired: 1 out]
        n63 = Equal To 0?(x=w128) -> (x = 0?=w125:bool)
        n64 = And(x=w126, y=w125) -> (x .and. y?=w124:bool)
        n65 = case shown="True" w124 {
          tunnel: "Zeroes" -> [_ w144]
          tunnel: [w136 w146] -> w122
          tunnel: w121 -> [w136 w145]
          frame False {
          }
          frame True {
            n66 = Unbundle(w144) -> ("X"=w142:dbl, "Y"=w141:dbl, "Z"=w140:dbl, "Use Tunnel Coords?"=w138:bool)  [unwired: 1 out]
            n67 = local read "Measure (mins)"() -> (w147:dbl)
            n68 = Bundle(cluster=T22 {"X"=36.0, "Y"=54.0, "Z"=300.0, "", "Use Tunnel Coords?"=TRUE} ("Coordinate Location"), "X"=w142, "Y"=w141, "Z"=w140, "Zeroes" ("Comments"), "Use Tunnel Coords?"=w138) -> (w139:T22)
            n69 = call-poly "AddTask.vi"("Averaging time (min)"=w147, "Coordinate Description"=w139, "Tunnel Speed"=0.0, "Input Task Array"=w145) -> ("Output Task Array"=w146:T20[])  [unwired: 7 in]
          }
        }
      }
      frame "AutoCal" {
        n70 = Unbundle By Name(w151) -> ("AutoCal"=w153:bool)
        n71 = Unbundle By Name(w155) -> ("Azimuth Array Index"=w154:u32)
        n72 = Equal To 0?(x=w154) -> (x = 0?=w156:bool)
        n73 = And(x=w153, y=w156) -> (x .and. y?=w152:bool)
        n74 = case shown="True" w152 {
          tunnel: [w159 w162] -> w150
          tunnel: w149 -> [w159 w161]
          frame False {
          }
          frame True {
            n75 = local read "Autocal.TunnelSpeeds"() -> (w160:dbl[])
            n76 = local read "Global Calcheck"() -> (w163:T8)
            n77 = local read "Measure (mins)"() -> (w164:dbl)
            n78 = call-poly "AddTask.vi"("Averaging time (min)"=w164, "Global Calcheck"=w163, "Autocal.TunnelSpeeds"=w160, "Input Task Array"=w161) -> ("Output Task Array"=w162:T20[])  [unwired: 7 in]
          }
        }
      }
      frame "GlobalCalCheck" {
        n79 = Unbundle By Name(w172) -> ("Azimuth Array Index"=w177:u32)
        n80 = Unbundle By Name(w171) -> ("Global Cal Checks"=w170:bool)
        n81 = Unbundle By Name("Global Calcheck") -> ("RepeatEveryXDeg"=w175:dbl)
        n82 = Index Array(array=w168, index=w177) -> (element=w176:dbl)
        n83 = Quotient & Remainder(x=w176, y=w175) -> (x-y*floor(x/y)=w174:dbl)  [unwired: 1 out]
        n84 = Equal To 0?(x=w174) -> (x = 0?=w173:bool)
        n85 = And(x=w170, y=w173) -> (x .and. y?=w167:bool)
        n86 = case shown="True" w167 {
          tunnel: "Global Calcheck" -> [_ w188]
          tunnel: [w180 w190] -> w166
          tunnel: w165 -> [w180 w189]
          frame False {
          }
          frame True {
            n87 = Unbundle(w188) -> ("X"=w185:dbl, "Y"=w184:dbl, "Z"=w183:dbl, "Use Tunnel Coords?"=w182:bool)  [unwired: 1 out]
            n88 = local read "Measure (mins)"() -> (w191:dbl)
            n89 = local read "Velocity (m/s)"() -> (w192:dbl)
            n90 = Bundle(cluster=T22 {"X"=36.0, "Y"=54.0, "Z"=300.0, "", "Use Tunnel Coords?"=TRUE} ("Coordinate Location"), "X"=w185, "Y"=w184, "Z"=w183, "CalCheck" ("Comments"), "Use Tunnel Coords?"=w182) -> (w181:T22)
            n91 = call-poly "AddTask.vi"("Averaging time (min)"=w191, "Coordinate Description"=w181, "Tunnel Speed"=w192, "Input Task Array"=w189) -> ("Output Task Array"=w190:T20[])  [unwired: 7 in]
          }
        }
      }
      frame "LocalCalCheck" {
        n92 = Unbundle By Name(w200) -> ("Local Cal Checks"=w199:bool)
        n93 = Unbundle By Name(w201) -> ("Azimuth Array Index"=w205:u32)
        n94 = Unbundle By Name("Local Calcheck") -> ("RepeatEveryXDeg"=w203:dbl)
        n95 = Index Array(array=w195, index=w205) -> (element=w204:dbl)
        n96 = Quotient & Remainder(x=w204, y=w203) -> (x-y*floor(x/y)=w202:dbl)  [unwired: 1 out]
        n97 = Equal To 0?(x=w202) -> (x = 0?=w198:bool)
        n98 = And(x=w199, y=w198) -> (x .and. y?=w197:bool)
        n99 = case shown="True" w197 {
          tunnel: "Local Calcheck" -> [_ w216]
          tunnel: w194 -> [w208 w218]
          tunnel: [w208 w217] -> w193
          frame False {
          }
          frame True {
            n100 = Unbundle(w216) -> ("X"=w209:dbl, "Y"=w210:dbl, "Z"=w211:dbl, "Use Tunnel Coords? Coords"=w212:bool)  [unwired: 1 out]
            n101 = local read "Measure (mins)"() -> (w219:dbl)
            n102 = local read "Velocity (m/s)"() -> (w220:dbl)
            n103 = Bundle(cluster=T22 {"X"=36.0, "Y"=54.0, "Z"=300.0, "", "Use Tunnel Coords?"=TRUE} ("Coordinate Location"), "X"=w209, "Y"=w210, "Z"=w211, "LocalCalCheck" ("Comments"), "Use Tunnel Coords?"=w212) -> (w213:T22)
            n104 = call-poly "AddTask.vi"("Averaging time (min)"=w219, "Coordinate Description"=w213, "Tunnel Speed"=w220, "Input Task Array"=w218) -> ("Output Task Array"=w217:T20[])  [unwired: 7 in]
          }
        }
      }
      frame "Turn Table Schedule" {
        n105 = Unbundle By Name(w224) -> ("Turn Table Schedule"=w225:bool)
        n106 = case shown="True" w225 {
          tunnel: w227 -> [_ w235]
          tunnel: w223 -> [_ w234]
          tunnel: w222 -> [w229 w233]
          tunnel: [w229 w232] -> w221
          frame False {
          }
          frame True {
            n107 = Unbundle By Name(w234) -> ("Azimuth Array Index"=w231:u32)
            n108 = Index Array(array=w235, index=w231) -> (element=w230:dbl)
            n109 = call-poly "AddTask.vi"("TT:Azimuth"=w230, "Input Task Array"=w233) -> ("Output Task Array"=w232:T20[])  [unwired: 9 in]
          }
        }
      }
      frame "Build-A-Block" {
        n110 = call "MR_Build-A-Block.vi"("Build-A-Block"="Build-A-Block") -> ("TaskArray"=w240:T3)
        n111 = Build Array (concatenate)(w239, w240) -> (w238:T20[])
      }
      frame "Repeat?" {
        # "Only reason to repeat is if TT Scheduling"
        n112 = Unbundle By Name(w243) -> ("Turn Table Schedule"=w245:bool)
        n113 = case shown="True" w245 {
          tunnel: w252 -> [w254 w261]
          tunnel: [TRUE w260] -> w251
          tunnel: [w254 w259] -> w250
          tunnel: w246 -> [_ w258]
          frame False {
          }
          frame True {
            n114 = Array Size(array=w258) -> (size(s)=w257:i32)
            n115 = Decrement(x=w257) -> (x-1=w256:i32)
            n116 = in-place {
              in-place-border: w256 -> [w263]
              in-place-border: [w264] -> w260
              n117 = in-place-cluster #1(w261) -> ("Azimuth Array Index"=w262:u32)
              n118 = Equal?(x=w263, y=w262) -> (x = y?=w264:bool)
              n119 = case shown="True" w264 {
                tunnel: [w266 0] -> w265
                tunnel: w262 -> [w267 _]
                frame False {
                  n120 = Increment(x=w267) -> (x+1=w266:u32)
                }
                frame True {
                }
              }
              n121 = in-place-cluster #1("Azimuth Array Index"=w265) -> (w259:T19)
            }
          }
        }
        n122 = Select(t="End", s=w251, f="Zeroes" ("t")) -> (s? t:f=w247:string)
      }
      frame "End" {
        n123 = Unbundle By Name("Multirun Closure Tasks") -> ("Turn Table --> Zero"=w277:bool, "Zeroes"=w276:bool, "AutoCal"=w275:bool, "Global Cal Checks"=w274:bool, "Local Cal Checks"=w273:bool, "Tunnel Off"=w272:bool)
        n124 = while {
          shift-right: [w291] -> _
          shift-left: "Turn Table" -> [w292]
          tunnel: w277 -> [w290]
          tunnel: w276 -> [w287]
          tunnel: w275 -> [w286]
          tunnel: w274 -> [w285]
          tunnel: w273 -> [w284]
          tunnel: w272 -> [w283]
          shift-right: [w288] -> w271
          shift-left: w270 -> [w289]
          stop <- w282 continue-if-true
          n125 = case shown="\"Tunnel Off\"" w292 {
            tunnel: [_ "Zeroes" "AutoCal" "GlobalCalCheck" "LocalCalCheck" "Tunnel Off" _] -> w291
            tunnel: w290 -> [_ w299 _ _ _ _ _]
            tunnel: w289 -> [w294 w298 w308 w326 w337 w355 w372]
            tunnel: [w294 w297 w307 w325 w336 w354 w371] -> w288
            tunnel: w287 -> [_ _ w304 _ _ _ _]
            tunnel: w286 -> [_ _ _ w322 _ _ _]
            tunnel: w285 -> [_ _ _ _ w334 _ _]
            tunnel: w284 -> [_ _ _ _ _ w352 _]
            tunnel: w283 -> [_ _ _ _ _ _ w370]
            tunnel: [FALSE TRUE TRUE TRUE TRUE TRUE TRUE] -> w282
            frame "No Match", Default {
            }
            frame "Turn Table" {
              n126 = case shown="True" w299 {
                tunnel: w298 -> [w300 w302]
                tunnel: [w300 w301] -> w297
                frame False {
                }
                frame True {
                  n127 = call-poly "AddTask.vi"("TT:Azimuth"=0.0, "Input Task Array"=w302) -> ("Output Task Array"=w301:T20[])  [unwired: 9 in]
                }
              }
            }
            frame "Zeroes" {
              n128 = case shown="True" w304 {
                tunnel: w308 -> [w309 w320]
                tunnel: [w309 w319] -> w307
                frame False {
                }
                frame True {
                  n129 = local read "Zeroes"() -> (w317:T8)
                  n130 = Unbundle(w317) -> ("X"=w314:dbl, "Y"=w313:dbl, "Z"=w312:dbl, "Use Tunnel Coords?"=w311:bool)  [unwired: 1 out]
                  n131 = local read "Measure (mins)"() -> (w318:dbl)
                  n132 = Bundle(cluster=T22 {"X"=36.0, "Y"=54.0, "Z"=300.0, "", "Use Tunnel Coords?"=TRUE} ("Coordinate Location"), "X"=w314, "Y"=w313, "Z"=w312, "Zeroes" ("Comments"), "Use Tunnel Coords?"=w311) -> (w310:T22)
                  n133 = call-poly "AddTask.vi"("Averaging time (min)"=w318, "Coordinate Description"=w310, "Tunnel Speed"=0.0, "Input Task Array"=w320) -> ("Output Task Array"=w319:T20[])  [unwired: 7 in]
                }
              }
            }
            frame "AutoCal" {
              n134 = case shown="True" w322 {
                tunnel: w326 -> [w327 w332]
                tunnel: [w327 w331] -> w325
                frame False {
                }
                frame True {
                  n135 = local read "Autocal.TunnelSpeeds"() -> (w328:dbl[])
                  n136 = local read "Global Calcheck"() -> (w329:T8)
                  n137 = local read "Measure (mins)"() -> (w330:dbl)
                  n138 = call-poly "AddTask.vi"("Averaging time (min)"=w330, "Global Calcheck"=w329, "Autocal.TunnelSpeeds"=w328, "Input Task Array"=w332) -> ("Output Task Array"=w331:T20[])  [unwired: 7 in]
                }
              }
            }
            frame "GlobalCalCheck" {
              n139 = case shown="True" w334 {
                tunnel: w337 -> [w338 w350]
                tunnel: [w338 w347] -> w336
                frame False {
                }
                frame True {
                  n140 = local read "Global Calcheck"() -> (w346:T8)
                  n141 = Unbundle(w346) -> ("X"=w342:dbl, "Y"=w341:dbl, "Z"=w340:dbl, "Use Tunnel Coords?"=w339:bool)  [unwired: 1 out]
                  n142 = local read "Measure (mins)"() -> (w348:dbl)
                  n143 = local read "Velocity (m/s)"() -> (w349:dbl)
                  n144 = Bundle(cluster=T22 {"X"=36.0, "Y"=54.0, "Z"=300.0, "", "Use Tunnel Coords?"=TRUE} ("Coordinate Location"), "X"=w342, "Y"=w341, "Z"=w340, "CalCheck" ("Comments"), "Use Tunnel Coords?"=w339) -> (w343:T22)
                  n145 = call-poly "AddTask.vi"("Averaging time (min)"=w348, "Coordinate Description"=w343, "Tunnel Speed"=w349, "Input Task Array"=w350) -> ("Output Task Array"=w347:T20[])  [unwired: 7 in]
                }
              }
            }
            frame "LocalCalCheck" {
              n146 = case shown="True" w352 {
                tunnel: w355 -> [w356 w367]
                tunnel: [w356 w366] -> w354
                frame False {
                }
                frame True {
                  n147 = local read "Local Calcheck"() -> (w364:T9)
                  n148 = Unbundle(w364) -> ("X"=w362:dbl, "Y"=w361:dbl, "Z"=w360:dbl, "Use Tunnel Coords? Coords"=w357:bool)  [unwired: 1 out]
                  n149 = local read "Measure (mins)"() -> (w365:dbl)
                  n150 = local read "Velocity (m/s)"() -> (w368:dbl)
                  n151 = Bundle(cluster=T22 {"X"=36.0, "Y"=54.0, "Z"=300.0, "", "Use Tunnel Coords?"=TRUE} ("Coordinate Location"), "X"=w362, "Y"=w361, "Z"=w360, "LocalCalCheck" ("Comments"), "Use Tunnel Coords?"=w357) -> (w358:T22)
                  n152 = call-poly "AddTask.vi"("Averaging time (min)"=w365, "Coordinate Description"=w358, "Tunnel Speed"=w368, "Input Task Array"=w367) -> ("Output Task Array"=w366:T20[])  [unwired: 7 in]
                }
              }
            }
            frame "Tunnel Off" {
              n153 = case shown="True" w370 {
                tunnel: w372 -> [w373 w375]
                tunnel: [w373 w374] -> w371
                frame False {
                }
                frame True {
                  n154 = call-poly "AddTask.vi"("Comments"="Tunnel Off", "Tunnel Speed"=0.0, "Input Task Array"=w375) -> ("Output Task Array"=w374:T20[])  [unwired: 8 in]
                }
              }
            }
          }
        }
      }
      frame "Save Multirun?" {
        n155 = Unbundle By Name(w384) -> ("Save Command File"=w382:bool)
        n156 = case shown="True" w382 {
          tunnel: "Command File Path / Name" -> [_ w391]
          tunnel: w381 -> [w385 w386]
          tunnel: [w385 w386] -> w380
          frame False {
          }
          frame True {
            n157 = case shown="False" "Work in TUNNEL Coordinates" {
              tunnel: [Tunnel_Coordinates."Work in Model Coordinates" ("Work in Tunnel Coordinates?") Tunnel_Coordinates."Work in Tunnel Coordinates" ("Work in Tunnel Coordinates?")] -> w388
              frame False {
              }
              frame True {
              }
            }
            n158 = call "Multi_Run_Prog.vi"("Command filename"=w391, "Mode"=T23."Save Command File", "Table"=w386, "Work in Tunnel Coordinates?"=w388, "Jump Bad Positions"="Jump Bad Positions") -> ()  [unwired: 14 in, 1 out]
          }
        }
      }
    }
    n159 = Or(x=w18, y="Stop Button") -> (x .or. y?=w17:bool)
    n160 = global write "MRCMDFBGlobal.vi" "Index Tracking"(w12) -> ()
    n161 = local write "Index Tracking"(w12) -> ()
  }
  "Audit Array" <- w2
  n162 = local write "TaskArray"(w1) -> ()
  n163 = global write "MRCMDFBGlobal.vi" "Index Tracking"(w3) -> ()
  n164 = local write "Index Tracking"(w3) -> ()
  n165 = global write "MRCMDFBGlobal.vi" "Audit Array"(w2) -> ()
